vi "Main.vi"() -> ()   [LabVIEW 2024]
doc: "Main Program initialize config files, handles user inputs, image acquisition, object detection and image storing. User interface is handled in a state machine sending outputs."
uses:
  controls/Data_JKI.ctl
  <vilib>/userDefined/High Color/IMAQdx.ctl
  <vilib>/vision/Image Controls.llb/IMAQ Image.ctl
  CAM_ID.ctl
  <vilib>/vision/driver/IMAQdx.llb/IMAQdx Camera Control Mode.ctl
  <vilib>/addons/_JKI Toolkits/State Machine/_JKI_lib_State_Machine.llb/Select State(s)_bool__jki_lib_state_machine.vi
  <vilib>/addons/_JKI Toolkits/State Machine/_JKI_lib_State_Machine.llb/Select State(s)_err__jki_lib_state_machine.vi
  5a594196-7142-418f-9656-114c0d668309.vi
  bb2d0c64-4a32-4bc2-b703-4003a0b41c3e.vi
  382dfe38-6e62-4a8f-90ef-71572aba4852.vi
  03aece60-1779-4009-a170-6ff07e738b5d.vi
  84b06488-54b1-401d-9401-24ea6e13162c.vi
  8324a88f-2dce-41de-b56a-eb000cd9b6a9.vi
  af50b9d5-4c90-4cd4-8bfe-74b4777be0cf.vi
  75fb93f5-a9aa-4c6b-93c7-07fbec5219cd.vi
  9cdd72f1-8236-455d-ab5e-5837bd52b41e.vi
  99c214c5-2fde-429c-805f-c7e6bab6585a.vi
  c28b30e7-2201-423e-8025-b3bde2d8c85a.vi
  557f3c17-7900-4f14-af8c-d1828dceced0.vi
  f995d3e5-f405-4ab5-a577-27e0de2fc963.vi
  fac71c25-9fc9-4a64-ae82-7863fefb1b13.vi
  4f10c793-c4d5-419f-bcb1-2d0c9d14968a.vi
  05f65ac7-837b-4982-8062-8738a5ade4f2.vi
  3f6d6c7d-6f0a-4ecb-ada9-c2a4a5f01e8e.vi
  <extravilib>/ChannelInstances/Tag-t'Data_JKI.ctl'/Read With Abort.vi
  <extravilib>/ChannelInstances/Tag-c(bool,bool)/Write With Abort.vi
  <extravilib>/ChannelInstances/Tag-c(bool,bool)/Read With Abort.vi
  <extravilib>/ChannelInstances/Tag-t'Data_JKI.ctl'/Write With Abort.vi
  <extravilib>/ChannelInstances/Tag-t'Data_JKI.ctl'/Instantiate.vi
  <extravilib>/ChannelInstances/Tag-t'Data_JKI.ctl'/EndpointRead.vi
  <vilib>/addons/_JKI Toolkits/State Machine/_JKI_lib_State_Machine.llb/Periodic Trigger__ogtk__JKI-SM__jki_lib_state_machine.vi
  <vilib>/Utility/xml.llb/Read From XML File(string).vi
  <vilib>/Utility/xml.llb/Write to XML File(string).vi
  <extravilib>/ChannelInstances/Tag-t'Data_JKI.ctl'/Endpoint.vi
  <extravilib>/ChannelInstances/Tag-c(bool,bool)/Instantiate.vi
  <extravilib>/ChannelInstances/Tag-c(bool,bool)/EndpointRead.vi
  <extravilib>/ChannelInstances/Tag-c(bool,bool)/Endpoint.vi
  <vilib>/regexp/Match Regular Expression.xnode
  <extravilib>/ChannelInstances/Tag-c(bool,bool).lvlib
  <vilib>/vision/driver/NI_Vision_Acquisition_Software.lvlib
  <extravilib>/ChannelInstances/Tag-t'Data_JKI.ctl'.lvlib
panel:
  out "Phase 3":bool
  out "Valve":bool
  out "Pump":bool
  out "Cam 1":bool
  out "Cam 2":bool
  out "Status":string
  in  "Auto Flush":bool
  in  "Empty and Refill":bool
  in  "Close and Refill":bool
  out "read buffer 2":string
  out "System Version":string="SRS Software - Version 0.0.0.1-beta"
  in  "Other notes":string caption="Sample Name"
  in  "Species Name":string="Test Sample" caption="Sample Name"
  out "Ready":bool=TRUE
  in  "Operator":string="JFR" caption="Sample Name"
  out "Active":bool
  in  "Start Image Capture":bool
  in  "Sample Name":string="#00000"
  in  "Stop Image Capture":bool
  out "Overlay_tab":T1(tab)=enum."Phase3"
  in  "Overload threshold":i32=50 min=1
  in  "Img Save Que Size":i32=100 caption="Save Buffer Size" min=1
  in  "Img Proc Que Size":i32=200 caption="Process Buffer Sze" min=1
  in  "Reconnect Cams":bool
  in  "Reconnect Arduino mega":bool
  in  "Reconnect Pump":bool
  in  "Reconnect Arduino Uno":bool
  in  "Connect Systems":bool
  out "Cam1_Stats":cluster{"Mean_Area":i32, "Img_Count":u32} caption="Camera 1"
  out "Cam2_Stats":cluster{"Mean_Area":i32, "Img_Count":u32} caption="Camera 2"
  out "Sample Number":string="#0000" caption="Sample Name"
  out "Container barcode":string
  out "Container num. Out":i32
  out "Individual processed":bool
  in  "Collection Date":timestamp=timestamp(2713993200 s since 1904-01-01) format="%<%x>T"
  in  "Station":string="Station..." caption="Sample Name"
  in  "Location":string="Location..." caption="Sample Name"
  in  "Latitude":string="56.149375" caption="Sample Name"
  in  "Longitude":string="10.212404" caption="Sample Name"
  in  "Determiner":string="Name..." caption="Sample Name"
  in  "Sex":string="NaN" caption="Sample Name"
  in  "LegCamAtt":bool caption="Legacy Camera Attributes"
  in  "Change Crop":bool
  in  "DetectCrop":dbl=30.0 caption="Movement Detection size" format="%#_g %"
  in  "Sample size threshold":i32=500 min=1
  in  "New Sample timeout":i32=20 min=1
  in  "Calibration Pictures":bool
  out "Target framerate":i32=5 caption="Target FPS"
  in  "Max Framerate":i32=5 caption="Max FPS" min=1
  in  "Exposure Time":dbl=2000.0
  in  "Exposure":enum32{"Item 0", "Item 1", "Item 2", "Item 3"}(radio)=enum."Item 3"
  in  "Aperture":enum32{"Item 0", "Item 1", "Item 2", "Item 3"}(radio)=enum."Item 2"
  in  "I":i32(slide)=1 min=1 max=9 step=1 scale=1.0..9.0
  in  "A":dbl(slide) min=0.0 max=6000.0 step=100.0 scale=0.0..6000.0
  in  "Send CMD":bool
  in  "Pump Cycle":bool
  in  "Manual Open":bool
  in  "Open & Close":bool
  in  "Manual Close":bool
  out "Current Position":string
  in  "Position":bool
  in  "Apply sorting val":bool
  in  "Initial size":dbl min=0.0
  in  "Num. of containers":dbl=30.0 min=1.0 max=30.0
  in  "Size Interval":dbl=100.0 min=1.0
  in  "Sorting sys.":bool
  in  "Clear Error":bool
  in  "Rescan barcodes":bool
  in  "Send Barcode":bool
  in  "Return Home":bool
  in  "Get Barcode list":bool
  in  "Get Status":bool
  in  "Container nr.":dbl=30.0 min=1.0 max=30.0
  out "Process buffer":T2(graph)
  out "Save buffer":T2(graph)
  out "Framerate":i32 caption="Current Framerate"
  out "Status History":string
  in  "Save History":bool
  in  "Overlay_Ring":u16(ring)=5 items=["System", "Session Data", "Extended Setup", "Camera", "Dispenser", "Phase3", "Stats", "History"]
  in  "Exit":bool
  out "Camera 1":T3(plugin-control)
  out "Camera 2":T3(plugin-control)
  out "Camera 1 Binary":T3(plugin-control)
  out "Camera 2 Binary":T3(plugin-control)
  out "Camera 1 Detect":T3(plugin-control)
  out "Camera 2 Detect":T3(plugin-control)
  # "Connections"
  # "Description:\nData from the last sample for each camera.\n\nMean area\nMean area  from detection algorithm.\n\nImages\nTotal number of images saved."
  # "Barcode and container"
  # "Detection settings"
  # "Camera/Lens settings"
  # "Pump Control"
  # "Hatch Control"
  # "A0-6000 Plunger position\nI1-9 Valve port [CW]"
  # "Automatic Functions"
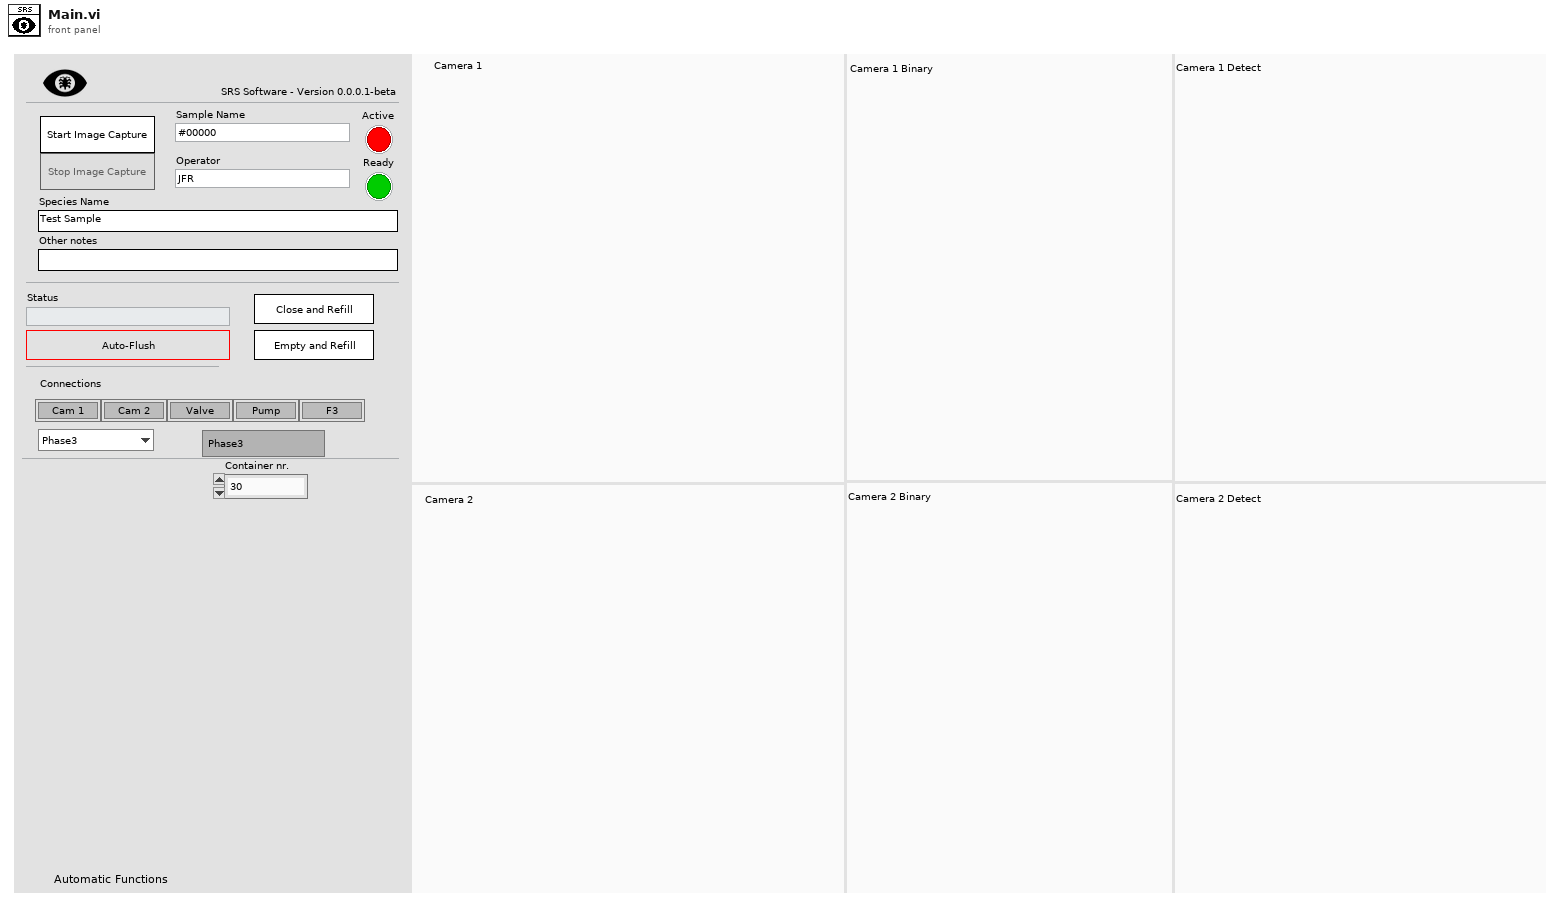
[diagram p1: front panel]
types:
  T1 = enum32{"System", "Session Data", "Extended Setup", "Camera", "Dispenser", "Phase3", "Stats", "History"}
  T2 = cluster{"# elements in queue":i32, "# elements in queue":i32}
  T3 = typedef "IMAQ Image.ctl" = refnum<image>
  T4 = typedef "Data_JKI.ctl" = cluster{"Camera 1":cluster{"Camera1":T5, "Cam 1":bool, "CAM1 Model":enum16{"a2A5328-15ucBAS", "acA1920-155uc"}, "Cam1 ID":i32}, "Camera 2":cluster{"Camera2":T5, "Cam 2":bool, "CAM2 Model":enum16{"a2A5328-15ucBAS", "acA1920-155uc"}, "Cam2 ID":i32}, "Image":cluster{"Camera1_Img":T3, "Camera2_Img":T3, "Img1_Orig_Disp":T3, "Img2_Orig_Disp":T3, "Img1_Orig_RGB":T3, "Img2_Orig_RGB":T3, "Blue_Plane_Extract":T3, "Subtracted_Plane":T3, "Img1_Binary":T3, "Img2_Binary":T3, "Crop_Mask":T3, "Img1_Save":T3, "Img2_Save":T3, "Img1_Cali_Full":T3, "Img2_Cali_Full":T3, "Img1_Cali_Detect":T3, "Img2_Cali_Detect":T3}, "Ques":cluster{"Cam 1 queue":refnum<queue>, "Cam 2 queue":refnum<queue>, "Cam 1 - save queue":refnum<queue>, "Cam 2 - save queue":refnum<queue>, "Image Process Queue Size":i32, "Image Save Queue Size":i32, "Overload threshold":i32, "Max large object threshold":i32}, "Arduino SRS":cluster{"Pinch-valve":refnum<visa-resource-name>, "Actuator":bool, "Arduino Uno":string, "Valve state":enum16{"Standby", "Close", "Open"}}, "Pump":cluster{"Port":refnum<visa-resource-name>, "Connection":bool, "Flush Size":i32, "Command":string, "Pump Size":enum16{"None", "Small", "Large"}, "Pump":string, "Ready":bool}, "Camera settings":cluster{"Detection settings":cluster{"Sample size threshold":i32, "Detection Region %":dbl, "Timeout Sample":i32}, "Lens/camera settings":cluster{"Aperture":enum32{"Item 0", "Item 1", "Item 2", "Item 3"}, "Legacy Cam Attributes":bool, "Max Framerate":i32, "Exposure Time":dbl, "Framerate":i32}, "Crop settings":cluster{"Cam1":cluster{"Rectangle 1":T6, "Camera Orientation 1":string, "Pixel to mm 1":dbl}, "Cam2":cluster{"Rectangle 2":T6, "Camera Orientation 2":string, "Pixel to mm 2":dbl}}}, "Arduino ISS":cluster{"Mega F3":refnum<visa-resource-name>, "Phase3":bool, "Barcode":string, "Sorting sys.":bool, "Initial size":dbl, "Size Interval":dbl, "Mun. of containers":dbl, "Container nr.":dbl, "Arduino Mega":string, "Attempts":dbl}, "Img_Capt":bool, "Empty_Refill":bool, "I don't think is in use":cluster{"Light intensity":i32}, "Extended setup":cluster{"Location":string, "Latitude":string, "Longitude":string, "Determiner":string, "Sex":string, "Station":string, "Collection date":string}, "Main interface":cluster{"Sample Name":string, "Operator":string, "Species Name":string, "Other Notes":string}, "Tap1":u16, "SystemVersion":u16, "System Serial":string, "Exit":bool, "Kuvette Full":bool, "Core JKI":cluster{"Current VI Reference":refnum<vi>, "Close Panel on Exit?":bool}, "Calibration":cluster{"Calibration 1":path, "Calibration 2":path, "Detect 1":path, "Detect 2":path}, "Auto Flush":bool, "Status History":string, "Timestamp Start":string}
  T5 = typedef "IMAQdx.ctl" = refnum<k21>
  T6 = typedef "IMAQ Rectangle" = cluster{"Left":i32, "Top":i32, "Right":i32, "Bottom":i32, "Rotation":dbl}
  T7 = enum8{"Enabled", "Disabled", "Disabled and Grayed Out"}
  T8 = enum32{"Invalid", "Standard", "Closed", "Hidden", "Minimized", "Maximized"}
  T9 = enum32{"invalid app kind", "Development System", "Run Time System", "Student Edition", "Embedded LabVIEW", "Evaluation", "Custom"}
  T10 = typedef "CAM_ID.ctl" = cluster{"CAM_ID1":i32, "CAM_ID2":i32}
  T11 = enum16{"open", "replace", "create", "open or create", "replace or create", "replace or create with confirmation"}
  T12 = cluster{"Current VI Reference":refnum<vi>, "Close Panel on Exit?":bool}
  T13 = cluster{"# elements in queue":i32, "# elements in queue":i32}[]
  T14 = enum16{"Left Button", "Center Button", "Right Button", "Window Close"}
  T15 = typedef "NI_Vision_Acquisition_Software.lvlib/IMAQdx Camera Control Mode.ctl" = enum32{"Controller", "Listener"}
  T16 = typedef "Tag-t'Data_JKI.ctl'.lvlib/))Channel.ctl" = refnum<queue>
  T17 = typedef "Tag-c(bool,bool).lvlib/))Channel.ctl" = refnum<queue>
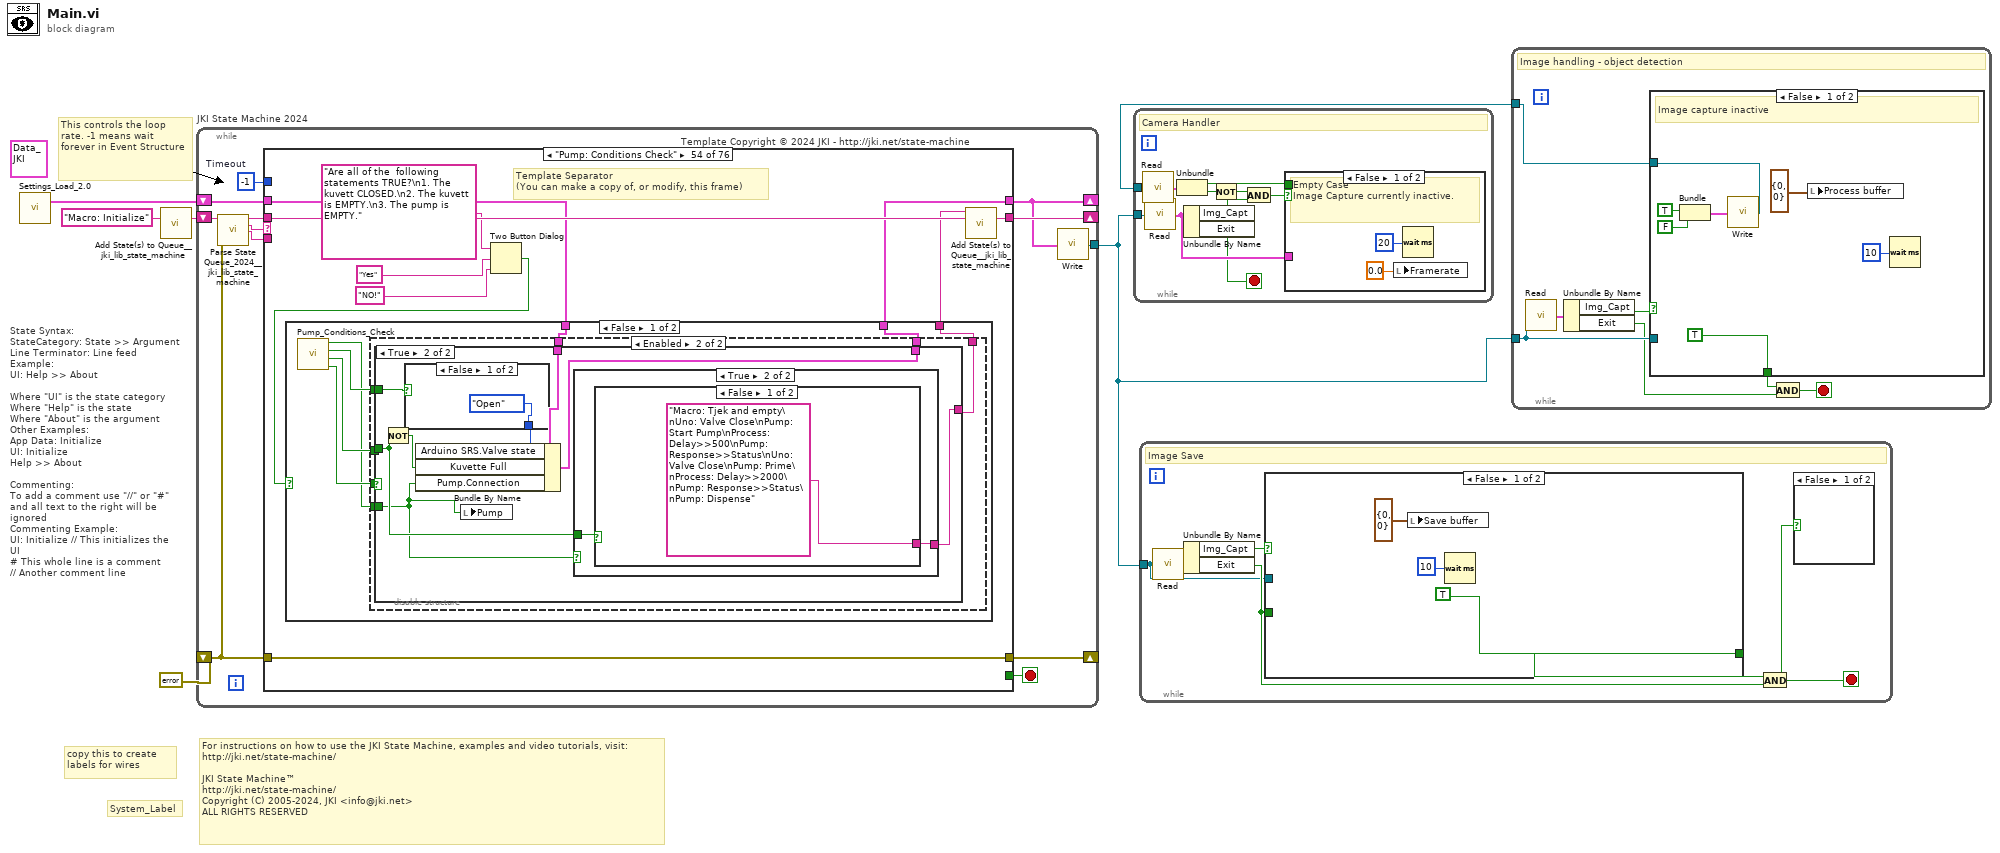
[diagram p0: block diagram]
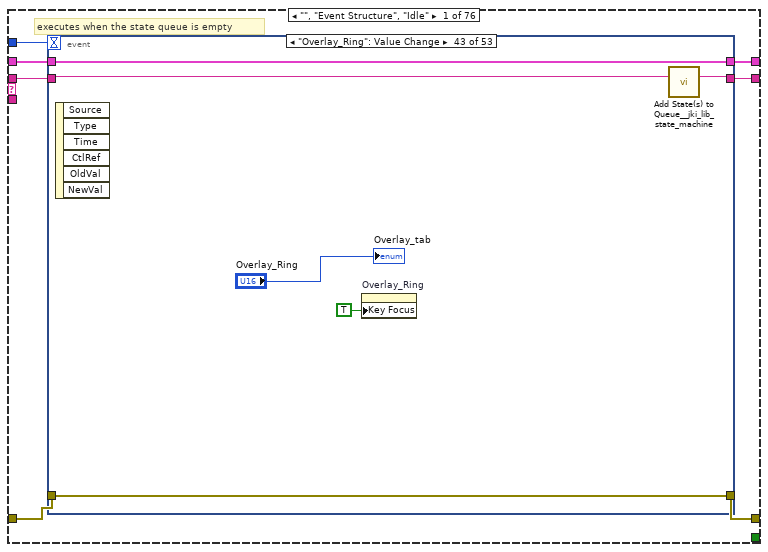
[diagram p2: hidden frame]
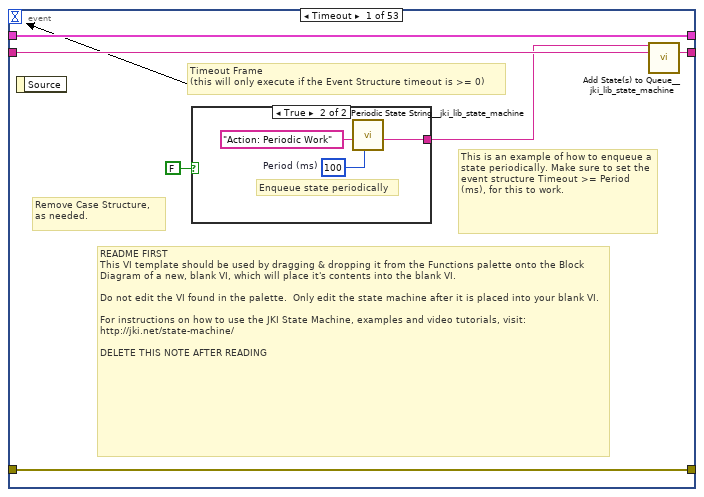
[diagram p3: hidden frame]
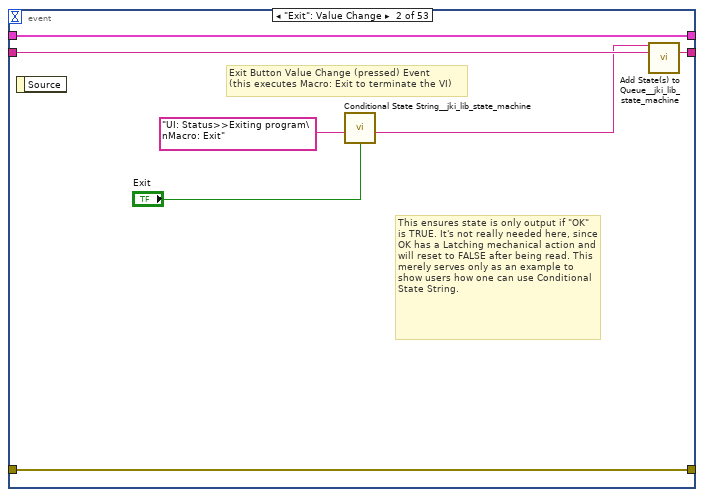
[diagram p5: hidden frame]
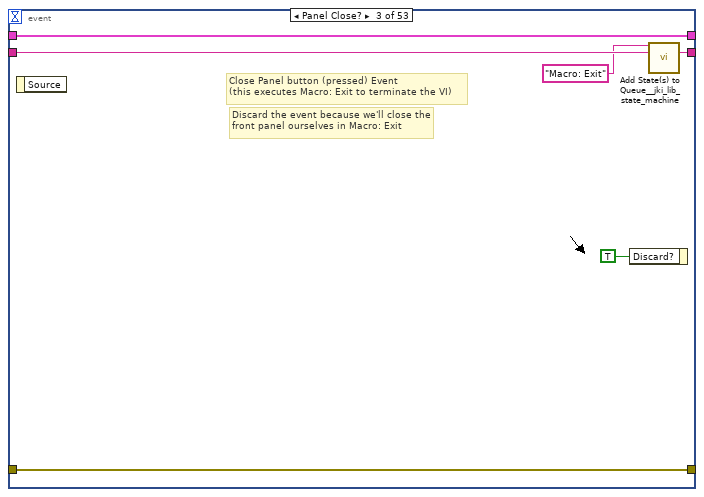
[diagram p6: hidden frame]
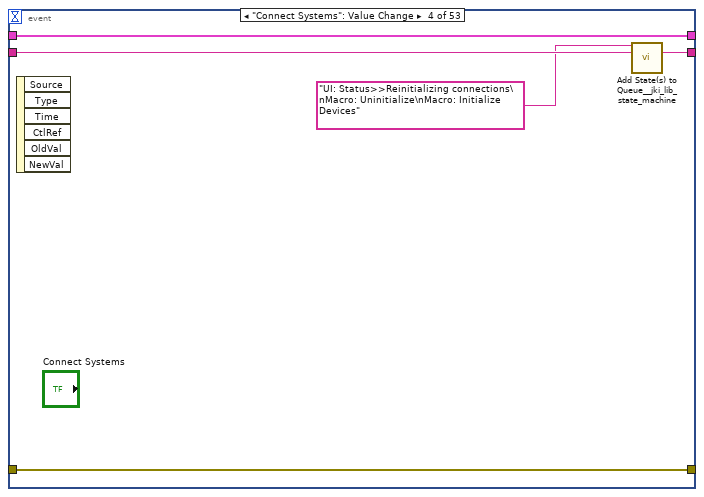
[diagram p7: hidden frame]
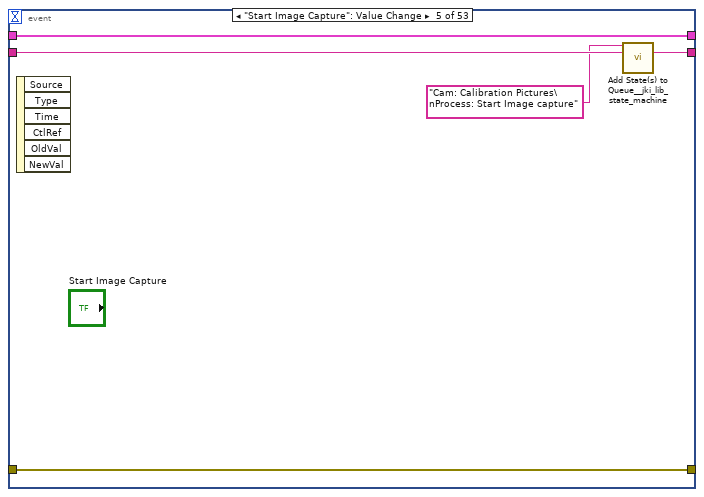
[diagram p8: hidden frame]
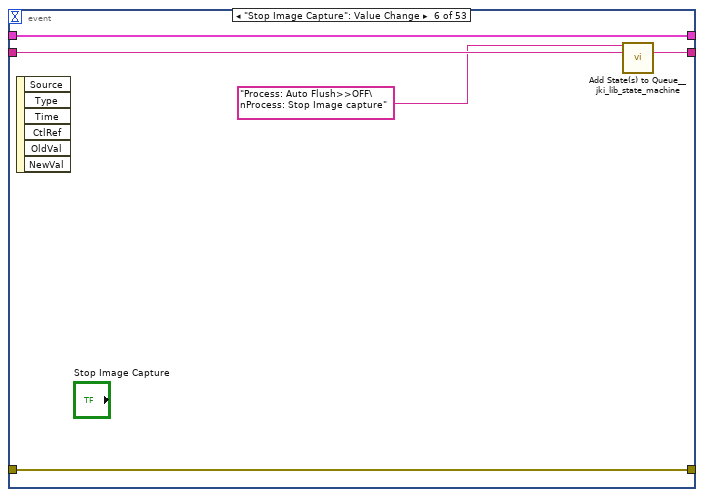
[diagram p9: hidden frame]
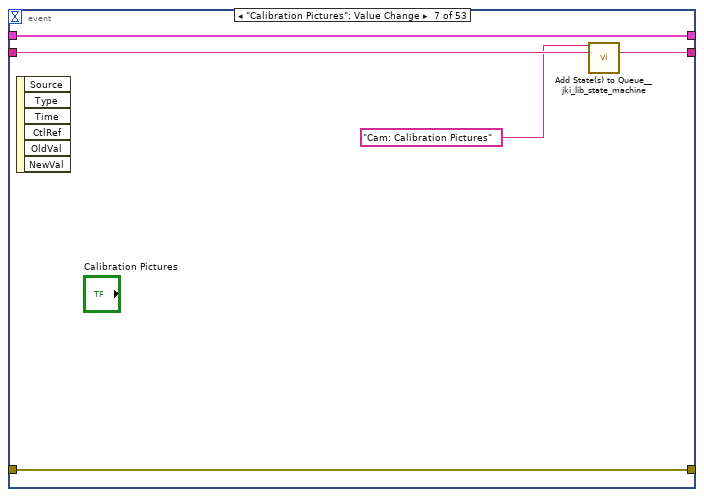
[diagram p10: hidden frame]
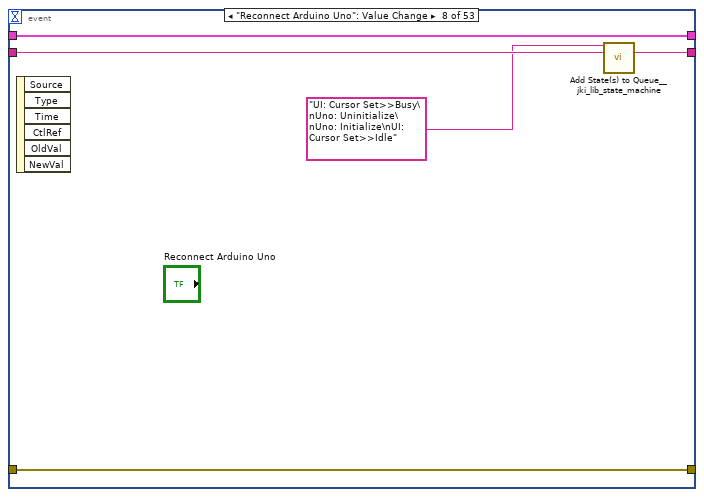
[diagram p11: hidden frame]
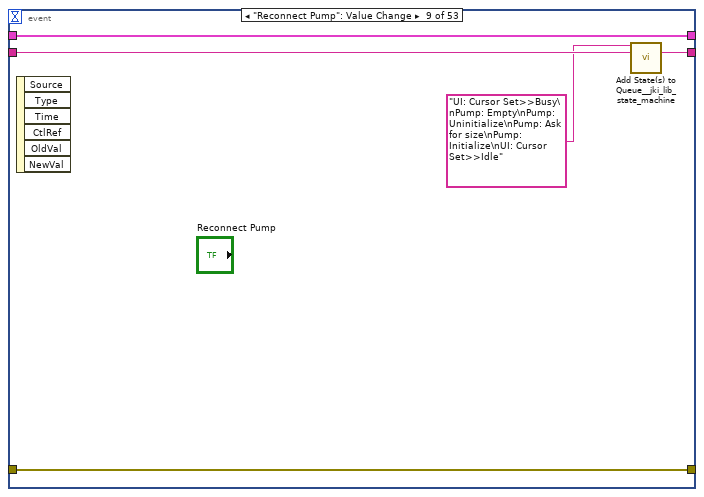
[diagram p12: hidden frame]
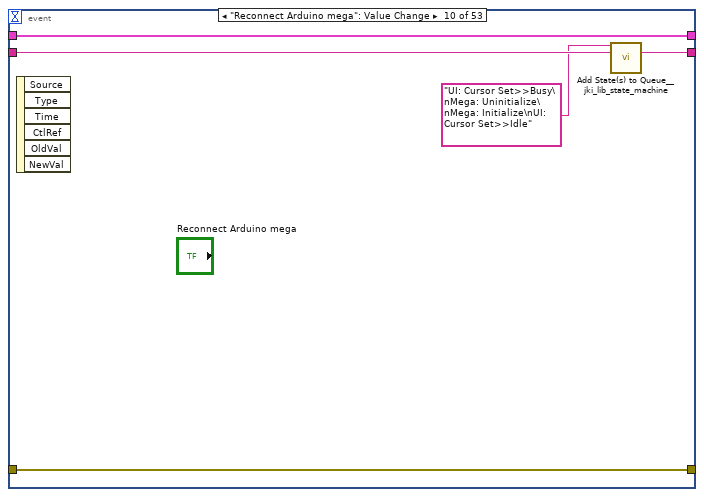
[diagram p13: hidden frame]
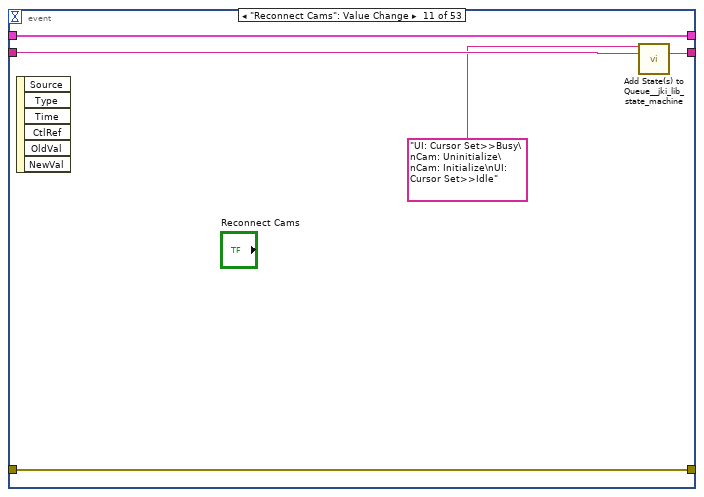
[diagram p14: hidden frame]
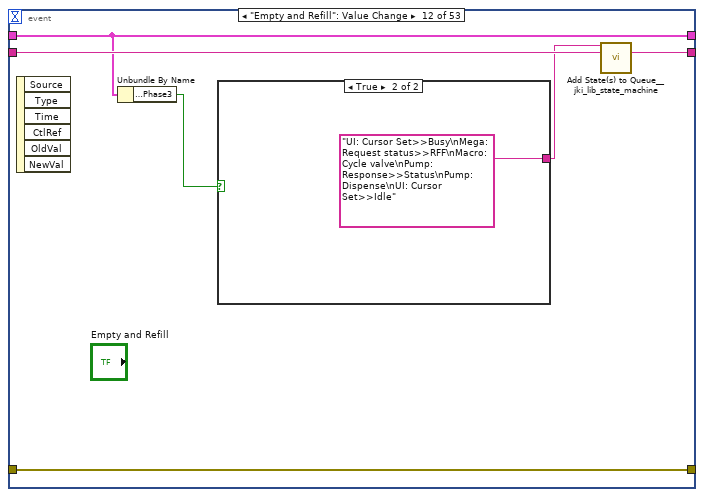
[diagram p15: hidden frame]
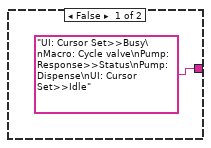
[diagram p16: hidden frame]
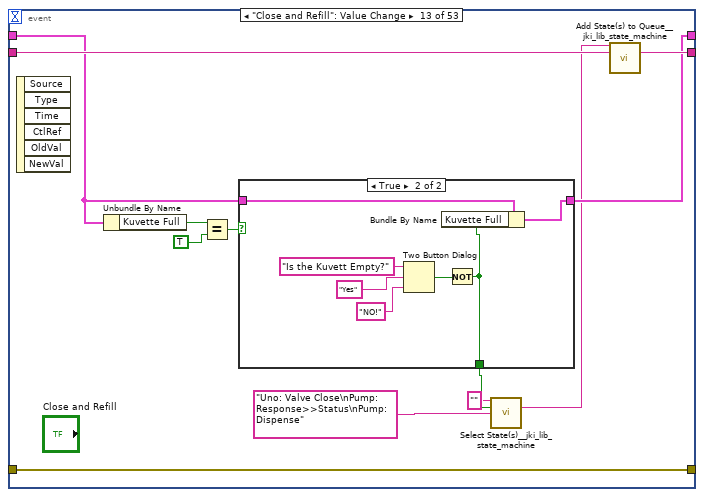
[diagram p17: hidden frame]
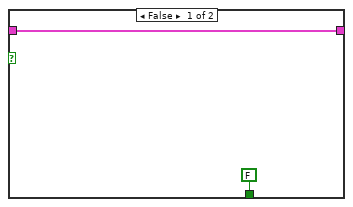
[diagram p18: hidden frame]
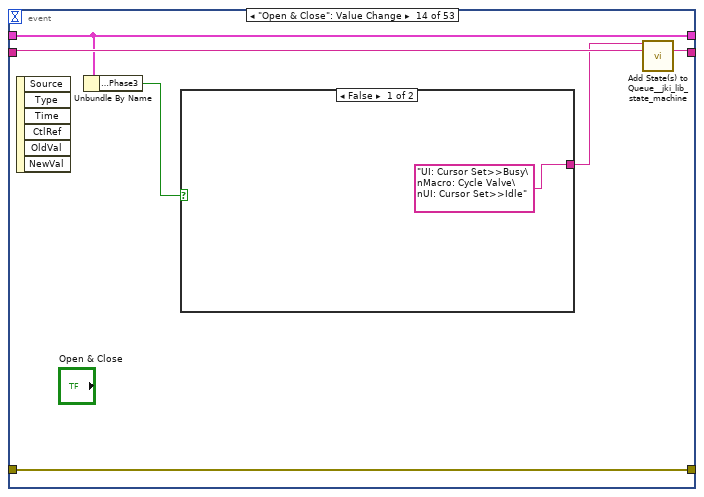
[diagram p19: hidden frame]
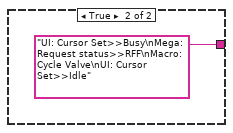
[diagram p20: hidden frame]
diagram:
  (unwired) T4 {"Camera 1"={"Camera1"="", "Cam 1"=FALSE, "CAM1 Model"=enum."a2A5328-15ucBAS", "Cam1 ID"=0}, "Camera 2"={"Camera2"="", "Cam 2"=FALSE, "CAM2 Model"=enum."a2A5328-15ucBAS", "Cam2 ID"=0}, "Image"={"Camera1_Img"=refnum, "Camera2_Img"=refnum, "Img1_Orig_Disp"=refnum, "Img2_Orig_Disp"=refnum, "Img1_Orig_RGB"=refnum, "Img2_Orig_RGB"=refnum, "Blue_Plane_Extract"=refnum, "Subtracted_Plane"=refnum, "Img1_Binary"=refnum, "Img2_Binary"=refnum, "Crop_Mask"=refnum, "Img1_Save"=refnum, "Img2_Save"=refnum, "Img1_Cali_Full"=refnum, "Img2_Cali_Full"=refnum, "Img1_Cali_Detect"=refnum, "Img2_Cali_Detect"=refnum}, "Ques"={"Cam 1 queue"=refnum, "Cam 2 queue"=refnum, "Cam 1 - save queue"=refnum, "Cam 2 - save queue"=refnum, "Image Process Queue Size"=0, "Image Save Queue Size"=0, "Overload threshold"=0, "Max large object threshold"=0}, "Arduino SRS"={"Pinch-valve"="", "Actuator"=FALSE, "Arduino Uno"="", "Valve state"=enum."Standby"}, "Pump"={"Port"="", "Connection"=FALSE, "Flush Size"=0, "Command"="", "Pump Size"=enum."None", "Pump"="", "Ready"=FALSE}, "Camera settings"={"Detection settings"={"Sample size threshold"=0, "Detection Region %"=0.0, "Timeout Sample"=0}, "Lens/camera settings"={"Aperture"=enum."Item 0", "Legacy Cam Attributes"=FALSE, "Max Framerate"=0, "Exposure Time"=0.0, "Framerate"=0}, "Crop settings"={"Cam1"={"Rectangle 1"={"Left"=0, "Top"=0, "Right"=0, "Bottom"=0, "Rotation"=0.0}, "Camera Orientation 1"="", "Pixel to mm 1"=0.0}, "Cam2"={"Rectangle 2"={"Left"=0, "Top"=0, "Right"=0, "Bottom"=0, "Rotation"=0.0}, "Camera Orientation 2"="", "Pixel to mm 2"=0.0}}}, "Arduino ISS"={"Mega F3"="", "Phase3"=FALSE, "Barcode"="", "Sorting sys."=FALSE, "Initial size"=0.0, "Size Interval"=0.0, "Mun. of containers"=0.0, "Container nr."=0.0, "Arduino Mega"="", "Attempts"=0.0}, "Img_Capt"=FALSE, "Empty_Refill"=FALSE, "I don't think is in use"={"Light intensity"=0}, "Extended setup"={"Location"="", "Latitude"="", "Longitude"="", "Determiner"="", "Sex"="", "Station"="", "Collection date"=""}, "Main interface"={"Sample Name"="", "Operator"="", "Species Name"="", "Other Notes"=""}, "Tap1"=0, "SystemVersion"=0, "System Serial"="", "Exit"=FALSE, "Kuvette Full"=FALSE, "Core JKI"={"Current VI Reference"=refnum, "Close Panel on Exit?"=FALSE}, "Calibration"={"Calibration 1"=path "", "Calibration 2"=path "", "Detect 1"=path "", "Detect 2"=path ""}, "Auto Flush"=FALSE, "Status History"="", "Timestamp Start"=""}
  # "For instructions on how to use the JKI State Machine, examples and video tutorials, visit:\nhttp://jki.net/state-machine/\n\nJKI State Machine™\nhttp://jki.net/state-machine/\nCopyright (C) 2005-2024, JKI <info@jki.net>\nALL RIGHTS RESERVED"
  # "State Syntax:\nStateCategory: State >> Argument\nLine Terminator: Line feed\nExample:\nUI: Help >> About\n\nWhere \"UI\" is the state category\nWhere \"Help\" is the state\nWhere \"About\" is the argument\nOther Examples:\nApp Data: Initialize\nUI: Initialize\nHelp >> About\n\nCommenting:\nTo add a comment use \"//\" or \"#\" and all text to the right will be ignored\nCommenting Example:\nUI: Initialize // This initializes the UI\n# This whole line is a comment\n// Another comment line"
  # "copy this to create labels for wires"
  # "This controls the loop rate. -1 means wait forever in Event Structure"
  # "System_Label"
  n1 = call "Settings_Load_2.0.vi"() -> ("Data"=w3:T4)  [unwired: 3 in, 1 out]
  n2 = call <vilib>:"Add State(s) to Queue__jki_lib_state_machine.vi"("State(s) in (\"\")"="Macro: Initialize") -> ("States Out"=w5:string)  [unwired: 14 in]
  n3 = while "JKI State Machine 2024" {
    shift-right: [w7] -> _
    shift-left: w3 -> [w8]
    shift-right: [w14] -> _
    shift-left: errorcluster {"status"=FALSE, "code"=0, "source"=""} ("error constant") -> [w10]
    shift-right: [w13] -> _
    shift-left: w5 -> [w15]
    tunnel: [w9] -> w1
    stop <- w12 stop-if-true
    w11 = -1  # Timeout
    # "Template Copyright © 2024 JKI - http://jki.net/state-machine"
    n4 = call <vilib>:"Parse State Queue_2024__jki_lib_state_machine.vi"("State Queue"=w15, "Error In (no error)"=w10) -> ("Remaining States"=w17:string, "Current State"=w18:string, "Arguments"=w16:string)  [unwired: 11 in]
    n5 = case shown="\"Pump: Conditions Check\"" w18 {
      selector: w18 -> [_ _ w464 _ _ _ _ _ _ _ _ _ _ _ _ _ _ _ _ _ _ _ _ _ _ _ _ _ _ _ _ _ _ _ _ _ _ _ _ _ _ _ _ _ _ _ _ _ _ _ _ _ _ _ _ _ _ _ _ _ _ _ _ _ _ _ _ _ _ _ _ _ _ _ _ _]
      tunnel: w17 -> [w25 w463 w468 w487 w497 w508 w512 w518 w537 w563 w575 w581 w585 w602 w629 w634 w639 w654 w662 w667 w673 w684 w753 w758 w763 w768 w773 w778 w785 w801 w805 w815 w850 w874 w884 w892 w899 w904 w923 w927 w935 w942 w983 w1009 w1031 w1039 w1197 w1227 w1257 w1289 w1312 w1323 w1336 w1350 w1424 w1482 w1499 w1531 w1555 w1568 w1613 w1635 w1648 w1655 w1726 w1728 w1779 w1812 w1832 w1849 w1867 w1890 w1906 w1936 w1977 w1989]
      tunnel: w16 -> [_ _ _ _ w492 _ _ _ _ _ _ _ _ _ _ _ _ w644 w657 _ w668 w678 _ _ _ _ _ _ _ _ _ _ _ _ w879 _ w894 _ _ _ _ w938 _ _ _ _ _ _ _ w1281 _ _ _ _ _ _ _ _ _ w1574 _ _ _ _ _ w1727 _ w1797 _ _ w1859 _ _ _ _ _]
      tunnel: w8 -> [w23 w460 w466 w480 w494 w503 w509 w515 w521 w553 w565 w577 w582 w593 w625 w631 w636 w641 w659 w665 w671 w680 w750 w755 w760 w765 w770 w775 w781 w792 w802 w810 w840 w871 w881 w889 w897 w901 w917 w924 w933 w944 w978 w1004 w1029 w1036 w1195 w1225 w1253 w1283 w1309 w1321 w1333 w1343 w1418 w1475 w1500 w1530 w1548 w1573 w1607 w1632 w1645 w1653 w1724 w1736 w1775 w1801 w1829 w1845 w1861 w1887 w1904 w1942 w1975 w1983]
      tunnel: [w22 w461 w470 w484 errorcluster {"status"=FALSE, "code"=0, "source"=""} ("error out") w506 w510 w516 w524 w549 w567 w578 w583 w600 w627 w632 w637 w652 w660 w664 w669 w681 w751 w756 w761 w766 w771 w776 w783 w798 w803 w813 w837 w872 w882 w890 w895 w902 w914 w925 w931 w945 w979 w1005 w1027 w1032 w1191 w1221 w1254 w1284 w1310 w1319 w1334 w1348 w1421 w1477 w1501 w1532 w1552 w1577 w1608 w1633 w1640 w1651 w1721 w1738 w1774 w1802 w1827 w1844 w1864 w1888 w1891 w1937 w1972 w1978] -> w14
      tunnel: w10 -> [w19 w461 w469 w484 w493 w506 w510 w516 w523 w550 w566 w579 w583 w600 w627 w632 w637 w652 w660 w664 w670 w682 w751 w756 w761 w766 w771 w776 w783 w798 w803 w812 w843 w872 w882 w890 w896 w902 w905 w925 w930 w946 w980 w1006 w1028 w1033 w1192 w1222 w1255 w1285 w1310 w1318 w1334 w1348 w1422 w1478 w1503 w1534 w1553 w1575 w1609 w1633 w1646 w1652 w1723 w1739 w1776 w1803 w1828 w1846 w1865 w1888 w1903 w1938 w1973 w1980]
      tunnel: [w24 w462 w467 w486 w496 w507 w511 w517 w536 w562 w574 w580 w584 w601 w628 w633 w638 w653 w661 w666 w672 w683 w752 w757 w762 w767 w772 w777 w784 w800 w804 w814 w849 w873 w883 w891 w898 w903 w922 w926 w934 w948 w982 w1008 w1030 w1038 w1196 w1226 w1256 w1288 w1311 w1322 w1335 w1349 w1423 w1481 w1497 w1528 w1554 w1578 w1612 w1634 w1647 w1654 w1725 w1734 w1778 w1811 w1831 w1848 w1866 w1889 w1905 w1944 w1976 w1988] -> w13
      tunnel: [_ _ _ _ _ TRUE _ _ _ _ _ _ _ _ _ _ _ _ _ _ _ _ _ _ _ _ _ _ _ _ _ _ _ _ _ _ _ _ _ _ _ _ _ _ _ _ _ _ _ _ _ _ _ _ _ _ _ _ _ _ _ _ _ _ _ _ _ _ _ _ _ _ _ _ _ _] -> w12
      tunnel: [w21 w460 w466 w485 w494 w502 w509 w513 w520 w553 w565 w577 w582 w592 w625 w631 w636 w649 w659 w665 w671 w680 w750 w755 w760 w765 w770 w775 w781 w792 w802 w811 w841 w870 w880 w888 w897 w901 w917 w924 w932 w947 w977 w1003 w1026 w1035 w1195 w1225 w1253 w1282 w1309 w1320 w1332 w1342 w1417 w1474 w1502 w1533 w1547 w1572 w1606 w1632 w1639 w1653 w1722 w1730 w1775 w1801 w1829 w1845 w1860 w1887 w1896 w1943 w1974 w1981] -> w7
      tunnel: w11 -> [w20 _ _ _ _ _ _ _ _ _ _ _ _ _ _ _ _ _ _ _ _ _ _ _ _ _ _ _ _ _ _ _ _ _ _ _ _ _ _ _ _ _ _ _ _ _ _ _ _ _ _ _ _ _ _ _ _ _ _ _ _ _ _ _ _ _ _ _ _ _ _ _ _ _ _ _]
      frame "", "Event Structure", "Idle" {
        # "executes when the state queue is empty"
        n6 = event shown="[42] \"Overlay_Ring\": Value Change" {
          selector: _ -> [_ _ _ _ _ _ _ _ _ _ _ _ _ _ _ _ _ _ _ _ _ _ _ _ _ _ _ _ _ _ _ _ _ _ _ _ _ _ _ _ _ _ _ _ _ _ _ _ _ _ _ _ _]
          dyn-events: _ -> [_ _ _ _ _ _ _ _ _ _ _ _ _ _ _ _ _ _ _ _ _ _ _ _ _ _ _ _ _ _ _ _ _ _ _ _ _ _ _ _ _ _ _ _ _ _ _ _ _ _ _ _ _]
          timeout: w20 -> [_ _ _ _ _ _ _ _ _ _ _ _ _ _ _ _ _ _ _ _ _ _ _ _ _ _ _ _ _ _ _ _ _ _ _ _ _ _ _ _ _ _ _ _ _ _ _ _ _ _ _ _ _]
          tunnel: w25 -> [w31 w41 w47 w50 w55 w61 w65 w71 w74 w79 w85 w91 w105 w121 w128 w134 w143 w158 w173 w225 w231 w237 w243 w250 w256 w263 w268 w274 w277 w286 w293 w299 w307 w326 w337 w343 w349 w361 w367 w373 w379 w384 w388 w398 w403 w408 w412 w422 w426 w431 w438 w452 w458]
          tunnel: [w30 w40 w46 w51 w56 w62 w66 w70 w75 w80 w84 w92 w106 w122 w129 w135 w144 w159 w174 w226 w232 w238 w244 w251 w257 w264 w269 w275 w281 w287 w294 w300 w308 w327 w338 w344 w350 w362 w368 w374 w380 w385 w389 w399 w404 w409 w413 w423 w427 w432 w439 w453 w457] -> w24
          tunnel: w23 -> [w28 w38 w44 w52 w53 w58 w64 w69 w76 w81 w86 w89 w101 w118 w126 w136 w142 w154 w178 w224 w230 w236 w242 w249 w255 w262 w267 w273 w279 w285 w292 w298 w305 w325 w336 w342 w348 w359 w366 w372 w378 w383 w387 w395 w405 w410 w415 w421 w428 w433 w437 w450 w456]
          tunnel: [w29 w39 w45 w49 w57 w59 w67 w72 w77 w82 w87 w93 w107 w120 w130 w137 w145 w160 w170 w227 w233 w239 w245 w252 w258 w260 w270 w276 w282 w288 w289 w301 w315 w328 w339 w345 w351 w363 w369 w375 w381 w386 w390 w400 w402 w406 w414 w424 w429 w434 w440 w454 w459] -> w22
          tunnel: w19 -> [w29 w39 w45 w49 w57 w59 w67 w72 w77 w82 w87 w93 w107 w120 w130 w137 w145 w160 w170 w227 w233 w239 w245 w252 w258 w260 w270 w276 w282 w288 w289 w301 w315 w328 w339 w345 w351 w363 w369 w375 w381 w386 w390 w400 w402 w406 w414 w424 w429 w434 w440 w454 w459]
          tunnel: [w28 w38 w44 w52 w53 w58 w64 w69 w76 w81 w86 w89 w100 w118 w126 w136 w142 w153 w176 w223 w229 w235 w241 w248 w254 w261 w266 w272 w280 w284 w291 w295 w302 w323 w335 w341 w347 w360 w365 w371 w377 w383 w387 w395 w405 w410 w415 w420 w428 w433 w436 w451 w456] -> w21
          event Timeout {
            # "Remove Case Structure, as needed."
            # "This is an example of how to enqueue a state periodically. Make sure to set the event structure Timeout >= Period (ms), for this to work."
            # "README FIRST\nThis VI template should be used by dragging & dropping it from the Functions palette onto the Block Diagram of a new, blank VI, which will place it's contents into the blank VI.\n\nDo not edit the VI found in the palette.  Only edit the state machine after it is placed into your blank VI.\n\nFor instructions on how to use the JKI State Machine, examples and video tutorials, visit:\nhttp://jki.net/state-machine/\n\nDELETE THIS NOTE AFTER READING"
            # "Timeout Frame\n(this will only execute if the Event Structure timeout is >= 0)"
            n7 = event-data() -> ()  [unwired: 1 in, 1 out]
            n8 = case shown="True" FALSE {
              tunnel: [_ w34] -> w27
              frame False {
              }
              frame True {
                w32 = u32 100  # Period (ms)
                # "Enqueue state periodically"
                n9 = call <vilib>:"Periodic State String__jki_lib_state_machine.vi"("Period (ms)"=w32, "State"="Action: Periodic Work") -> ("State Out"=w34:string)  [unwired: 9 in]
              }
            }
            n10 = call <vilib>:"Add State(s) to Queue__jki_lib_state_machine.vi"("State(s) in Front (\"\")"=w27, "State(s) in (\"\")"=w31) -> ("States Out"=w30:string)  [unwired: 13 in]
          }
          event "Exit": Value Change {
            # "This ensures state is only output if \"OK\" is TRUE. It's not really needed here, since OK has a Latching mechanical action and will reset to FALSE after being read. This merely serves only as an example to show users how one can use Conditional State String."
            # "Exit Button Value Change (pressed) Event\n(this executes Macro: Exit to terminate the VI)"
            n11 = event-data() -> ()  [unwired: 1 in, 1 out]
            n12 = call <vilib>:"Conditional State String__jki_lib_state_machine.vi"("Do State(s)?"="Exit", "State"="UI: Status>>Exiting program\nMacro: Exit") -> ("State Out"=w35:string)  [unwired: 7 in]
            n13 = call <vilib>:"Add State(s) to Queue__jki_lib_state_machine.vi"("State(s) in Front (\"\")"=w35, "State(s) in (\"\")"=w41) -> ("States Out"=w40:string)  [unwired: 13 in]
          }
          event Panel Close? {
            # "Discard the event because we'll close the front panel ourselves in Macro: Exit"
            # "Close Panel button (pressed) Event\n(this executes Macro: Exit to terminate the VI)"
            n14 = event-data() -> ()  [unwired: 1 in, 1 out]
            n15 = event-data("Discard?"=TRUE) -> ()  [unwired: 1 in, 1 out]
            n16 = call <vilib>:"Add State(s) to Queue__jki_lib_state_machine.vi"("State(s) in Front (\"\")"="Macro: Exit", "State(s) in (\"\")"=w47) -> ("States Out"=w46:string)  [unwired: 13 in]
          }
          event "Connect Systems": Value Change {
            n17 = event-data() -> ()  [unwired: 1 in, 6 out]
            n18 = call <vilib>:"Add State(s) to Queue__jki_lib_state_machine.vi"("State(s) in Front (\"\")"="UI: Status>>Reinitializing connections\nMacro: Uninitialize\nMacro: Initialize Devices" ("State(s) in Front (\"\")"), "State(s) in (\"\")"=w50) -> ("States Out"=w51:string)  [unwired: 13 in]
          }
          event "Start Image Capture": Value Change {
            n19 = event-data() -> ()  [unwired: 1 in, 6 out]
            n20 = call <vilib>:"Add State(s) to Queue__jki_lib_state_machine.vi"("State(s) in Front (\"\")"="Cam: Calibration Pictures\nProcess: Start Image capture" ("State(s) in Front (\"\")"), "State(s) in (\"\")"=w55) -> ("States Out"=w56:string)  [unwired: 13 in]
          }
          event "Stop Image Capture": Value Change {
            n21 = event-data() -> ()  [unwired: 1 in, 6 out]
            n22 = call <vilib>:"Add State(s) to Queue__jki_lib_state_machine.vi"("State(s) in Front (\"\")"="Process: Auto Flush>>OFF\nProcess: Stop Image capture" ("State(s) in Front (\"\")"), "State(s) in (\"\")"=w61) -> ("States Out"=w62:string)  [unwired: 13 in]
          }
          event "Calibration Pictures": Value Change {
            n23 = event-data() -> ()  [unwired: 1 in, 6 out]
            n24 = call <vilib>:"Add State(s) to Queue__jki_lib_state_machine.vi"("State(s) in Front (\"\")"="Cam: Calibration Pictures" ("State(s) in Front (\"\")"), "State(s) in (\"\")"=w65) -> ("States Out"=w66:string)  [unwired: 13 in]
          }
          event "Reconnect Arduino Uno": Value Change {
            n25 = event-data() -> ()  [unwired: 1 in, 6 out]
            n26 = call <vilib>:"Add State(s) to Queue__jki_lib_state_machine.vi"("State(s) in Front (\"\")"="UI: Cursor Set>>Busy\nUno: Uninitialize\nUno: Initialize\nUI: Cursor Set>>Idle" ("State(s) in Front (\"\")"), "State(s) in (\"\")"=w71) -> ("States Out"=w70:string)  [unwired: 13 in]
          }
          event "Reconnect Pump": Value Change {
            n27 = event-data() -> ()  [unwired: 1 in, 6 out]
            n28 = call <vilib>:"Add State(s) to Queue__jki_lib_state_machine.vi"("State(s) in Front (\"\")"="UI: Cursor Set>>Busy\nPump: Empty\nPump: Uninitialize\nPump: Ask for size\nPump: Initialize\nUI: Cursor Set>>Idle" ("State(s) in Front (\"\")"), "State(s) in (\"\")"=w74) -> ("States Out"=w75:string)  [unwired: 13 in]
          }
          event "Reconnect Arduino mega": Value Change {
            n29 = event-data() -> ()  [unwired: 1 in, 6 out]
            n30 = call <vilib>:"Add State(s) to Queue__jki_lib_state_machine.vi"("State(s) in Front (\"\")"="UI: Cursor Set>>Busy\nMega: Uninitialize\nMega: Initialize\nUI: Cursor Set>>Idle" ("State(s) in Front (\"\")"), "State(s) in (\"\")"=w79) -> ("States Out"=w80:string)  [unwired: 13 in]
          }
          event "Reconnect Cams": Value Change {
            n31 = event-data() -> ()  [unwired: 1 in, 6 out]
            n32 = call <vilib>:"Add State(s) to Queue__jki_lib_state_machine.vi"("State(s) in Front (\"\")"="UI: Cursor Set>>Busy\nCam: Uninitialize\nCam: Initialize\nUI: Cursor Set>>Idle" ("State(s) in Front (\"\")"), "State(s) in (\"\")"=w85) -> ("States Out"=w84:string)  [unwired: 13 in]
          }
          event "Empty and Refill": Value Change {
            n33 = event-data() -> ()  [unwired: 1 in, 6 out]
            n34 = Unbundle By Name(w89) -> ("Arduino ISS.Phase3"=w88:bool)
            n35 = case shown="True" w88 {
              tunnel: ["UI: Cursor Set>>Busy\nMacro: Cycle valve\nPump: Response>>Status\nPump: Dispense\nUI: Cursor Set>>Idle" ("State(s) in Front (\"\")") "UI: Cursor Set>>Busy\nMega: Request status>>RFF\nMacro: Cycle valve\nPump: Response>>Status\nPump: Dispense\nUI: Cursor Set>>Idle" ("State(s) in Front (\"\")")] -> w90
              frame False {
              }
              frame True {
              }
            }
            n36 = call <vilib>:"Add State(s) to Queue__jki_lib_state_machine.vi"("State(s) in Front (\"\")"=w90, "State(s) in (\"\")"=w91) -> ("States Out"=w92:string)  [unwired: 13 in]
          }
          event "Close and Refill": Value Change {
            n37 = event-data() -> ()  [unwired: 1 in, 6 out]
            n38 = Unbundle By Name(w101) -> ("Kuvette Full"=w104:bool)
            n39 = Equal?(x=w104, y=TRUE) -> (x = y?=w102:bool)
            n40 = case shown="True" w102 {
              tunnel: w101 -> [w109 w113]
              tunnel: [w109 w112] -> w100
              tunnel: [FALSE w110] -> w99
              frame False {
              }
              frame True {
                n41 = Two Button Dialog(message="Is the Kuvett Empty?", 1:"NO!" ("F button name (\"Cancel\")"), 2:"Yes" ("T button name (\"OK\")")) -> (T button?=w111:bool)
                n42 = Not(x=w111) -> (.not. x?=w110:bool)
                n43 = Bundle By Name(cluster=w113, "Kuvette Full"=w110) -> (w112:T4)
              }
            }
            n44 = call-poly <vilib>:"Select State(s)__jki_lib_state_machine.vi"("State(s) if True (\"\")"="" ("State(s) if True (\"\")"), "Select"=w99, "State(s) if False (\"\")"="Uno: Valve Close\nPump: Response>>Status\nPump: Dispense" ("State(s) in Front (\"\")")) -> ("States Out"=w96:string)  [unwired: 12 in]
            n45 = call <vilib>:"Add State(s) to Queue__jki_lib_state_machine.vi"("State(s) in Front (\"\")"=w96, "State(s) in (\"\")"=w105) -> ("States Out"=w106:string)  [unwired: 13 in]
          }
          event "Open & Close": Value Change {
            n46 = event-data() -> ()  [unwired: 1 in, 6 out]
            n47 = Unbundle By Name(w118) -> ("Arduino ISS.Phase3"=w117:bool)
            n48 = case shown="False" w117 {
              tunnel: ["UI: Cursor Set>>Busy\nMacro: Cycle Valve\nUI: Cursor Set>>Idle" ("State(s) in Front (\"\")") "UI: Cursor Set>>Busy\nMega: Request status>>RFF\nMacro: Cycle Valve\nUI: Cursor Set>>Idle" ("State(s) in Front (\"\")")] -> w119
              frame False {
              }
              frame True {
              }
            }
            n49 = call <vilib>:"Add State(s) to Queue__jki_lib_state_machine.vi"("State(s) in Front (\"\")"=w119, "State(s) in (\"\")"=w121) -> ("States Out"=w122:string)  [unwired: 13 in]
          }
          event "Manual Open": Value Change {
            n50 = event-data() -> ()  [unwired: 1 in, 6 out]
            n51 = Unbundle By Name(w126) -> ("Arduino ISS.Phase3"=w125:bool)
            n52 = case shown="True" w125 {
              tunnel: ["Uno: Valve Open" ("State(s) in Front (\"\")") "Mega: Request status>>RFF\nUno: Valve Open" ("State(s) in Front (\"\")")] -> w127
              frame False {
              }
              frame True {
              }
            }
            n53 = call <vilib>:"Add State(s) to Queue__jki_lib_state_machine.vi"("State(s) in Front (\"\")"=w127, "State(s) in (\"\")"=w128) -> ("States Out"=w129:string)  [unwired: 13 in]
          }
          event "Manual Close": Value Change {
            n54 = event-data() -> ()  [unwired: 1 in, 6 out]
            n55 = call <vilib>:"Add State(s) to Queue__jki_lib_state_machine.vi"("State(s) in Front (\"\")"="Uno: Valve Close" ("State(s) in Front (\"\")"), "State(s) in (\"\")"=w134) -> ("States Out"=w135:string)  [unwired: 13 in]
          }
          event "Position": Value Change {
            n56 = event-data() -> ()  [unwired: 1 in, 6 out]
            n57 = Unbundle By Name(w142) -> ("Arduino SRS.Valve state"=w141:enum16{"Standby", "Close", "Open"})
            n58 = case shown="\"Standby\", Default" w141 {
              tunnel: ["Standby" ("string") "Close" ("string") "Open" ("string")] -> w139
              frame "Standby", Default {
              }
              frame "Close" {
              }
              frame "Open" {
              }
            }
            n59 = Concatenate Strings("Uno: Validate Valve Pos´>> " ("State(s) in Front (\"\")"), w139) -> (w138:string)
            n60 = call <vilib>:"Add State(s) to Queue__jki_lib_state_machine.vi"("State(s) in Front (\"\")"=w138, "State(s) in (\"\")"=w143) -> ("States Out"=w144:string)  [unwired: 13 in]
          }
          event "Pump Cycle": Value Change {
            n61 = event-data() -> ()  [unwired: 1 in, 6 out]
            n62 = Unbundle By Name(w154) -> ("Kuvette Full"=w157:bool)
            n63 = Equal?(x=w157, y=TRUE) -> (x = y?=w155:bool)
            n64 = case shown="False" w155 {
              tunnel: w154 -> [w162 w166]
              tunnel: [w162 w165] -> w153
              tunnel: [FALSE w163] -> w152
              frame False {
              }
              frame True {
                n65 = Two Button Dialog(message="Is the Kuvett Empty?", 1:"NO!" ("F button name (\"Cancel\")"), 2:"Yes" ("T button name (\"OK\")")) -> (T button?=w164:bool)
                n66 = Not(x=w164) -> (.not. x?=w163:bool)
                n67 = Bundle By Name(cluster=w166, "Kuvette Full"=w163) -> (w165:T4)
              }
            }
            n68 = call-poly <vilib>:"Select State(s)__jki_lib_state_machine.vi"("State(s) if True (\"\")"="" ("State(s) if True (\"\")"), "Select"=w152, "State(s) if False (\"\")"="UI: Status>>Pump cycle requested\nPump: Response>>Status\nPump: Dispense\nProcess: Delay>>2000\nPump: Response>>Status\nPump: Prime" ("State(s) in Front (\"\")")) -> ("States Out"=w151:string)  [unwired: 12 in]
            n69 = call <vilib>:"Add State(s) to Queue__jki_lib_state_machine.vi"("State(s) in Front (\"\")"=w151, "State(s) in (\"\")"=w158) -> ("States Out"=w159:string)  [unwired: 13 in]
          }
          event "Send CMD": Value Change {
            # "Manual Pump Command\nManually move the pump \nto the selected valve and plunger positions."
            n70 = event-data() -> ()  [unwired: 1 in, 6 out]
            n71 = Unbundle By Name(w178) -> ("Kuvette Full"=w181:bool, "Pump.Pump Size"=w175:enum16{"None", "Small", "Large"})
            n72 = Equal?(x=w181, y=TRUE) -> (x = y?=w179:bool)
            n73 = case shown="True" w179 {
              tunnel: w178 -> [w214 w218]
              tunnel: [w214 w217] -> w177
              tunnel: [FALSE w215] -> w171
              frame False {
              }
              frame True {
                n74 = Two Button Dialog(message="Is the Kuvett Empty?", 1:"NO!" ("F button name (\"Cancel\")"), 2:"Yes" ("T button name (\"OK\")")) -> (T button?=w216:bool)
                n75 = Not(x=w216) -> (.not. x?=w215:bool)
                n76 = Bundle By Name(cluster=w218, "Kuvette Full"=w215) -> (w217:T4)
              }
            }
            n77 = case shown="False" w171 {
              tunnel: w177 -> [w185 w212]
              tunnel: [w184 w212] -> w176
              tunnel: w175 -> [w183 _]
              tunnel: ["Pump: Response>>Status\nPump: Command" ("State(s) in Front (\"\")") "" ("State(s) in Front (\"\")")] -> w172
              frame False {
                n78 = To Long Integer(number="A") -> (32bit integer=w188:i32)
                n79 = case shown="\"Small\"" w183 {
                  tunnel: "I" -> [_ w197 w209]
                  tunnel: ["" w195 w210] -> w189
                  tunnel: w188 -> [_ w191 w200]
                  frame "None", Default {
                  }
                  frame "Large" {
                    n80 = Number To Decimal String(number=w191) -> (decimal integer string=w196:string)  [unwired: 1 in]
                    n81 = Number To Decimal String(number=w197) -> (decimal integer string=w194:string)  [unwired: 1 in]
                    n82 = Concatenate Strings("I" ("string"), w194, "A" ("string"), w196) -> (w195:string)
                  }
                  frame "Small" {
                    w201 = 1000 ("y")
                    n83 = Greater Or Equal?(x=w200, y=w201) -> (x >= y?=w202:bool)
                    n84 = Equal?(x=w209, y=1) -> (x = y?=w207:bool)
                    n85 = Select(t=w201, s=w202, f=w200) -> (s? t:f=w199:i32)
                    n86 = Select(t="I", s=w207, f="O") -> (s? t:f=w205:string)
                    n87 = Number To Decimal String(number=w199) -> (decimal integer string=w198:string)  [unwired: 1 in]
                    n88 = Concatenate Strings(w205, "A" ("string"), w198) -> (w210:string)
                  }
                }
                n89 = Bundle By Name(cluster=w185, "Pump.Command"=w189, "Pump.Flush Size"=w188) -> (w184:T4)
              }
              frame True {
              }
            }
            n90 = call <vilib>:"Add State(s) to Queue__jki_lib_state_machine.vi"("State(s) in Front (\"\")"=w172, "State(s) in (\"\")"=w173) -> ("States Out"=w174:string)  [unwired: 13 in]
          }
          event "Sample Name": Value Change {
            n91 = event-data() -> ()  [unwired: 1 in, 6 out]
            n92 = Bundle By Name(cluster=w224, "Main interface.Sample Name"="Sample Name") -> (w223:T4)
            n93 = call <vilib>:"Add State(s) to Queue__jki_lib_state_machine.vi"("State(s) in (\"\")"=w225) -> ("States Out"=w226:string)  [unwired: 14 in]
          }
          event "Operator": Value Change {
            n94 = event-data() -> ()  [unwired: 1 in, 6 out]
            n95 = Bundle By Name(cluster=w230, "Main interface.Operator"="Operator") -> (w229:T4)
            n96 = call <vilib>:"Add State(s) to Queue__jki_lib_state_machine.vi"("State(s) in (\"\")"=w231) -> ("States Out"=w232:string)  [unwired: 14 in]
          }
          event "Species Name": Value Change {
            n97 = event-data() -> ()  [unwired: 1 in, 6 out]
            n98 = Bundle By Name(cluster=w236, "Main interface.Species Name"="Species Name") -> (w235:T4)
            n99 = call <vilib>:"Add State(s) to Queue__jki_lib_state_machine.vi"("State(s) in (\"\")"=w237) -> ("States Out"=w238:string)  [unwired: 14 in]
          }
          event "Collection Date": Value Change {
            n100 = event-data() -> ()  [unwired: 1 in, 6 out]
            n101 = call "Timestamp_Converter.vi"("Date"="Collection Date") -> ("Date string"=w240:string)  [unwired: 7 in, 1 out]
            n102 = Bundle By Name(cluster=w242, "Extended setup.Collection date"=w240) -> (w241:T4)
            n103 = call <vilib>:"Add State(s) to Queue__jki_lib_state_machine.vi"("State(s) in (\"\")"=w243) -> ("States Out"=w244:string)  [unwired: 14 in]
          }
          event "Station": Value Change {
            n104 = event-data() -> ()  [unwired: 1 in, 6 out]
            n105 = Bundle By Name(cluster=w249, "Extended setup.Station"="Station") -> (w248:T4)
            n106 = call <vilib>:"Add State(s) to Queue__jki_lib_state_machine.vi"("State(s) in (\"\")"=w250) -> ("States Out"=w251:string)  [unwired: 14 in]
          }
          event "Location": Value Change {
            n107 = event-data() -> ()  [unwired: 1 in, 6 out]
            n108 = Bundle By Name(cluster=w255, "Extended setup.Location"="Location") -> (w254:T4)
            n109 = call <vilib>:"Add State(s) to Queue__jki_lib_state_machine.vi"("State(s) in (\"\")"=w256) -> ("States Out"=w257:string)  [unwired: 14 in]
          }
          event "Latitude": Value Change {
            n110 = event-data() -> ()  [unwired: 1 in, 6 out]
            n111 = Bundle By Name(cluster=w262, "Extended setup.Latitude"="Latitude") -> (w261:T4)
            n112 = call <vilib>:"Add State(s) to Queue__jki_lib_state_machine.vi"("State(s) in (\"\")"=w263) -> ("States Out"=w264:string)  [unwired: 14 in]
          }
          event "Longitude": Value Change {
            n113 = event-data() -> ()  [unwired: 1 in, 6 out]
            n114 = Bundle By Name(cluster=w267, "Extended setup.Longitude"="Longitude") -> (w266:T4)
            n115 = call <vilib>:"Add State(s) to Queue__jki_lib_state_machine.vi"("State(s) in (\"\")"=w268) -> ("States Out"=w269:string)  [unwired: 14 in]
          }
          event "Determiner": Value Change {
            n116 = event-data() -> ()  [unwired: 1 in, 6 out]
            n117 = Bundle By Name(cluster=w273, "Extended setup.Determiner"="Determiner") -> (w272:T4)
            n118 = call <vilib>:"Add State(s) to Queue__jki_lib_state_machine.vi"("State(s) in (\"\")"=w274) -> ("States Out"=w275:string)  [unwired: 14 in]
          }
          event "Sex": Value Change {
            n119 = event-data() -> ()  [unwired: 1 in, 6 out]
            n120 = Bundle By Name(cluster=w279, "Extended setup.Sex"="Sex") -> (w280:T4)
            n121 = call <vilib>:"Add State(s) to Queue__jki_lib_state_machine.vi"("State(s) in (\"\")"=w277) -> ("States Out"=w281:string)  [unwired: 14 in]
          }
          event "LegCamAtt": Value Change {
            n122 = event-data() -> ()  [unwired: 1 in, 6 out]
            n123 = Bundle By Name(cluster=w285, "Camera settings.Lens/camera settings.Legacy Cam Attributes"="LegCamAtt") -> (w284:T4)
            n124 = call <vilib>:"Add State(s) to Queue__jki_lib_state_machine.vi"("State(s) in (\"\")"=w286) -> ("States Out"=w287:string)  [unwired: 14 in]
          }
          event "Other notes": Value Change {
            n125 = event-data() -> ()  [unwired: 1 in, 6 out]
            n126 = Bundle By Name(cluster=w292, "Main interface.Other Notes"="Other notes") -> (w291:T4)
            n127 = call <vilib>:"Add State(s) to Queue__jki_lib_state_machine.vi"("State(s) in (\"\")"=w293) -> ("States Out"=w294:string)  [unwired: 14 in]
          }
          event "Aperture": Value Change {
            n128 = event-data() -> ()  [unwired: 1 in, 6 out]
            n129 = Bundle By Name(cluster=w298, "Camera settings.Lens/camera settings.Aperture"="Aperture") -> (w296:T4)
            n130 = call "Calibration_Update_2.0.vi"("Data"=w296) -> ("output cluster"=w295:T4)  [unwired: 2 in]
            n131 = call <vilib>:"Add State(s) to Queue__jki_lib_state_machine.vi"("State(s) in (\"\")"=w299) -> ("States Out"=w300:string)  [unwired: 14 in]
          }
          event "Exposure": Value Change {
            n132 = event-data() -> ()  [unwired: 1 in, 6 out]
            n133 = Unbundle By Name(w305) -> ("Camera settings.Lens/camera settings.Max Framerate"=w314:i32)
            n134 = case shown="\"Item 0\", Default" "Exposure" {
              tunnel: [1000.0 1500.0 2000.0 w319] -> w309
              frame "Item 0", Default {
              }
              frame "Item 1" {
              }
              frame "Item 2" {
              }
              frame "Item 3" {
                n135 = local read "Exposure Time"() -> (w319:dbl)
              }
            }
            n136 = Multiply(x=w309, y=10.0) -> (x*y=w312:dbl)
            n137 = Divide(x=1000000.0, y=w312) -> (x/y=w313:dbl)
            n138 = local write "Exposure Time"(w309) -> ()
            n139 = Max & Min(x=w313, y=w314) -> (min(x,y)=w304:dbl)  [unwired: 1 out]
            n140 = local write "Target framerate"(w304) -> ()
            n141 = Bundle By Name(cluster=w305, "Camera settings.Lens/camera settings.Exposure Time"=w309, "Camera settings.Lens/camera settings.Framerate"=w304) -> (w303:T4)
            n142 = call <vilib>:"Add State(s) to Queue__jki_lib_state_machine.vi"("State(s) in (\"\")"=w307) -> ("States Out"=w308:string)  [unwired: 14 in]
            n143 = call "Calibration_Update_2.0.vi"("Data"=w303) -> ("output cluster"=w302:T4)  [unwired: 2 in]
          }
          event "Exposure Time": Value Change {
            n144 = event-data() -> ()  [unwired: 1 in, 6 out]
            n145 = Unbundle By Name(w325) -> ("Camera settings.Lens/camera settings.Max Framerate"=w333:i32)
            n146 = Multiply(x="Exposure Time", y=10.0) -> (x*y=w330:dbl)
            n147 = Divide(x=1000000.0, y=w330) -> (x/y=w332:dbl)
            n148 = local write "Exposure"(enum32{"Item 0", "Item 1", "Item 2", "Item 3"}."Item 3" ("Exposure")) -> ()
            n149 = Max & Min(x=w332, y=w333) -> (min(x,y)=w321:dbl)  [unwired: 1 out]
            "Target framerate" <- w321
            n150 = Bundle By Name(cluster=w325, "Camera settings.Lens/camera settings.Exposure Time"="Exposure Time", "Camera settings.Lens/camera settings.Framerate"=w321) -> (w324:T4)
            n151 = call <vilib>:"Add State(s) to Queue__jki_lib_state_machine.vi"("State(s) in (\"\")"=w326) -> ("States Out"=w327:string)  [unwired: 14 in]
            n152 = call "Calibration_Update_2.0.vi"("Data"=w324) -> ("output cluster"=w323:T4)  [unwired: 2 in]
          }
          event "Img Proc Que Size": Value Change {
            n153 = event-data() -> ()  [unwired: 1 in, 6 out]
            n154 = property on="Process buffer" class="WFChart (strict)"("YScale.Maximum"="Img Proc Que Size") -> ()  [unwired: 2 in, 2 out]
            n155 = Bundle By Name(cluster=w336, "Ques.Image Process Queue Size"="Img Proc Que Size") -> (w335:T4)
            n156 = call <vilib>:"Add State(s) to Queue__jki_lib_state_machine.vi"("State(s) in (\"\")"=w337) -> ("States Out"=w338:string)  [unwired: 14 in]
          }
          event "Img Save Que Size": Value Change {
            n157 = event-data() -> ()  [unwired: 1 in, 6 out]
            n158 = property on="Save buffer" class="WFChart (strict)"("YScale.Maximum"="Img Save Que Size") -> ()  [unwired: 2 in, 2 out]
            n159 = Bundle By Name(cluster=w342, "Ques.Image Save Queue Size"="Img Save Que Size") -> (w341:T4)
            n160 = call <vilib>:"Add State(s) to Queue__jki_lib_state_machine.vi"("State(s) in (\"\")"=w343) -> ("States Out"=w344:string)  [unwired: 14 in]
          }
          event "Overload threshold": Value Change {
            n161 = event-data() -> ()  [unwired: 1 in, 6 out]
            n162 = Bundle By Name(cluster=w348, "Ques.Overload threshold"="Overload threshold") -> (w347:T4)
            n163 = call <vilib>:"Add State(s) to Queue__jki_lib_state_machine.vi"("State(s) in (\"\")"=w349) -> ("States Out"=w350:string)  [unwired: 14 in]
          }
          event "Max Framerate": Value Change {
            n164 = event-data() -> ()  [unwired: 1 in, 6 out]
            n165 = Unbundle By Name(w359) -> ("Camera settings.Lens/camera settings.Exposure Time"=w352:dbl)
            n166 = Multiply(x=w352, y=10.0) -> (x*y=w357:dbl)
            n167 = Divide(x=1000000.0, y=w357) -> (x/y=w358:dbl)
            n168 = Max & Min(x="Max Framerate", y=w358) -> (min(x,y)=w353:dbl)  [unwired: 1 out]
            n169 = Bundle By Name(cluster=w359, "Camera settings.Lens/camera settings.Max Framerate"="Max Framerate", "Camera settings.Lens/camera settings.Framerate"=w353) -> (w360:T4)
            n170 = local write "Target framerate"(w353) -> ()
            n171 = call <vilib>:"Add State(s) to Queue__jki_lib_state_machine.vi"("State(s) in (\"\")"=w361) -> ("States Out"=w362:string)  [unwired: 14 in]
          }
          event "New Sample timeout": Value Change {
            n172 = event-data() -> ()  [unwired: 1 in, 6 out]
            n173 = Bundle By Name(cluster=w366, "Camera settings.Detection settings.Timeout Sample"="New Sample timeout") -> (w365:T4)
            n174 = call <vilib>:"Add State(s) to Queue__jki_lib_state_machine.vi"("State(s) in (\"\")"=w367) -> ("States Out"=w368:string)  [unwired: 14 in]
          }
          event "Sample size threshold": Value Change {
            n175 = event-data() -> ()  [unwired: 1 in, 6 out]
            n176 = Bundle By Name(cluster=w372, "Camera settings.Detection settings.Sample size threshold"="Sample size threshold") -> (w371:T4)
            n177 = call <vilib>:"Add State(s) to Queue__jki_lib_state_machine.vi"("State(s) in (\"\")"=w373) -> ("States Out"=w374:string)  [unwired: 14 in]
          }
          event "DetectCrop": Value Change {
            n178 = event-data() -> ()  [unwired: 1 in, 6 out]
            n179 = Bundle By Name(cluster=w378, "Camera settings.Detection settings.Detection Region %"="DetectCrop") -> (w377:T4)
            n180 = call <vilib>:"Add State(s) to Queue__jki_lib_state_machine.vi"("State(s) in (\"\")"=w379) -> ("States Out"=w380:string)  [unwired: 14 in]
          }
          event "Change Crop": Value Change {
            n181 = event-data() -> ()  [unwired: 1 in, 6 out]
            n182 = call <vilib>:"Add State(s) to Queue__jki_lib_state_machine.vi"("State(s) in Front (\"\")"="Cam: Change Crop\nData: Save Settings" ("State(s) in Front (\"\")"), "State(s) in (\"\")"=w384) -> ("States Out"=w385:string)  [unwired: 13 in]
          }
          event "Overlay_Ring": Value Change {
            n183 = event-data() -> ()  [unwired: 1 in, 6 out]
            n184 = property on="Overlay_Ring" class="Ring (strict)"("Key Focus"=TRUE) -> ()  [unwired: 2 in, 2 out]
            n185 = call <vilib>:"Add State(s) to Queue__jki_lib_state_machine.vi"("State(s) in (\"\")"=w388) -> ("States Out"=w389:string)  [unwired: 14 in]
            "Overlay_tab" <- "Overlay_Ring"
          }
          event "Individual processed": Value Change {
            n186 = event-data() -> ()  [unwired: 1 in, 6 out]
            n187 = Unbundle By Name(w395) -> ("Auto Flush"=w394:bool)
            n188 = call-poly <vilib>:"Select State(s)__jki_lib_state_machine.vi"("State(s) if True (\"\")"="UI: Status>>Individual Processed\n\rMacro: Auto Flush" ("State(s) if True (\"\")"), "Select"=w394, "State(s) if False (\"\")"="UI: Status>>Individual Processed" ("State(s) if True (\"\")")) -> ("States Out"=w396:string)  [unwired: 12 in]
            n189 = call <vilib>:"Add State(s) to Queue__jki_lib_state_machine.vi"("State(s) in Front (\"\")"=w396, "State(s) in (\"\")"=w398) -> ("States Out"=w399:string)  [unwired: 13 in]
          }
          event "Get Status": Value Change {
            n190 = event-data() -> ()  [unwired: 1 in, 6 out]
            n191 = call <vilib>:"Add State(s) to Queue__jki_lib_state_machine.vi"("State(s) in Front (\"\")"="UI: Status>>Requesting F3 status\nMega: Request status" ("State(s) in Front (\"\")"), "State(s) in (\"\")"=w403) -> ("States Out"=w404:string)  [unwired: 13 in]
          }
          event "Get Barcode list": Value Change {
            n192 = event-data() -> ()  [unwired: 1 in, 6 out]
            n193 = call <vilib>:"Add State(s) to Queue__jki_lib_state_machine.vi"("State(s) in Front (\"\")"="Mega: Request Barcodes" ("State(s) in Front (\"\")"), "State(s) in (\"\")"=w408) -> ("States Out"=w409:string)  [unwired: 13 in]
          }
          event "Return Home": Value Change {
            n194 = event-data() -> ()  [unwired: 1 in, 6 out]
            n195 = call <vilib>:"Add State(s) to Queue__jki_lib_state_machine.vi"("State(s) in Front (\"\")"="Mega: Return Home" ("State(s) in Front (\"\")"), "State(s) in (\"\")"=w412) -> ("States Out"=w413:string)  [unwired: 13 in]
          }
          event "Send Barcode": Value Change {
            n196 = event-data() -> ()  [unwired: 1 in, 6 out]
            n197 = Number To Decimal String(number="Container nr.") -> (decimal integer string=w418:string)  [unwired: 1 in]
            n198 = Bundle By Name(cluster=w421, "Arduino ISS.Container nr."="Container nr.") -> (w420:T4)
            n199 = Concatenate Strings("Mega: Send Barcode>>" ("State(s) in Front (\"\")"), w418) -> (w417:string)
            n200 = call <vilib>:"Add State(s) to Queue__jki_lib_state_machine.vi"("State(s) in Front (\"\")"=w417, "State(s) in (\"\")"=w422) -> ("States Out"=w423:string)  [unwired: 13 in]
          }
          event "Rescan barcodes": Value Change {
            n201 = event-data() -> ()  [unwired: 1 in, 6 out]
            n202 = call <vilib>:"Add State(s) to Queue__jki_lib_state_machine.vi"("State(s) in Front (\"\")"="Mega: Scan Barcodes" ("State(s) in Front (\"\")"), "State(s) in (\"\")"=w426) -> ("States Out"=w427:string)  [unwired: 13 in]
          }
          event "Clear Error": Value Change {
            n203 = event-data() -> ()  [unwired: 1 in, 6 out]
            n204 = call <vilib>:"Add State(s) to Queue__jki_lib_state_machine.vi"("State(s) in Front (\"\")"="Mega: Clear error" ("State(s) in Front (\"\")"), "State(s) in (\"\")"=w431) -> ("States Out"=w432:string)  [unwired: 13 in]
          }
          event "Sorting sys.": Value Change {
            n205 = event-data() -> ()  [unwired: 1 in, 6 out]
            n206 = case shown="False" "Sorting sys." {
              frame False {
                n207 = property on="Initial size" class="DigNum (strict)"("DisabledEnum"=T7."Disabled and Grayed Out" ("Disabled")) -> ()  [unwired: 2 in, 2 out]
                n208 = property on="Size Interval" class="DigNum (strict)"("DisabledEnum"=T7."Disabled and Grayed Out" ("Disabled")) -> ()  [unwired: 2 in, 2 out]
                n209 = property on="Num. of containers" class="DigNum (strict)"("DisabledEnum"=T7."Disabled and Grayed Out" ("Disabled")) -> ()  [unwired: 2 in, 2 out]
              }
              frame True {
                n210 = property on="Initial size" class="DigNum (strict)"("DisabledEnum"=T7."Enabled" ("Disabled")) -> ()  [unwired: 2 in, 2 out]
                n211 = property on="Size Interval" class="DigNum (strict)"("DisabledEnum"=T7."Enabled" ("Disabled")) -> ()  [unwired: 2 in, 2 out]
                n212 = property on="Num. of containers" class="DigNum (strict)"("DisabledEnum"=T7."Enabled" ("Disabled")) -> ()  [unwired: 2 in, 2 out]
              }
            }
            n213 = Bundle By Name(cluster=w437, "Arduino ISS.Sorting sys."="Sorting sys.") -> (w436:T4)
            n214 = call <vilib>:"Add State(s) to Queue__jki_lib_state_machine.vi"("State(s) in (\"\")"=w438) -> ("States Out"=w439:string)  [unwired: 14 in]
          }
          event "Apply sorting val": Value Change {
            n215 = event-data() -> ()  [unwired: 1 in, 6 out]
            n216 = Bundle By Name(cluster=w450, "Arduino ISS.Initial size"="Initial size", "Arduino ISS.Size Interval"="Size Interval", "Arduino ISS.Mun. of containers"="Num. of containers") -> (w451:T4)
            n217 = call <vilib>:"Add State(s) to Queue__jki_lib_state_machine.vi"("State(s) in (\"\")"=w452) -> ("States Out"=w453:string)  [unwired: 14 in]
          }
          event "Save History": Value Change {
            n218 = event-data() -> ()  [unwired: 1 in, 6 out]
            n219 = call <vilib>:"Add State(s) to Queue__jki_lib_state_machine.vi"("State(s) in Front (\"\")"="UI: Status>>Saving history\nProcess: Save History" ("State(s) in Front (\"\")"), "State(s) in (\"\")"=w458) -> ("States Out"=w457:string)  [unwired: 13 in]
          }
        }
      }
      frame "---------- Core ----------" {
        # "Do not put any code in this frame.\n(it is a separator no-op)"
        n220 = call <vilib>:"Add State(s) to Queue__jki_lib_state_machine.vi"("State(s) in (\"\")"=w463) -> ("States Out"=w462:string)  [unwired: 14 in]
      }
      frame Default {
        w473 = 42 items=["No error", "Argument error", "Memory is full", "Out of zone", "End of file", "File already open", "Generic file I/O error", "File not found", "File permission error", "Disk is full", "Duplicate path", "Too many files open", "System feature not enabled", "Resource file not found", "Cannot add resource", "Resource not found", "Image not found", "Image memory error", "Pen does not exist", "Config type invalid", "Config token not found", "Config parse error", "Config memory error", "Bad external code format", "Bad external code offset", "External code not present", "Null window", "Destroy window error", "Null menu", "Print aborted", "Bad print record", "Print driver error", "Windows error during printing", "Memory error during printing", "Print dialog error", "Generic print error", "Invalid device refnum", "Device not found", "Device parameter error", "Device unit error", "Cannot open device", "Device call aborted", "Generic error", "Cancelled by user", "Object ID too low", "Object ID too high", "Object not in heap", "Unknown heap", "Unknown object (invalid DefProc)", "Unknown object (DefProc not in table)", "Message out of range", "Invalid (null) method", "Unknown message", "Manager call not supported", "Bad address", "Network operation in progress", "Network operation timed out", "Connection is busy", "Network attribute not supported", "Network error", "Address in use", "System out of memory", "Connection aborted", "Connection refused", "Not connected", "Already connected", "Connection closed", "Initialization error (interapplication manager)", "Bad occurrence", "Wait on unbound occurrence handler", "Occurrence queue overflow", "Datalog type conflict", "Unused", "Unrecognized type (interapplication manager)", "Memory corrupt", "Failed to make temporary DLL", "Old CIN version", "Drag socket not found", "Failed to load drop-object", "Failed to register OLE object", "Failed to release OLE object", "Format specifier type mismatch", "Unknown format specifier", "Too few format specifiers", "Too many format specifiers", "Scan failed", "Newer CIN version", "Error converting to variant", "Runtime menu error", "Password tampered", "Variant attribute not found", "Incompatible variant data type", "Event data is not available", "Event Store is not present", "Occurrence is not found", "Event Queue is not created", "Event info is not available", "Refnum passed is NULL", "Error retrieving Class GUID", "Error retrieving CoClass GUID", "Error retrieving TypeLib GUID.", "Bad built application magic bytes.", "Specific driver is different from the specific driver associated with the Logical Name.", "There is no session opened to the class driver.", "Max Error", "MAX - Error with config objects", "MAX - Error loading configuration", "MAX - Group not supported"]
        # "Current State"
        # "Do not delete, rename, or modify this frame.\n(this is used to capture unhandled states and typos)"
        # "Handle mistyped state name (developer tool)"
        n221 = Format Into String(format string="Software Exception: Unhandled State \"%s\"." ("message"), error in=w469, w464) -> (resulting string=w472:string, error out=w471:errorcluster)  [unwired: 1 in]
        n222 = call <vilib>:"Error Cluster From Error Code.vi"("show call chain? (False)"=TRUE, "error in (no error)"=w471, "error message (\"\")"=w472, "error code (0)"=w473) -> ("error out"=w470:errorcluster)  [unwired: 5 in]
        n223 = call <vilib>:"Add State(s) to Queue__jki_lib_state_machine.vi"("State(s) in (\"\")"=w468) -> ("States Out"=w467:string)  [unwired: 14 in]
      }
      frame "Initialize Core Data" {
        # "Do not delete, rename, or modify this frame.\n(this is used to determine panel behavior on exit)"
        # "originally closed?"
        # "exe?"
        # "If panel starts closed or is an EXE, then close it when we exit"
        n224 = property class="VI"() -> ("FP.State"=w477:T8)  [unwired: 2 in, 2 out]
        n225 = property class="App"() -> ("App.Kind"=w483:T9)  [unwired: 2 in, 2 out]
        n226 = control-ref of="Current VI Reference"() -> (w478:refnum<vi>)
        n227 = Equal?(x=w477, y=T8."Closed" ("Front Panel Window:State")) -> (x = y?=w475:bool)
        n228 = Equal?(x=w483, y=T9."Run Time System" ("Application:Kind")) -> (x = y?=w481:bool)
        n229 = Or(x=w475, y=w481) -> (x .or. y?=w479:bool)
        n230 = Bundle By Name(cluster=w480, "Core JKI.Current VI Reference"=w478, "Core JKI.Close Panel on Exit?"=w479) -> (w485:T4)
        n231 = call <vilib>:"Add State(s) to Queue__jki_lib_state_machine.vi"("State(s) in (\"\")"=w487) -> ("States Out"=w486:string)  [unwired: 14 in]
      }
      frame "Error Handler" {
        # "When running as sourcecode, this function will add previous state data to the error message to aid the developer in troubleshoot errors.\nIf run as an executable, no additional information is added to the error message."
        # "This state receives both Errors and Warnings which is how the Status of this wire can be FALSE"
        # "Unhandled Error -- Display it"
        # "Handle any errors or warnings here.\nYou can also output any states to clean-up after errors or warnings occur"
        # "Clear error or warning"
        n232 = disable-structure shown="Default" {
          disable-tunnel: w493 -> [w500 w501]
          disable-tunnel: w492 -> [w499 _]
          disable-tunnel: [w498 w501] -> w491
          frame condition #0 (active) {
            n233 = call <vilib>:"Append Error Details__jki_lib_state_machine.vi"("error in (no error)"=w500, "Previous State and Argument(s)"=w499) -> ("error out"=w498:errorcluster)  [unwired: 9 in]
          }
          frame condition #1 {
          }
        }
        n234 = call <vilib>:"General Error Handler.vi"("error in (no error)"=w491) -> ()  [unwired: 10 in, 5 out]
        n235 = call-poly <vilib>:"Select State(s)__jki_lib_state_machine.vi"("State(s) if True (\"\")"="/* Post Error States", "Select"=w491, "State(s) if False (\"\")"="/* Post Warning States") -> ("States Out"=w489:string)  [unwired: 12 in]
        n236 = call <vilib>:"Add State(s) to Queue__jki_lib_state_machine.vi"("State(s) in Front (\"\")"=w489, "State(s) in (\"\")"=w497) -> ("States Out"=w496:string)  [unwired: 13 in]
      }
      frame "Exit" {
        # "Do not put any code in this frame.\n(No errors that occur here will be handled.)"
        n237 = Bundle By Name(cluster=w503, "Exit"=TRUE) -> (w502:T4)
        n238 = call <vilib>:"Add State(s) to Queue__jki_lib_state_machine.vi"("State(s) in (\"\")"=w508) -> ("States Out"=w507:string)  [unwired: 14 in]
      }
      frame "---------- Data ----------" {
        # "Do not put any code in this frame.\n(It is a separator no-op. You can make a copy of this frame to create a new Data frame)"
        n239 = call <vilib>:"Add State(s) to Queue__jki_lib_state_machine.vi"("State(s) in (\"\")"=w512) -> ("States Out"=w511:string)  [unwired: 14 in]
      }
      frame "Data: Initialize" {
        w514 = T12 {"Current VI Reference"=refnum, "Close Panel on Exit?"=FALSE}  # Core
        # "Initialize the shift-register data, here.\n(data names are defined by what you wire into the bundle function)"
        n240 = Bundle By Name(cluster=w515, "Core JKI"=w514) -> (w513:T4)
        n241 = call <vilib>:"Add State(s) to Queue__jki_lib_state_machine.vi"("State(s) in (\"\")"=w518) -> ("States Out"=w517:string)  [unwired: 14 in]
      }
      frame "Data: Camera ID from file" {
        # "Do not put any code in this frame.\n(It is a separator no-op. You can make a copy of this frame to create a new Data frame)"
        n242 = call <vilib>:"Application Directory.vi"() -> ("Application Directory"=w534:path)
        n243 = Path To String(path=w534) -> (string=w535:string)
        n244 = Concatenate Strings(w535, "\\CameraID.ini" ("string")) -> (w532:string)
        n245 = String To Path(string=w532) -> (path=w531:path)
        n246 = call-poly <vilib>:"Read From XML File.vi"("error in (no error)"=w523, "XML File Path"=w531) -> ("error out"=w529:errorcluster, "XML Elements"=w530:string)  [unwired: 7 in, 1 out]
        n247 = Unflatten From XML(xml string=w530, type=T10 {"CAM_ID1"=0, "CAM_ID2"=0} ("CAM_ID"), error in (no error)=w529) -> (value=w527:T10, error out=w525:errorcluster)
        n248 = Unbundle By Name(w527) -> ("CAM_ID1"=w528:i32)
        n249 = Equal To 0?(x=w528) -> (x = 0?=w522:bool)
        n250 = case shown="False" w522 {
          tunnel: w527 -> [w542 _]
          tunnel: [w544 errorcluster {"status"=FALSE, "code"=0, "source"=""} ("error out")] -> w524
          tunnel: w525 -> [w544 _]
          tunnel: w521 -> [w543 w547]
          tunnel: [w539 w547] -> w520
          tunnel: ["" "Uno: Cam Id request"] -> w519
          frame False {
            n251 = Unbundle By Name(w542) -> ("CAM_ID1"=w541:i32, "CAM_ID2"=w540:i32)
            n252 = Bundle By Name(cluster=w543, "Camera 1.Cam1 ID"=w541, "Camera 2.Cam2 ID"=w540) -> (w539:T4)
          }
          frame True {
            n253 = One Button Dialog(message="Camera ID's not found on file") -> ()  [unwired: 1 in, 1 out]
          }
        }
        n254 = call <vilib>:"Add State(s) to Queue__jki_lib_state_machine.vi"("State(s) in Front (\"\")"=w519, "State(s) in (\"\")"=w537) -> ("States Out"=w536:string)  [unwired: 13 in]
      }
      frame "Data: Save Cam Id" {
        # "Do not put any code in this frame.\n(It is a separator no-op. You can make a copy of this frame to create a new Data frame)"
        n255 = Unbundle By Name(w553) -> ("Camera 1.Cam1 ID"=w552:i32, "Camera 2.Cam2 ID"=w551:i32)
        n256 = call <vilib>:"Application Directory.vi"() -> ("Application Directory"=w559:path)
        n257 = Bundle By Name(cluster=T10 {"CAM_ID1"=0, "CAM_ID2"=0} ("CAM_ID"), "CAM_ID1"=w552, "CAM_ID2"=w551) -> (w554:T10)
        n258 = Path To String(path=w559) -> (string=w560:string)
        n259 = Concatenate Strings(w560, "\\CameraID.ini" ("string")) -> (w557:string)
        n260 = String To Path(string=w557) -> (path=w556:path)
        n261 = Flatten To XML(6:w554) -> (2:w561:string)
        n262 = call-poly <vilib>:"Write to XML File.vi"("error in (no error)"=w550, "XML Input"=w561, "XML File Path"=w556) -> ("error out"=w549:errorcluster)  [unwired: 6 in, 2 out]
        n263 = case shown="No Error" w549 {
          frame No Error {
          }
          frame Error {
            n264 = One Button Dialog(message="Camera ID Save Error!\nError while saving camera IDs") -> ()  [unwired: 1 in, 1 out]
          }
        }
        n265 = call <vilib>:"Add State(s) to Queue__jki_lib_state_machine.vi"("State(s) in (\"\")"=w563) -> ("States Out"=w562:string)  [unwired: 14 in]
      }
      frame "Data: Save Settings" {
        # "Do not put any code in this frame.\n(It is a separator no-op. You can make a copy of this frame to create a new Data frame)"
        n266 = call <vilib>:"Application Directory.vi"() -> ("Application Directory"=w571:path)
        n267 = Path To String(path=w571) -> (string=w572:string)
        n268 = Concatenate Strings(w572, "\\settings.ini" ("string")) -> (w569:string)
        n269 = String To Path(string=w569) -> (path=w568:path)
        n270 = Flatten To XML(6:w565) -> (2:w573:string)
        n271 = call-poly <vilib>:"Write to XML File.vi"("error in (no error)"=w566, "XML Input"=w573, "XML File Path"=w568) -> ("error out"=w567:errorcluster)  [unwired: 6 in, 2 out]
        n272 = call <vilib>:"Add State(s) to Queue__jki_lib_state_machine.vi"("State(s) in (\"\")"=w575) -> ("States Out"=w574:string)  [unwired: 14 in]
      }
      frame "Data: Cleanup" {
        # "Cleanup any data and references, here.\n(this is called automatically, by the Macro: Exit)"
        n273 = Unbundle By Name(w577) -> ("Core JKI.Current VI Reference"=w576:refnum<vi>)
        n274 = Close Reference(reference=w576, error in (no error)=w579) -> (error out=w578:errorcluster)
        n275 = call <vilib>:"Add State(s) to Queue__jki_lib_state_machine.vi"("State(s) in (\"\")"=w581) -> ("States Out"=w580:string)  [unwired: 14 in]
      }
      frame "---------- UI ----------" {
        # "Do not put any code in this frame.\n(It is a separator no-op. You can make a copy of this frame to create a new UI frame)"
        n276 = call <vilib>:"Add State(s) to Queue__jki_lib_state_machine.vi"("State(s) in (\"\")"=w585) -> ("States Out"=w584:string)  [unwired: 14 in]
      }
      frame "UI: Initialize" {
        w586 = u16 7 items=["System", "Session Data", "Extended Setup", "Camera", "Dispenser", "Phase3", "Stats", "History"] ("Overlay_Ring")
        w590 = FALSE ("Pump")
        w595 = T13 [] ("History Data")
        # "BETA"
        # "Initialize the User Interface, here.\n(this is called automatically, by the Macro: Initialize)"
        n277 = property on="Overlay_tab" class="TabCtl (strict)"("Page Labels Display Visible?"=FALSE) -> ()  [unwired: 2 in, 2 out]
        n278 = property on="Process buffer" class="WFChart (strict)"("History Data"=w595) -> ()  [unwired: 2 in, 2 out]
        n279 = property on="Save buffer" class="WFChart (strict)"("History Data"=w595) -> ()  [unwired: 2 in, 2 out]
        n280 = local write "Exposure"(enum32{"Item 0", "Item 1", "Item 2", "Item 3"}."Item 3" ("Exposure")) -> ()
        n281 = call "Read Exe Version.vi"("beta?"=TRUE, "Application name"=path "SRS.exe") -> ("Title String"=→"System Version":string)  [unwired: 6 in, 3 out]
        n282 = Format Date/Time String(time format string (%c)="%y%m%d-%H;%M;%S") -> (date/time string=w588:string)  [unwired: 2 in]
        n283 = local write "Overlay_tab"(T1."History" ("Overlay_tab")) -> ()
        n284 = local write "Active"(w590) -> ()
        n285 = local write "Pump"(w590) -> ()
        n286 = local write "Valve"(w590) -> ()
        n287 = local write "Phase 3"(w590) -> ()
        n288 = local write "Ready"(w590) -> ()
        n289 = local write "Cam 1"(w590) -> ()
        n290 = local write "Cam 2"(w590) -> ()
        n291 = property on="Overlay_Ring" class="Ring (strict)"("Value"=w586) -> ()  [unwired: 2 in, 2 out]
        n292 = Bundle By Name(cluster=w593, "Timestamp Start"=w588, "Img_Capt"=w590, "Auto Flush"=w590) -> (w592:T4)
        n293 = property on="Auto Flush" class="Bool (strict)"("Value"=w590) -> ()  [unwired: 2 in, 2 out]
        n294 = property on="Auto Flush" class="Bool (strict)"("DisabledEnum"=T7."Disabled and Grayed Out" ("Disabled")) -> ()  [unwired: 2 in, 2 out]
        n295 = call <vilib>:"Add State(s) to Queue__jki_lib_state_machine.vi"("State(s) in (\"\")"=w602) -> ("States Out"=w601:string)  [unwired: 14 in]
      }
      frame "UI: Display Cluster Data" {
        # "Do not put any code in this frame.\n(It is a separator no-op. You can make a copy of this frame to create a new UI frame)"
        n296 = Unbundle By Name(w625) -> ("Main interface.Operator"=w623:string, "Main interface.Sample Name"=w622:string, "Main interface.Species Name"=w621:string, "Main interface.Other Notes"=w620:string, "Extended setup.Location"=w619:string, "Extended setup.Latitude"=w618:string, "Extended setup.Longitude"=w617:string, "Extended setup.Determiner"=w616:string, "Extended setup.Sex"=w615:string, "Extended setup.Station"=w614:string, "Extended setup.Collection date"=w624:string, "Ques.Image Process Queue Size"=w609:i32, "Ques.Image Save Queue Size"=w608:i32, "Ques.Overload threshold"=w613:i32, "Camera settings.Detection settings.Sample size threshold"=w612:i32, "Camera settings.Detection settings.Timeout Sample"=w604:i32, "Camera settings.Detection settings.Detection Region %"=w605:dbl, "Camera settings.Lens/camera settings.Aperture"=w606:enum32{"Item 0", "Item 1", "Item 2", "Item 3"}, "Camera settings.Lens/camera settings.Max Framerate"=w611:i32, "Camera settings.Lens/camera settings.Framerate"=w610:i32, "Camera settings.Lens/camera settings.Legacy Cam Attributes"=w603:bool, "Camera settings.Lens/camera settings.Exposure Time"=w607:dbl)
        n297 = call "Timestamp_Converter.vi"("Date String"=w624) -> ("Date"=w626:timestamp)  [unwired: 7 in, 1 out]
        n298 = local write "Operator"(w623) -> ()
        n299 = local write "Sample Name"(w622) -> ()
        n300 = local write "Species Name"(w621) -> ()
        n301 = local write "Other notes"(w620) -> ()
        n302 = local write "Location"(w619) -> ()
        n303 = local write "Latitude"(w618) -> ()
        n304 = local write "Longitude"(w617) -> ()
        n305 = local write "Determiner"(w616) -> ()
        n306 = local write "Sex"(w615) -> ()
        n307 = local write "Station"(w614) -> ()
        n308 = local write "Collection Date"(w626) -> ()
        n309 = local write "Img Proc Que Size"(w609) -> ()
        n310 = local write "Img Save Que Size"(w608) -> ()
        n311 = local write "Overload threshold"(w613) -> ()
        n312 = local write "Sample size threshold"(w612) -> ()
        n313 = local write "New Sample timeout"(w604) -> ()
        n314 = local write "DetectCrop"(w605) -> ()
        n315 = local write "Aperture"(w606) -> ()
        n316 = local write "Max Framerate"(w611) -> ()
        n317 = local write "Target framerate"(w610) -> ()
        n318 = local write "LegCamAtt"(w603) -> ()
        n319 = local write "Exposure Time"(w607) -> ()
        n320 = property on="Process buffer" class="WFChart (strict)"("YScale.Maximum"=w609) -> ()  [unwired: 2 in, 2 out]
        n321 = property on="Save buffer" class="WFChart (strict)"("YScale.Maximum"=w608) -> ()  [unwired: 2 in, 2 out]
        n322 = call <vilib>:"Add State(s) to Queue__jki_lib_state_machine.vi"("State(s) in (\"\")"=w629) -> ("States Out"=w628:string)  [unwired: 14 in]
      }
      frame "UI: Disabled and Grayed Out" {
        w630 = T7."Disabled and Grayed Out" ("Disabled")
        # "Do not put any code in this frame.\n(It is a separator no-op. You can make a copy of this frame to create a new UI frame)"
        n323 = property on="Start Image Capture" class="Bool"("DisabledEnum"=w630) -> ()  [unwired: 2 in, 2 out]
        n324 = property on="Calibration Pictures" class="Bool"("DisabledEnum"=w630) -> ()  [unwired: 2 in, 2 out]
        n325 = property on="Connect Systems" class="Bool"("DisabledEnum"=w630) -> ()  [unwired: 2 in, 2 out]
        n326 = property on="Close and Refill" class="Bool"("DisabledEnum"=w630) -> ()  [unwired: 2 in, 2 out]
        n327 = property on="Empty and Refill" class="Bool"("DisabledEnum"=w630) -> ()  [unwired: 2 in, 2 out]
        n328 = property on="Pump Cycle" class="Bool"("DisabledEnum"=w630) -> ()  [unwired: 2 in, 2 out]
        n329 = property on="Send CMD" class="Bool"("DisabledEnum"=w630) -> ()  [unwired: 2 in, 2 out]
        n330 = property on="Open & Close" class="Bool"("DisabledEnum"=w630) -> ()  [unwired: 2 in, 2 out]
        n331 = property on="Manual Close" class="Bool"("DisabledEnum"=w630) -> ()  [unwired: 2 in, 2 out]
        n332 = property on="Manual Open" class="Bool"("DisabledEnum"=w630) -> ()  [unwired: 2 in, 2 out]
        n333 = property on="Position" class="Bool"("DisabledEnum"=w630) -> ()  [unwired: 2 in, 2 out]
        n334 = property on="Get Status" class="Bool"("DisabledEnum"=w630) -> ()  [unwired: 2 in, 2 out]
        n335 = property on="Get Barcode list" class="Bool"("DisabledEnum"=w630) -> ()  [unwired: 2 in, 2 out]
        n336 = property on="Return Home" class="Bool"("DisabledEnum"=w630) -> ()  [unwired: 2 in, 2 out]
        n337 = property on="Send Barcode" class="Bool"("DisabledEnum"=w630) -> ()  [unwired: 2 in, 2 out]
        n338 = property on="Rescan barcodes" class="Bool"("DisabledEnum"=w630) -> ()  [unwired: 2 in, 2 out]
        n339 = property on="Clear Error" class="Bool"("DisabledEnum"=w630) -> ()  [unwired: 2 in, 2 out]
        n340 = call <vilib>:"Add State(s) to Queue__jki_lib_state_machine.vi"("State(s) in (\"\")"=w634) -> ("States Out"=w633:string)  [unwired: 14 in]
      }
      frame "UI: Enabled" {
        w635 = T7."Enabled" ("Disabled")
        # "Do not put any code in this frame.\n(It is a separator no-op. You can make a copy of this frame to create a new UI frame)"
        n341 = property on="Start Image Capture" class="Bool"("DisabledEnum"=w635) -> ()  [unwired: 2 in, 2 out]
        n342 = property on="Calibration Pictures" class="Bool"("DisabledEnum"=w635) -> ()  [unwired: 2 in, 2 out]
        n343 = property on="Connect Systems" class="Bool"("DisabledEnum"=w635) -> ()  [unwired: 2 in, 2 out]
        n344 = property on="Close and Refill" class="Bool"("DisabledEnum"=w635) -> ()  [unwired: 2 in, 2 out]
        n345 = property on="Empty and Refill" class="Bool"("DisabledEnum"=w635) -> ()  [unwired: 2 in, 2 out]
        n346 = property on="Pump Cycle" class="Bool"("DisabledEnum"=w635) -> ()  [unwired: 2 in, 2 out]
        n347 = property on="Send CMD" class="Bool"("DisabledEnum"=w635) -> ()  [unwired: 2 in, 2 out]
        n348 = property on="Open & Close" class="Bool"("DisabledEnum"=w635) -> ()  [unwired: 2 in, 2 out]
        n349 = property on="Manual Close" class="Bool"("DisabledEnum"=w635) -> ()  [unwired: 2 in, 2 out]
        n350 = property on="Manual Open" class="Bool"("DisabledEnum"=w635) -> ()  [unwired: 2 in, 2 out]
        n351 = property on="Position" class="Bool"("DisabledEnum"=w635) -> ()  [unwired: 2 in, 2 out]
        n352 = property on="Get Status" class="Bool"("DisabledEnum"=w635) -> ()  [unwired: 2 in, 2 out]
        n353 = property on="Get Barcode list" class="Bool"("DisabledEnum"=w635) -> ()  [unwired: 2 in, 2 out]
        n354 = property on="Return Home" class="Bool"("DisabledEnum"=w635) -> ()  [unwired: 2 in, 2 out]
        n355 = property on="Send Barcode" class="Bool"("DisabledEnum"=w635) -> ()  [unwired: 2 in, 2 out]
        n356 = property on="Rescan barcodes" class="Bool"("DisabledEnum"=w635) -> ()  [unwired: 2 in, 2 out]
        n357 = property on="Clear Error" class="Bool"("DisabledEnum"=w635) -> ()  [unwired: 2 in, 2 out]
        n358 = call <vilib>:"Add State(s) to Queue__jki_lib_state_machine.vi"("State(s) in (\"\")"=w639) -> ("States Out"=w638:string)  [unwired: 14 in]
      }
      frame "UI: Status" {
        # "Do not put any code in this frame.\n(It is a separator no-op. You can make a copy of this frame to create a new UI frame)"
        n359 = Unbundle By Name(w641) -> ("Timestamp Start"=w640:string)
        n360 = Concatenate Strings("Starting system", w640) -> (w646:string)
        n361 = Format Date/Time String(time format string (%c)="%H;%M;%S") -> (date/time string=w642:string)  [unwired: 2 in]
        n362 = call <vilib>:"Space Constant.vi"() -> ("String"=w643:string)
        n363 = feedback #1(w646) -> (w650:string)
        n364 = Concatenate Strings(w650, "\r\n", w642, w643, w644) -> (w648:string)
        "Status History" <- w648
        n365 = feedback-in #1(w648) -> ()
        n366 = Bundle By Name(cluster=w641, "Status History"=w648) -> (w649:T4)
        n367 = call <vilib>:"Add State(s) to Queue__jki_lib_state_machine.vi"("State(s) in (\"\")"=w654) -> ("States Out"=w653:string)  [unwired: 14 in]
        "Status" <- w644
      }
      frame "UI: Popup" {
        # "Do not put any code in this frame.\n(It is a separator no-op. You can make a copy of this frame to create a new UI frame)"
        n368 = Concatenate Strings("The system has experienced an\nerror:  " ("string"), w657, ". \nSystem is stopped and user interaction is needed." ("string")) -> (w655:string)
        n369 = One Button Dialog(message=w655) -> ()  [unwired: 1 in, 1 out]
        n370 = call <vilib>:"Add State(s) to Queue__jki_lib_state_machine.vi"("State(s) in (\"\")"=w662) -> ("States Out"=w661:string)  [unwired: 14 in]
      }
      frame "UI: Uninitialize" {
        # "Cleanup the User Interface, here.\n(this is called automatically, by the Macro: Exit)"
        n371 = property on="Overlay_tab" class="TabCtl (strict)"("Page Labels Display Visible?"=TRUE) -> ()  [unwired: 2 in, 2 out]
        n372 = call <vilib>:"Add State(s) to Queue__jki_lib_state_machine.vi"("State(s) in (\"\")"=w667) -> ("States Out"=w666:string)  [unwired: 14 in]
      }
      frame "UI: Cursor Set" {
        # "Argument"
        # "Set and Unset Cursor Busy.\n(Usage: \"UI: Cursor Set >> Busy|Idle\")"
        n373 = case shown="\"Idle\", Default" w668 {
          tunnel: w670 -> [w675 w677]
          tunnel: [w674 w676] -> w669
          frame "Idle", Default {
            n374 = call <vilib>:"Unset Busy.vi"("error in (no error)"=w675) -> ("error out"=w674:errorcluster)  [unwired: 10 in]
          }
          frame "Busy" {
            n375 = call <vilib>:"Set Busy.vi"("error in (no error)"=w677) -> ("error out"=w676:errorcluster)  [unwired: 9 in, 1 out]
          }
        }
        n376 = call <vilib>:"Add State(s) to Queue__jki_lib_state_machine.vi"("State(s) in (\"\")"=w673) -> ("States Out"=w672:string)  [unwired: 14 in]
      }
      frame "UI: Front Panel State" {
        # "Argument"
        # "Set Front Panel Open or Closed\n(Usage: \"UI: Front Panel State >> Open|Close\")"
        n377 = Unbundle By Name(w680) -> ("Core JKI.Current VI Reference"=w679:refnum<vi>)
        n378 = case shown="\"Close\", \"Closed\"" w678 {
          tunnel: w682 -> [w690 w705 w716 w729 w742]
          tunnel: [w692 w706 w718 w731 w744] -> w681
          tunnel: w679 -> [w691 w703 w717 w730 w743]
          frame "Open", "Standard", Default {
            w685 = T8."Standard" ("State")
            n379 = property class="VI"(reference=w691, error in=w690) -> (reference out=w688:refnum<vi>, error out=w689:errorcluster, "FP.State"=w687:T8)
            n380 = Not Equal?(x=w687, y=w685) -> (x != y?=w686:bool)
            n381 = case shown="True" w686 {
              tunnel: [w696 w698] -> w692
              tunnel: w689 -> [w695 w698]
              tunnel: w688 -> [w694 _]
              tunnel: w685 -> [w693 _]
              frame True {
                n382 = invoke class="VI" method="FP.Open"(reference=w694, error in=w695, "Activate"=TRUE, "State"=w693) -> (error out=w696:errorcluster)  [unwired: 1 in, 4 out]
              }
              frame False {
              }
            }
          }
          frame "Close", "Closed" {
            n383 = property class="VI"(reference=w703, error in=w705) -> (reference out=w702:refnum<vi>, error out=w704:errorcluster, "FP.State"=w700:T8)
            n384 = Not Equal?(x=w700, y=T8."Closed" ("Front Panel Window:State")) -> (x != y?=w699:bool)
            n385 = case shown="True" w699 {
              tunnel: [w707 w710] -> w706
              tunnel: w704 -> [w707 w709]
              tunnel: w702 -> [_ w708]
              frame False {
              }
              frame True {
                n386 = invoke class="VI" method="FP.Close"(reference=w708, error in=w709) -> (error out=w710:errorcluster)  [unwired: 1 in, 2 out]
              }
            }
          }
          frame "Hidden", "Hide" {
            w711 = T8."Hidden" ("State")
            n387 = property class="VI"(reference=w717, error in=w716) -> (reference out=w714:refnum<vi>, error out=w715:errorcluster, "FP.State"=w713:T8)
            n388 = Not Equal?(x=w713, y=w711) -> (x != y?=w712:bool)
            n389 = case shown="True" w712 {
              tunnel: [w722 w723] -> w718
              tunnel: w715 -> [w721 w723]
              tunnel: w714 -> [w720 _]
              tunnel: w711 -> [w719 _]
              frame True {
                n390 = invoke class="VI" method="FP.Open"(reference=w720, error in=w721, "State"=w719) -> (error out=w722:errorcluster)  [unwired: 2 in, 4 out]
              }
              frame False {
              }
            }
          }
          frame "Minimize", "Minimized" {
            w724 = T8."Minimized" ("State")
            n391 = property class="VI"(reference=w730, error in=w729) -> (reference out=w727:refnum<vi>, error out=w728:errorcluster, "FP.State"=w726:T8)
            n392 = Not Equal?(x=w726, y=w724) -> (x != y?=w725:bool)
            n393 = case shown="True" w725 {
              tunnel: [w735 w736] -> w731
              tunnel: w728 -> [w734 w736]
              tunnel: w727 -> [w733 _]
              tunnel: w724 -> [w732 _]
              frame True {
                n394 = invoke class="VI" method="FP.Open"(reference=w733, error in=w734, "State"=w732) -> (error out=w735:errorcluster)  [unwired: 2 in, 4 out]
              }
              frame False {
              }
            }
          }
          frame "Maximize", "Maximized" {
            w737 = T8."Maximized" ("State")
            n395 = property class="VI"(reference=w743, error in=w742) -> (reference out=w740:refnum<vi>, error out=w741:errorcluster, "FP.State"=w739:T8)
            n396 = Not Equal?(x=w739, y=w737) -> (x != y?=w738:bool)
            n397 = case shown="True" w738 {
              tunnel: [w748 w749] -> w744
              tunnel: w741 -> [w747 w749]
              tunnel: w740 -> [w746 _]
              tunnel: w737 -> [w745 _]
              frame True {
                n398 = invoke class="VI" method="FP.Open"(reference=w746, error in=w747, "State"=w745) -> (error out=w748:errorcluster)  [unwired: 2 in, 4 out]
              }
              frame False {
              }
            }
          }
        }
        n399 = call <vilib>:"Add State(s) to Queue__jki_lib_state_machine.vi"("State(s) in (\"\")"=w684) -> ("States Out"=w683:string)  [unwired: 14 in]
      }
      frame "---------- Macro ----------" {
        # "Do not put any code in this frame.\n(It is a separator no-op. You can make a copy of this frame to create a new Macro frame)"
        n400 = call <vilib>:"Add State(s) to Queue__jki_lib_state_machine.vi"("State(s) in (\"\")"=w753) -> ("States Out"=w752:string)  [unwired: 14 in]
      }
      frame "Macro: Initialize" {
        # "Initialization Macro\n(This is called once, when the VI starts)"
        n401 = call <vilib>:"Add State(s) to Queue__jki_lib_state_machine.vi"("State(s) in Front (\"\")"="UI: Cursor Set>>Busy\nUI: Initialize\nUI: Status>>Initialize data\nData: Initialize\nInitialize Core Data\nUI: Status>>Initialize UI\nUI: Display Cluster Data\nUI: Front Panel State >> Maximize\nUI: Disabled and Grayed Out\nUI: Status>>Initializing Serial Com.\nProcess: Identify Serial Communication\nUno: System Serial and Version\nUI: Status>>Serial connections initiated\nUI: Status>>Initializing Cams\nData: Camera ID from file\nCam: Initialize\nPump: Response>>Status\nPump: Prime\nUI: Enabled\nUI: Cursor Set>>Idle\nUI: Status>>Welcome ", "State(s) in (\"\")"=w758) -> ("States Out"=w757:string)  [unwired: 13 in]
      }
      frame "Macro: Initialize Devices" {
        # "Do not put any code in this frame.\n(It is a separator no-op. You can make a copy of this frame to create a new Macro frame)"
        n402 = call <vilib>:"Add State(s) to Queue__jki_lib_state_machine.vi"("State(s) in Front (\"\")"="UI: Cursor Set>>Busy\nUI: Status>>Initialize Arduino Uno\nUno: Initialize\nUI: Status>>Initialize Pump\nPump: Initialize\nUI: Status>>Initialize Arduino Mega\nMega: Initialize\nUI: Status>>Initialize Cams\nCam: Initialize\nUI: Cursor Set>>Idle" ("State(s) in Front (\"\")"), "State(s) in (\"\")"=w763) -> ("States Out"=w762:string)  [unwired: 13 in]
      }
      frame "Macro: Uninitialize" {
        # "Do not put any code in this frame.\n(It is a separator no-op. You can make a copy of this frame to create a new Macro frame)"
        n403 = call <vilib>:"Add State(s) to Queue__jki_lib_state_machine.vi"("State(s) in Front (\"\")"="UI: Cursor Set>>Busy\nUI: Status>>Uninitialize Arduino Uno\nUno: Uninitialize\nUI: Status>>Empty Pump\nPump: Response>>Status\nPump: Empty\nUI: Status>>Uninitialize Pump\nPump: Uninitialize\nUI: Status>>Uninitialize Arduino Mega\nMega: Uninitialize\nUI: Status>>Uninitialize Cams\nCam: Uninitialize\nUI: Cursor Set>>Idle" ("State(s) in Front (\"\")"), "State(s) in (\"\")"=w768) -> ("States Out"=w767:string)  [unwired: 13 in]
      }
      frame "Macro: Auto Flush" {
        # "Do not put any code in this frame.\n(It is a separator no-op. You can make a copy of this frame to create a new Macro frame)"
        n404 = call <vilib>:"Add State(s) to Queue__jki_lib_state_machine.vi"("State(s) in Front (\"\")"="UI: Cursor Set>>Busy\nUI: Status>>Stopping Image capture\nProcess: Stop Image capture\nUI: Status>>Requesting F3 Status\nMega: Request status>>RFB\nUI: Status>>Sending barcode\nMega: Send Barcode\nUI: Status>>Requesting F3 status\nMega: Request status>>RFF\nUI: Status>>Flushing\nMacro: Cycle valve\nUno: Validate Valve Pos>>Close\nUI: Status>>Filling Cuvett\nPump: Response>>Status\nPump: Dispense\nUI: Status>>Sending F3 Home\nMega: Return Home\nMega: Request status>>RFB\nPump: Response>>Status\nPump: Prime\nUI: Status>>Starting Image capture\nProcess: Start Image capture\nUI: Cursor Set>>Idle" ("State(s) in Front (\"\")"), "State(s) in (\"\")"=w773) -> ("States Out"=w772:string)  [unwired: 13 in]
      }
      frame "Macro: Cycle Valve" {
        # "Do not put any code in this frame.\n(It is a separator no-op. You can make a copy of this frame to create a new Macro frame)"
        n405 = call <vilib>:"Add State(s) to Queue__jki_lib_state_machine.vi"("State(s) in Front (\"\")"="UI: Cursor Set>>Busy\nUno: Valve Open\nProcess: Delay>>10000\nUno: Valve Close\nUI: Cursor Set>>Idle" ("State(s) in Front (\"\")"), "State(s) in (\"\")"=w778) -> ("States Out"=w777:string)  [unwired: 13 in]
      }
      frame "Macro: Tjek and empty" {
        # "Do not put any code in this frame.\n(It is a separator no-op. You can make a copy of this frame to create a new Macro frame)"
        n406 = Unbundle By Name(w781) -> ("Kuvette Full"=w780:bool, "Arduino ISS.Phase3"=w779:bool)
        n407 = case shown="True" w780 {
          tunnel: ["" ("State(s) in Front (\"\")") w788] -> w782
          tunnel: w779 -> [_ w787]
          frame False {
          }
          frame True {
            n408 = case shown="True" w787 {
              tunnel: ["Uno: Valve Open\nProcess: Delay>>2000" ("State(s) in Front (\"\")") "Mega: Request status>>RFB\nMega: Send Barcode>>30\nMega: Request status>>RFF\nUno: Valve Open\nProcess: Delay>>2000" ("State(s) in Front (\"\")")] -> w788
              frame False {
                n409 = One Button Dialog(message="Ready for Valve open?") -> ()  [unwired: 1 in, 1 out]
              }
              frame True {
              }
            }
          }
        }
        n410 = call <vilib>:"Add State(s) to Queue__jki_lib_state_machine.vi"("State(s) in Front (\"\")"=w782, "State(s) in (\"\")"=w785) -> ("States Out"=w784:string)  [unwired: 13 in]
      }
      frame "Macro: Exit" {
        # "Exit Macro\n(This is called once, when the VI exits)"
        n411 = Unbundle By Name(w792) -> ("Core JKI.Close Panel on Exit?"=w796:bool)
        n412 = call <vilib>:"Conditional State String__jki_lib_state_machine.vi"("Do State(s)?"=w796, "State"="UI: Front Panel State >> Close") -> ("State Out"=w795:string)  [unwired: 7 in]
        n413 = call <vilib>:"Add State(s) to Queue__jki_lib_state_machine.vi"("State(s) in Front (\"\")"="UI: Cursor Set>>Busy\nUI: Status>>Tjeck and empty Kuvette\nMacro: Tjek and empty\nUI: Status>>Empty pump\nPump: Empty\nUI: Status>>Save settings\nData: Save Settings\nUI: Status>>Uno Uninitialize\nUno: Uninitialize>>Exit\nUI: Status>>Pump Uninitialize\nPump: Uninitialize\nUI: Status>>Mega Uninitialize\nMega: Return Home\nMega: Uninitialize>>Exit\nUI: Status>>Cam Uninitialize\nCam: Uninitialize\nData: Cleanup\nUI: Status>>Goodbye\nUI: Cursor Set>>Idle\nUI: Uninitialize" ("State(s) in Front (\"\")"), "State(s) in (\"\")"=w795, "State(s) at Back (\"\")"="Exit") -> ("States Out"=w799:string)  [unwired: 12 in]
        n414 = call <vilib>:"Add State(s) to Queue__jki_lib_state_machine.vi"("State(s) in Front (\"\")"=w799, "State(s) in (\"\")"=w801) -> ("States Out"=w800:string)  [unwired: 13 in]
      }
      frame "---------- Process ----------" {
        # "Template Separator\n(You can make a copy of, or modify, this frame)"
        n415 = call <vilib>:"Add State(s) to Queue__jki_lib_state_machine.vi"("State(s) in (\"\")"=w805) -> ("States Out"=w804:string)  [unwired: 14 in]
      }
      frame "Process: Start Image capture" {
        # "Template Separator\n(You can make a copy of, or modify, this frame)"
        n416 = call "Calibration_Load_2.0.vi"("Data"=w810) -> ("Next state"=w807:string, "Calibration error?"=w808:bool, "Data Out"=w809:T4)  [unwired: 2 in]
        n417 = case shown="False" w808 {
          tunnel: [w824 w832] -> w813
          tunnel: w812 -> [w823 w832]
          tunnel: [w818 w831] -> w811
          tunnel: w809 -> [w821 w831]
          frame False {
            w817 = TRUE ("Image_Capture")
            n418 = Unbundle By Name(w821) -> ("Arduino SRS.Pinch-valve"=w825:refnum<visa-resource-name>)
            n419 = call "Capture_Save_Initialize_2.0.vi"("Data"=w821) -> ("output cluster"=w819:T4)
            n420 = VISA Clear(VISA resource name=w825, error in (no error)=w823) -> (VISA resource name out=w829:refnum<visa-resource-name>, error out=w826:errorcluster)
            n421 = property on="Stop Image Capture" class="Bool"("DisabledEnum"=T7."Enabled" ("Disabled")) -> ()  [unwired: 2 in, 2 out]
            n422 = property on="Start Image Capture" class="Bool"("DisabledEnum"=T7."Disabled and Grayed Out" ("Disabled")) -> ()  [unwired: 2 in, 2 out]
            n423 = local write "Ready"(w817) -> ()
            n424 = VISA Write(VISA resource name=w829, write buffer="105", error in (no error)=w826) -> (error out=w828:errorcluster)  [unwired: 2 out]
            n425 = Bundle By Name(cluster=w819, "Img_Capt"=w817, "Auto Flush"="Auto Flush") -> (w818:T4)
            n426 = call "Stall Data Flow.vim"("value in"=w828, "milliseconds to wait"=u32 2005) -> ("value out"=w824:errorcluster)  [unwired: 1 out]
            "Active" <- w817
          }
          frame True {
          }
        }
        n427 = call <vilib>:"Add State(s) to Queue__jki_lib_state_machine.vi"("State(s) in Front (\"\")"=w807, "State(s) in (\"\")"=w815, "State(s) at Back (\"\")"="UI: Status>>Capture Active" ("State(s) at Back (\"\")")) -> ("States Out"=w814:string)  [unwired: 12 in]
      }
      frame "Process: Stop Image capture" {
        w833 = FALSE ("Image_Capture")
        # "Template Separator\n(You can make a copy of, or modify, this frame)"
        n428 = Unbundle By Name(w840) -> ("Auto Flush"=w836:bool, "Arduino SRS.Pinch-valve"=w842:refnum<visa-resource-name>)
        n429 = VISA Clear(VISA resource name=w842, error in (no error)=w843) -> (VISA resource name out=w845:refnum<visa-resource-name>, error out=w848:errorcluster)
        n430 = case shown="False" w836 {
          frame False {
            n431 = local write "Active"(FALSE ("Active")) -> ()
            n432 = property on="Start Image Capture" class="Bool"("DisabledEnum"=T7."Enabled" ("Disabled")) -> ()  [unwired: 2 in, 2 out]
          }
          frame True {
          }
        }
        n433 = property on="Stop Image Capture" class="Bool"("DisabledEnum"=T7."Disabled and Grayed Out" ("Disabled")) -> ()  [unwired: 2 in, 2 out]
        n434 = VISA Write(VISA resource name=w845, write buffer="106", error in (no error)=w848) -> (error out=w846:errorcluster)  [unwired: 2 out]
        n435 = call "Stall Data Flow.vim"("value in"=w846, "milliseconds to wait"=u32 4000) -> ("value out"=w838:errorcluster)  [unwired: 1 out]
        n436 = call "Image_Acquisition_Stop_2.0.vi"("error in"=w838, "Data"=w840) -> ("error out"=w837:errorcluster, "Data 2"=w839:T4)  [unwired: 1 in]
        n437 = local write "Ready"(w833) -> ()
        n438 = Bundle By Name(cluster=w839, "Img_Capt"=w833) -> (w841:T4)
        n439 = call <vilib>:"Add State(s) to Queue__jki_lib_state_machine.vi"("State(s) in (\"\")"=w850, "State(s) at Back (\"\")"="UI: Status>>Capture Stopped" ("State(s) at Back (\"\")")) -> ("States Out"=w849:string)  [unwired: 13 in]
      }
      frame "Process: Identify Serial Communication" {
        # "Template Separator\n(You can make a copy of, or modify, this frame)"
        n440 = call "ID_Connection_2.0.vi"() -> (2:"Arduino Uno"=w869:refnum<visa-resource-name>, 3:"Arduino Uno"=w868:string, 4:"Arduino Uno"=w862:bool, 6:"Pump"=w867:refnum<visa-resource-name>, 8:"Pump"=w866:string, 10:"Pump"=w858:bool, 13:"Arduino Mega"=w863:bool, 14:"Arduino Mega"=w864:string, 15:"Arduino Mega"=w865:refnum<visa-resource-name>)  [unwired: 7 in]
        "Valve" <- w862
        "Pump" <- w858
        "Phase 3" <- w863
        n441 = call-poly <vilib>:"Select State(s)__jki_lib_state_machine.vi"("State(s) if True (\"\")"="UI: Status>>Valve Initiated" ("State(s) if False (\"\")"), "Select"=w862, "State(s) if False (\"\")"="UI: Status>>Valve connection failed\nUno: Initialize" ("State(s) if True (\"\")")) -> ("States Out"=w855:string)  [unwired: 12 in]
        n442 = case shown="True" w863 {
          tunnel: ["UI: Status>>F3 Connection failed" ("State(s) at Back (\"\")") "UI: Status>>F3 Initiated\nMega: Scan Barcodes" ("State(s) at Back (\"\")")] -> w853
          frame False {
          }
          frame True {
            n443 = property on="Auto Flush" class="Bool (strict)"("DisabledEnum"=T7."Enabled" ("Disabled")) -> ()  [unwired: 2 in, 2 out]
          }
        }
        n444 = Bundle By Name(cluster=w871, "Arduino SRS.Pinch-valve"=w869, "Arduino SRS.Arduino Uno"=w868, "Arduino SRS.Actuator"=w862, "Pump.Port"=w867, "Pump.Pump"=w866, "Pump.Connection"=w858, "Arduino ISS.Mega F3"=w865, "Arduino ISS.Arduino Mega"=w864, "Arduino ISS.Phase3"=w863) -> (w870:T4)
        n445 = call-poly <vilib>:"Select State(s)__jki_lib_state_machine.vi"("State(s) if True (\"\")"="UI: Status>>Setting pump values\nPump: Conditions Check" ("State(s) if True (\"\")"), "Select"=w858, "State(s) if False (\"\")"="UI: Status>>Pump connection failed" ("State(s) if False (\"\")")) -> ("States Out"=w854:string)  [unwired: 12 in]
        n446 = call <vilib>:"Add State(s) to Queue__jki_lib_state_machine.vi"("State(s) in Front (\"\")"=w855, "State(s) in (\"\")"=w854, "State(s) at Back (\"\")"=w853) -> ("States Out"=w859:string)  [unwired: 12 in]
        n447 = call <vilib>:"Add State(s) to Queue__jki_lib_state_machine.vi"("State(s) in Front (\"\")"=w859, "State(s) in (\"\")"=w874) -> ("States Out"=w873:string)  [unwired: 13 in]
      }
      frame "Process: Auto Flush" {
        # "Template Separator\n(You can make a copy of, or modify, this frame)"
        n448 = case shown="\"OFF\", Default" w879 {
          tunnel: [FALSE TRUE] -> w878
          frame "OFF", Default {
          }
          frame "ON" {
          }
        }
        n449 = Bundle By Name(cluster=w881, "Auto Flush"=w878) -> (w880:T4)
        n450 = call <vilib>:"Add State(s) to Queue__jki_lib_state_machine.vi"("State(s) in (\"\")"=w884) -> ("States Out"=w883:string)  [unwired: 14 in]
      }
      frame "Process: End Auto Flush" {
        w887 = FALSE
        # "Template Separator\n(You can make a copy of, or modify, this frame)"
        n451 = Bundle By Name(cluster=w889, "Auto Flush"=w887) -> (w888:T4)
        n452 = property on="Auto Flush" class="Bool (strict)"("Value"=w887) -> ()  [unwired: 2 in, 2 out]
        n453 = call <vilib>:"Add State(s) to Queue__jki_lib_state_machine.vi"("State(s) in (\"\")"=w892) -> ("States Out"=w891:string)  [unwired: 14 in]
      }
      frame "Process: Delay" {
        # "Template Separator\n(You can make a copy of, or modify, this frame)"
        n454 = Decimal String To Number(string=w894) -> (number=w893:i32)  [unwired: 2 in, 1 out]
        n455 = call "Stall Data Flow.vim"("value in"=w896, "milliseconds to wait"=w893) -> ("value out"=w895:errorcluster)  [unwired: 1 out]
        n456 = call <vilib>:"Add State(s) to Queue__jki_lib_state_machine.vi"("State(s) in (\"\")"=w899) -> ("States Out"=w898:string)  [unwired: 14 in]
      }
      frame "Process: Stop" {
        # "Template Separator\n(You can make a copy of, or modify, this frame)"
        n457 = call <vilib>:"Add State(s) to Queue__jki_lib_state_machine.vi"("State(s) in Front (\"\")"="Process: Auto Flush>>OFF\nProcess: Stop Image capture\nUI: Enabled\nUI: Cursor Set>>Idle" ("State(s) in Front (\"\")"), "State(s) in (\"\")"=w904) -> ("States Out"=w903:string)  [unwired: 13 in]
      }
      frame "Process: Save History" {
        # "Template Separator\n(You can make a copy of, or modify, this frame)"
        n458 = Unbundle By Name(w917) -> ("Timestamp Start"=w913:string, "Status History"=w915:string)
        n459 = call <vilib>:"Application Directory.vi"() -> ("Application Directory"=w920:path)
        n460 = Path To String(path=w920) -> (string=w921:string)
        n461 = Concatenate Strings(w921, "\\StatusHistory" ("string"), "_" ("string"), w913, ".txt" ("string")) -> (w918:string)
        n462 = String To Path(string=w918) -> (path=w906:path)
        n463 = Open/Create/Replace File(file path (use dialog)=w906, error in=w905, operation (0:open)=T11."open or create") -> (refnum out=w911:refnum<file>, error out=w910:errorcluster)  [unwired: 3 in, 1 out]
        n464 = Write to Text File(file (use dialog)=w911, text=w915, error in=w910) -> (refnum out=w908:refnum<file>, error out=w909:errorcluster)  [unwired: 1 in, 1 out]
        n465 = Close File(refnum=w908, error in=w909) -> (error out=w914:errorcluster)  [unwired: 1 out]
        n466 = call <vilib>:"Add State(s) to Queue__jki_lib_state_machine.vi"("State(s) in (\"\")"=w923) -> ("States Out"=w922:string)  [unwired: 14 in]
      }
      frame "---------- Uno ----------" {
        # "Template Separator\n(You can make a copy of, or modify, this frame)"
        n467 = call <vilib>:"Add State(s) to Queue__jki_lib_state_machine.vi"("State(s) in (\"\")"=w927) -> ("States Out"=w926:string)  [unwired: 14 in]
      }
      frame "Uno: Initialize" {
        # "Your code here.\n(You can make a copy of, or modify, this frame)"
        n468 = call "Initialize_Serial_Device_2.0.vi"("error in (no error)"=w930, "Enum"=enum16{"Arduino Uno", "Pump", "Arduino Mega"}."Arduino Uno", "Data"=w933) -> ("error out"=w931:errorcluster, "Connection"=w928:bool, "Data 2"=w932:T4)  [unwired: 6 in]
        n469 = local write "Valve"(w928) -> ()
        n470 = call <vilib>:"Add State(s) to Queue__jki_lib_state_machine.vi"("State(s) in (\"\")"=w935) -> ("States Out"=w934:string)  [unwired: 14 in]
      }
      frame "Uno: Validate Valve Pos" {
        # "Template Separator\n(You can make a copy of, or modify, this frame)"
        n471 = case shown="\"Close\", Default" w938 {
          tunnel: [enum16{"Standby", "Close", "Open"}."Close" ("Expected state") enum16{"Standby", "Close", "Open"}."Open" ("Expected state")] -> w939
          frame "Close", Default {
            # "Expected state"
          }
          frame "Open" {
            # "Expected state"
          }
        }
        n472 = Unbundle By Name(w944) -> ("Auto Flush"=w943:bool)
        n473 = while {
          tunnel: [w963] -> w937
          tunnel: [w958] -> w941
          tunnel: w944 -> [w962]
          tunnel: [w966] -> w947
          tunnel: w946 -> [w965]
          tunnel: [w964] -> w945
          tunnel: w939 -> [w955]
          i -> [w961]
          stop <- w957 stop-if-true
          n474 = Wait (ms)(milliseconds to wait=u32 500) -> ()  [unwired: 1 out]
          n475 = Greater Or Equal?(x=w961, y=5) -> (x >= y?=w959:bool)
          n476 = call "Validate_Valve_pos_2.0.vi"("error in (no error)"=w965, "Expected state"=w955, "Data"=w962) -> ("error out"=w964:errorcluster, "Reported state"=w963:enum16{"Standby", "Close", "Open"}, "Valve check"=w958:bool, "output cluster"=w966:T4)  [unwired: 1 in]
          n477 = Or(x=w958, y=w959) -> (x .or. y?=w957:bool)
        }
        n478 = case shown="True" w943 {
          tunnel: w942 -> [w969 w973]
          tunnel: w941 -> [w967 w971]
          tunnel: [w970 w974] -> w940
          frame False {
            n479 = call-poly <vilib>:"Select State(s)__jki_lib_state_machine.vi"("State(s) if True (\"\")"=w969, "Select"=w967, "State(s) if False (\"\")"="UI: Status>>Valve check failed" ("State(s) if False (\"\")")) -> ("States Out"=w970:string)  [unwired: 12 in]
          }
          frame True {
            n480 = call-poly <vilib>:"Select State(s)__jki_lib_state_machine.vi"("State(s) if True (\"\")"=w973, "Select"=w971, "State(s) if False (\"\")"="UI: Status>>Valve responce didn't match\nProcess: Stop\nUI: Popup>>Valve response" ("f")) -> ("States Out"=w974:string)  [unwired: 12 in]
          }
        }
        n481 = case shown="\"Standby\", Default" w937 {
          tunnel: ["Standby" ("Current Position") "Close" ("Current Position") "Open" ("Current Position")] -> w936
          frame "Standby", Default {
            n482 = One Button Dialog(message="Valve  is reporting standby state") -> ()  [unwired: 1 in, 1 out]
          }
          frame "Close" {
          }
          frame "Open" {
          }
        }
        "Current Position" <- w936
        n483 = call <vilib>:"Add State(s) to Queue__jki_lib_state_machine.vi"("State(s) in (\"\")"=w940) -> ("States Out"=w948:string)  [unwired: 14 in]
      }
      frame "Uno: Valve Open" {
        # "Template Separator\n(You can make a copy of, or modify, this frame)"
        n484 = Unbundle By Name(w978) -> ("Arduino SRS.Pinch-valve"=w981:refnum<visa-resource-name>, "Arduino SRS.Actuator"=w976:bool)
        n485 = case shown="True" w976 {
          tunnel: w981 -> [_ w1000]
          tunnel: w980 -> [w985 w994]
          tunnel: [w985 w993] -> w979
          tunnel: w978 -> [w986 w992]
          tunnel: [w986 w991] -> w977
          tunnel: ["" ("State(s) in Front (\"\")") "UI: Status>>Valve Open" ("State(s) in Front (\"\")")] -> w975
          frame False {
          }
          frame True {
            n486 = VISA Clear(VISA resource name=w1000, error in (no error)=w994) -> (VISA resource name out=w996:refnum<visa-resource-name>, error out=w999:errorcluster)
            n487 = VISA Write(VISA resource name=w996, write buffer="102", error in (no error)=w999) -> (error out=w997:errorcluster)  [unwired: 2 out]
            n488 = call "Stall Data Flow.vim"("value in"=w997, "milliseconds to wait"=u32 2005) -> ("value out"=w993:errorcluster)  [unwired: 1 out]
            n489 = Bundle By Name(cluster=w992, "Arduino SRS.Valve state"=enum16{"Standby", "Close", "Open"}."Open", "Kuvette Full"=FALSE) -> (w991:T4)
            n490 = local write "Current Position"("Open" ("Current Position")) -> ()
          }
        }
        n491 = call <vilib>:"Add State(s) to Queue__jki_lib_state_machine.vi"("State(s) in Front (\"\")"=w975, "State(s) in (\"\")"=w983) -> ("States Out"=w982:string)  [unwired: 13 in]
      }
      frame "Uno: Valve Close" {
        # "Template Separator\n(You can make a copy of, or modify, this frame)"
        n492 = Unbundle By Name(w1004) -> ("Arduino SRS.Pinch-valve"=w1007:refnum<visa-resource-name>, "Arduino SRS.Actuator"=w1002:bool)
        n493 = case shown="True" w1002 {
          tunnel: w1007 -> [_ w1025]
          tunnel: w1006 -> [w1011 w1019]
          tunnel: [w1011 w1018] -> w1005
          tunnel: w1004 -> [w1012 w1017]
          tunnel: [w1012 w1016] -> w1003
          tunnel: ["" ("State(s) in Front (\"\")") "UI: Status>>Valve Closed" ("State(s) in Front (\"\")")] -> w1001
          frame False {
          }
          frame True {
            n494 = VISA Clear(VISA resource name=w1025, error in (no error)=w1019) -> (VISA resource name out=w1021:refnum<visa-resource-name>, error out=w1024:errorcluster)
            n495 = VISA Write(VISA resource name=w1021, write buffer="101", error in (no error)=w1024) -> (error out=w1022:errorcluster)  [unwired: 2 out]
            n496 = local write "Current Position"("Close" ("Current Position")) -> ()
            n497 = call "Stall Data Flow.vim"("value in"=w1022, "milliseconds to wait"=u32 2005) -> ("value out"=w1018:errorcluster)  [unwired: 1 out]
            n498 = Bundle By Name(cluster=w1017, "Arduino SRS.Valve state"=enum16{"Standby", "Close", "Open"}."Close") -> (w1016:T4)
          }
        }
        n499 = call <vilib>:"Add State(s) to Queue__jki_lib_state_machine.vi"("State(s) in Front (\"\")"=w1001, "State(s) in (\"\")"=w1009) -> ("States Out"=w1008:string)  [unwired: 13 in]
      }
      frame "Uno: Cam Id request" {
        # "Template Separator\n(You can make a copy of, or modify, this frame)"
        n500 = call "CAM_ID_Request_2.0.vi"("error in (no error)"=w1028, "Data"=w1029) -> ("error out"=w1027:errorcluster, "output cluster"=w1026:T4)  [unwired: 7 in, 1 out]
        n501 = call <vilib>:"Add State(s) to Queue__jki_lib_state_machine.vi"("State(s) in (\"\")"=w1031) -> ("States Out"=w1030:string)  [unwired: 14 in]
      }
      frame "Uno: System Serial and Version" {
        # "Template Separator\n(You can make a copy of, or modify, this frame)"
        n502 = Unbundle By Name(w1036) -> ("Arduino SRS.Pinch-valve"=w1037:refnum<visa-resource-name>, "Arduino SRS.Actuator"=w1034:bool)
        n503 = case shown="True" w1034 {
          tunnel: w1036 -> [w1041 w1049]
          tunnel: [w1041 w1048] -> w1035
          tunnel: w1033 -> [w1040 w1046]
          tunnel: [w1040 w1042] -> w1032
          tunnel: w1037 -> [_ w1047]
          frame False {
          }
          frame True {
            n504 = VISA Clear(VISA resource name=w1047, error in (no error)=w1046) -> (VISA resource name out=w1052:refnum<visa-resource-name>, error out=w1045:errorcluster)
            n505 = VISA Write(VISA resource name=w1052, write buffer="107", error in (no error)=w1045) -> (VISA resource name out=w1054:refnum<visa-resource-name>, error out=w1044:errorcluster)  [unwired: 1 out]
            n506 = call "Stall Data Flow.vim"("value in"=w1054, "milliseconds to wait"=u32 2005) -> ("value out"=w1051:refnum<visa-resource-name>)  [unwired: 1 out]
            n507 = property class="Instr"(reference=w1051, error in=w1044) -> (reference out=w1056:refnum<visa-resource-name>, error out=w1043:errorcluster, "Serial Settings:Number of Bytes at Serial Port"=w1057:u32)
            n508 = Greater Than 0?(x=w1057) -> (x > 0?=w1055:bool)
            n509 = case shown="True" w1055 {
              tunnel: w1057 -> [_ w1073]
              tunnel: w1056 -> [_ w1072]
              tunnel: w1049 -> [w1059 w1069]
              tunnel: [w1059 w1068] -> w1048
              tunnel: w1043 -> [w1058 w1062]
              tunnel: [w1058 w1060] -> w1042
              frame False {
                # "No data"
              }
              frame True {
                w1065 = u16 1 items=["Standard", "XL"] ("SystemVersion")
                w1066 = u16 0 items=["Standard", "XL"] ("SystemVersion")
                # "Data available"
                n510 = VISA Read(VISA resource name=w1072, byte count=w1073, error in (no error)=w1062) -> (read buffer=w1063:string, error out=w1061:errorcluster)  [unwired: 2 out]
                "read buffer 2" <- w1063
                n511 = xnode "Match Regular Expression"("input string"=w1063, "regular expression"="XL", "error in"=w1061) -> ("offset past match"=w1070:i32, "error out"=w1060:errorcluster)  [unwired: 3 in, 3 out]
                n512 = Greater Than 0?(x=w1070) -> (x > 0?=w1067:bool)
                n513 = Select(t=w1065, s=w1067, f=w1066) -> (s? t:f=w1064:u16)
                n514 = Bundle By Name(cluster=w1069, "System Serial"=w1063, "SystemVersion"=w1064) -> (w1068:T4)
              }
            }
          }
        }
        n515 = call <vilib>:"Add State(s) to Queue__jki_lib_state_machine.vi"("State(s) in (\"\")"=w1039) -> ("States Out"=w1038:string)  [unwired: 14 in]
      }
      frame "Uno: Send UR Go" {
        # "Template Separator\n(You can make a copy of, or modify, this frame)"
        n516 = Unbundle By Name(w1195) -> ("Arduino SRS.Pinch-valve"=w1194:refnum<visa-resource-name>, "Arduino SRS.Actuator"=w1193:bool)
        n517 = case shown="True" w1193 {
          tunnel: w1192 -> [w1198 w1208]
          tunnel: [w1198 w1199] -> w1191
          tunnel: w1194 -> [_ w1207]
          frame False {
          }
          frame True {
            n518 = VISA Clear(VISA resource name=w1207, error in (no error)=w1208) -> (VISA resource name out=w1210:refnum<visa-resource-name>, error out=w1213:errorcluster)
            n519 = VISA Write(VISA resource name=w1210, write buffer="105", error in (no error)=w1213) -> (VISA resource name out=w1206:refnum<visa-resource-name>, error out=w1211:errorcluster)  [unwired: 1 out]
            n520 = call "Stall Data Flow.vim"("value in"=w1211, "milliseconds to wait"=u32 2005) -> ("value out"=w1205:errorcluster)  [unwired: 1 out]
            n521 = property class="Instr"(reference=w1206, error in=w1205) -> (reference out=w1203:refnum<visa-resource-name>, error out=w1202:errorcluster, "Serial Settings:Number of Bytes at Serial Port"=w1200:u32)
            n522 = Not Equal?(x=w1200, y=u32 0) -> (x != y?=w1201:bool)
            n523 = case shown="True" w1201 {
              tunnel: w1200 -> [_ w1220]
              tunnel: w1203 -> [_ w1219]
              tunnel: w1202 -> [w1215 w1218]
              tunnel: [w1215 w1217] -> w1199
              tunnel: ["" ("read buffer") w1216] -> _
              frame False {
                # "No data"
              }
              frame True {
                # "Data available"
                n524 = VISA Read(VISA resource name=w1219, byte count=w1220, error in (no error)=w1218) -> (read buffer=w1216:string, error out=w1217:errorcluster)  [unwired: 2 out]
              }
            }
          }
        }
        n525 = call <vilib>:"Add State(s) to Queue__jki_lib_state_machine.vi"("State(s) in (\"\")"=w1197) -> ("States Out"=w1196:string)  [unwired: 14 in]
      }
      frame "Uno: Send UR Halt" {
        # "Template Separator\n(You can make a copy of, or modify, this frame)"
        n526 = Unbundle By Name(w1225) -> ("Arduino SRS.Pinch-valve"=w1224:refnum<visa-resource-name>, "Arduino SRS.Actuator"=w1223:bool)
        n527 = case shown="True" w1223 {
          tunnel: w1222 -> [w1228 w1238]
          tunnel: [w1228 w1229] -> w1221
          tunnel: w1224 -> [_ w1237]
          frame False {
          }
          frame True {
            n528 = VISA Clear(VISA resource name=w1237, error in (no error)=w1238) -> (VISA resource name out=w1240:refnum<visa-resource-name>, error out=w1243:errorcluster)
            n529 = VISA Write(VISA resource name=w1240, write buffer="106", error in (no error)=w1243) -> (VISA resource name out=w1236:refnum<visa-resource-name>, error out=w1241:errorcluster)  [unwired: 1 out]
            n530 = call "Stall Data Flow.vim"("value in"=w1241, "milliseconds to wait"=u32 2005) -> ("value out"=w1235:errorcluster)  [unwired: 1 out]
            n531 = property class="Instr"(reference=w1236, error in=w1235) -> (reference out=w1233:refnum<visa-resource-name>, error out=w1232:errorcluster, "Serial Settings:Number of Bytes at Serial Port"=w1230:u32)
            n532 = Not Equal?(x=w1230, y=u32 0) -> (x != y?=w1231:bool)
            n533 = case shown="True" w1231 {
              tunnel: w1230 -> [_ w1250]
              tunnel: w1233 -> [_ w1249]
              tunnel: w1232 -> [w1245 w1248]
              tunnel: [w1245 w1247] -> w1229
              tunnel: ["" ("read buffer") w1246] -> _
              frame False {
                # "No data"
              }
              frame True {
                # "Data available"
                n534 = VISA Read(VISA resource name=w1249, byte count=w1250, error in (no error)=w1248) -> (read buffer=w1246:string, error out=w1247:errorcluster)  [unwired: 2 out]
              }
            }
          }
        }
        n535 = call <vilib>:"Add State(s) to Queue__jki_lib_state_machine.vi"("State(s) in (\"\")"=w1227) -> ("States Out"=w1226:string)  [unwired: 14 in]
      }
      frame "Uno: Report Temp and Fan Data" {
        # "Template Separator\n(You can make a copy of, or modify, this frame)"
        n536 = Unbundle By Name(w1253) -> ("Arduino SRS.Pinch-valve"=w1251:refnum<visa-resource-name>, "Arduino SRS.Actuator"=w1252:bool)
        n537 = case shown="True" w1252 {
          tunnel: w1255 -> [w1258 w1268]
          tunnel: [w1258 w1259] -> w1254
          tunnel: w1251 -> [_ w1267]
          frame False {
          }
          frame True {
            n538 = VISA Clear(VISA resource name=w1267, error in (no error)=w1268) -> (VISA resource name out=w1270:refnum<visa-resource-name>, error out=w1273:errorcluster)
            n539 = VISA Write(VISA resource name=w1270, write buffer="106", error in (no error)=w1273) -> (VISA resource name out=w1266:refnum<visa-resource-name>, error out=w1271:errorcluster)  [unwired: 1 out]
            n540 = call "Stall Data Flow.vim"("value in"=w1271, "milliseconds to wait"=u32 2005) -> ("value out"=w1265:errorcluster)  [unwired: 1 out]
            n541 = property class="Instr"(reference=w1266, error in=w1265) -> (reference out=w1263:refnum<visa-resource-name>, error out=w1262:errorcluster, "Serial Settings:Number of Bytes at Serial Port"=w1260:u32)
            n542 = Not Equal?(x=w1260, y=u32 0) -> (x != y?=w1261:bool)
            n543 = case shown="True" w1261 {
              tunnel: w1260 -> [_ w1280]
              tunnel: w1263 -> [_ w1279]
              tunnel: w1262 -> [w1275 w1278]
              tunnel: [w1275 w1277] -> w1259
              tunnel: ["" ("read buffer") w1276] -> _
              frame False {
                # "No data"
              }
              frame True {
                # "Data available"
                n544 = VISA Read(VISA resource name=w1279, byte count=w1280, error in (no error)=w1278) -> (read buffer=w1276:string, error out=w1277:errorcluster)  [unwired: 2 out]
              }
            }
          }
        }
        n545 = call <vilib>:"Add State(s) to Queue__jki_lib_state_machine.vi"("State(s) in (\"\")"=w1257) -> ("States Out"=w1256:string)  [unwired: 14 in]
      }
      frame "Uno: Uninitialize" {
        # "Your code here.\n(You can make a copy of, or modify, this frame)"
        n546 = Unbundle By Name(w1283) -> ("Arduino SRS.Pinch-valve"=w1286:refnum<visa-resource-name>, "Arduino SRS.Actuator"=w1287:bool)
        n547 = case shown="True" w1287 {
          tunnel: w1286 -> [_ w1297]
          tunnel: w1285 -> [w1291 w1296]
          tunnel: [w1291 w1295] -> w1284
          tunnel: w1283 -> [w1290 w1294]
          tunnel: [w1290 w1293] -> w1282
          tunnel: w1281 -> [_ w1292]
          frame False {
          }
          frame True {
            n548 = case shown="\"Exit\"" w1292 {
              tunnel: w1297 -> [_ w1308]
              tunnel: w1296 -> [w1299 w1307]
              tunnel: [w1299 w1306] -> w1295
              tunnel: w1294 -> [w1301 w1305]
              tunnel: [w1300 w1304] -> w1293
              frame "", Default {
                w1302 = FALSE ("Arduino SRS.Actuator")
                n549 = local write "Valve"(w1302) -> ()
                n550 = Bundle By Name(cluster=w1301, "Arduino SRS.Pinch-valve"=refnum<visa-resource-name> refnum, "Arduino SRS.Actuator"=w1302) -> (w1300:T4)
              }
              frame "Exit" {
                w1303 = FALSE ("Arduino SRS.Actuator")
                n551 = VISA Close(VISA resource name=w1308, error in (no error)=w1307) -> (error out=w1306:errorcluster)
                n552 = local write "Valve"(w1303) -> ()
                n553 = Bundle By Name(cluster=w1305, "Arduino SRS.Actuator"=w1303) -> (w1304:T4)
              }
            }
          }
        }
        n554 = call <vilib>:"Add State(s) to Queue__jki_lib_state_machine.vi"("State(s) in (\"\")"=w1289) -> ("States Out"=w1288:string)  [unwired: 14 in]
      }
      frame "---------- Pump ----------" {
        # "Template Separator\n(You can make a copy of, or modify, this frame)"
        n555 = call <vilib>:"Add State(s) to Queue__jki_lib_state_machine.vi"("State(s) in (\"\")"=w1312) -> ("States Out"=w1311:string)  [unwired: 14 in]
      }
      frame "Pump: Initialize" {
        # "Template Separator\n(You can make a copy of, or modify, this frame)"
        n556 = call "Initialize_Serial_Device_2.0.vi"("error in (no error)"=w1318, "Enum"=enum16{"Arduino Uno", "Pump", "Arduino Mega"}."Pump", "Data"=w1321) -> ("error out"=w1319:errorcluster, "Connection"=w1316:bool, "Data 2"=w1320:T4)  [unwired: 6 in]
        n557 = local write "Pump"(w1316) -> ()
        n558 = call-poly <vilib>:"Select State(s)__jki_lib_state_machine.vi"("State(s) if True (\"\")"="UI: Status>>Pump Initiated\nPump: Conditions Check" ("State(s) if True (\"\")"), "Select"=w1316, "State(s) if False (\"\")"="UI: Status>>Pump initiazion failed" ("State(s) if False (\"\")")) -> ("States Out"=w1313:string)  [unwired: 12 in]
        n559 = call <vilib>:"Add State(s) to Queue__jki_lib_state_machine.vi"("State(s) in Front (\"\")"=w1313, "State(s) in (\"\")"=w1323) -> ("States Out"=w1322:string)  [unwired: 13 in]
      }
      frame "Pump: Ask for size" {
        # "Template Separator\n(You can make a copy of, or modify, this frame)"
        n560 = call <vilib>:"Three Button Dialog.vi"("Allow user to close window? (TRUE)"=TRUE, "Window Title (\"\")"="Pump Size" ("Window Title (\"\")"), "Right Button Text (\"Cancel\")"="None" ("Right Button Text (\"Cancel\")"), "Center Button Text (\"No\")"="Small" ("Center Button Text (\"No\")"), "Left Button Text (\"Yes\")"="Large" ("Left Button Text (\"Yes\")"), "message"="What size Pump is connected to the system?") -> ("Which Button?"=w1325:T14)  [unwired: 5 in]
        n561 = case shown="\"Center Button\"" w1325 {
          tunnel: [enum16{"None", "Small", "Large"}."None" ("Pump.Pump Size") enum16{"None", "Small", "Large"}."Large" ("Pump.Pump Size") enum16{"None", "Small", "Large"}."Small" ("Pump.Pump Size") enum16{"None", "Small", "Large"}."None" ("Pump.Pump Size")] -> w1324
          frame "Window Close", Default {
          }
          frame "Left Button" {
          }
          frame "Center Button" {
          }
          frame "Right Button" {
          }
        }
        n562 = Bundle By Name(cluster=w1333, "Pump.Pump Size"=w1324) -> (w1332:T4)
        n563 = call <vilib>:"Add State(s) to Queue__jki_lib_state_machine.vi"("State(s) in (\"\")"=w1336) -> ("States Out"=w1335:string)  [unwired: 14 in]
      }
      frame "Pump: Conditions Check" {
        # "Template Separator\n(You can make a copy of, or modify, this frame)"
        n564 = Two Button Dialog(message="Are all of the  following statements TRUE?\n1. The kuvett CLOSED.\n2. The kuvett is EMPTY.\n3. The pump is EMPTY.", 1:"NO!" ("F button name (\"Cancel\")"), 2:"Yes" ("T button name (\"OK\")")) -> (T button?=w1344:bool)
        n565 = case shown="False" w1344 {
          tunnel: w1343 -> [w1357 w1413]
          tunnel: [w1356 w1412] -> w1342
          tunnel: [w1355 "Pump: Start Pump\nProcess: Delay>>500\nPump: Response>>Status\nPump: Prime\nProcess: Delay>>2000\nPump: Response>>Status\nPump: Dispense" ("State(s) if False (\"\")")] -> w1341
          frame False {
            n566 = call "Pump_Conditions_Check.vi"() -> ("OK"=w1354:bool, "K_Empty Out"=w1353:bool, "K_Closed Out"=w1352:bool, "P_Empty Out"=w1351:bool)  [unwired: 4 in]
            n567 = disable-structure shown="Enabled" {
              disable-tunnel: w1357 -> [w1361 w1387]
              disable-tunnel: [w1360 w1383] -> w1356
              disable-tunnel: [w1358 w1382] -> w1355
              disable-tunnel: w1354 -> [_ w1388]
              disable-tunnel: w1353 -> [_ w1386]
              disable-tunnel: w1352 -> [_ w1385]
              disable-tunnel: w1351 -> [_ w1384]
              frame Disabled {
                n568 = Two Button Dialog(message="Is the kuvett Open?", 1:"No" ("F button name (\"Cancel\")"), 2:"YES!" ("T button name (\"OK\")")) -> (T button?=w1359:bool)
                n569 = case shown="False" w1359 {
                  tunnel: w1361 -> [w1368 w1381]
                  tunnel: [w1366 w1380] -> w1360
                  tunnel: [w1365 "Pump: Start Pump" ("State(s) if True (\"\")")] -> w1358
                  frame False {
                    n570 = Two Button Dialog(message="Is the kuvett Full?", 1:"No" ("F button name (\"Cancel\")"), 2:"YES!" ("T button name (\"OK\")")) -> (T button?=w1367:bool)
                    n571 = case shown="True" w1367 {
                      selector: w1367 -> [_ w1376]
                      tunnel: w1368 -> [w1373 w1377]
                      tunnel: [w1373 w1375] -> w1366
                      tunnel: ["UI: Status>>JackAss\nPump: Start Pump\nPrecess: Delay>>500\nPump: Response>>Status\nPump: Prime\nPump: Response>>Status\nPump: Dispense" ("State(s) if True (\"\")") "Pump: Start Pump" ("State(s) if True (\"\")")] -> w1365
                      frame False {
                      }
                      frame True {
                        n572 = Bundle By Name(cluster=w1377, "Kuvette Full"=w1376) -> (w1375:T4)
                      }
                    }
                  }
                  frame True {
                    n573 = Bundle By Name(cluster=w1381, "Arduino SRS.Valve state"=enum16{"Standby", "Close", "Open"}."Open") -> (w1380:T4)
                  }
                }
              }
              frame Enabled {
                n574 = case shown="True" w1388 {
                  tunnel: w1387 -> [w1394 w1402]
                  tunnel: w1386 -> [_ w1398]
                  tunnel: w1385 -> [_ w1401]
                  tunnel: w1384 -> [_ w1395]
                  tunnel: [w1390 w1396] -> w1383
                  tunnel: ["" ("State(s) if True (\"\")") w1400] -> w1382
                  frame False {
                    n575 = Bundle By Name(cluster=w1394, "Arduino SRS.Valve state"=enum16{"Standby", "Close", "Open"}."Standby", "Kuvette Full"=TRUE, "Pump.Connection"=FALSE) -> (w1390:T4)
                  }
                  frame True {
                    n576 = Not(x=w1398) -> (.not. x?=w1397:bool)
                    n577 = case shown="False" w1401 {
                      tunnel: [enum16{"Standby", "Close", "Open"}."Open" ("Arduino SRS.Valve state") enum16{"Standby", "Close", "Open"}."Close" ("Arduino SRS.Valve state")] -> w1399
                      frame False {
                      }
                      frame True {
                      }
                    }
                    n578 = Bundle By Name(cluster=w1402, "Arduino SRS.Valve state"=w1399, "Kuvette Full"=w1397, "Pump.Connection"=w1395) -> (w1396:T4)
                    n579 = local write "Pump"(w1395) -> ()
                    n580 = case shown="True" w1395 {
                      tunnel: ["Uno: Valve Close\nProcess: Delay>>500\nPump: Start Pump\nProcess: Delay>>500\nPump: Response>>Status\nMacro: Tjek and empty\nUno: Valve Close\nPump: Prime\nProcess: Delay>>2000\nPump: Response>>Status\nPump: Dispense" ("State(s) if True (\"\")") w1404] -> w1400
                      tunnel: w1398 -> [_ w1405]
                      frame False {
                      }
                      frame True {
                        n581 = case shown="False" w1405 {
                          tunnel: ["Macro: Tjek and empty\nUno: Valve Close\nPump: Start Pump\nProcess: Delay>>500\nPump: Response>>Status\nUno: Valve Close\nPump: Prime\nProcess: Delay>>2000\nPump: Response>>Status\nPump: Dispense" ("State(s) if True (\"\")") "Pump: Start Pump\nProcess: Delay>>500\nPump: Response>>Status\nPump: Prime\nProcess: Delay>>2000\nPump: Response>>Status\nPump: Dispense" ("State(s) if False (\"\")")] -> w1404
                          frame False {
                          }
                          frame True {
                          }
                        }
                      }
                    }
                  }
                }
              }
            }
          }
          frame True {
            n582 = Bundle By Name(cluster=w1413, "Kuvette Full"=FALSE, "Arduino SRS.Valve state"=enum16{"Standby", "Close", "Open"}."Close") -> (w1412:T4)
          }
        }
        n583 = call <vilib>:"Add State(s) to Queue__jki_lib_state_machine.vi"("State(s) in Front (\"\")"=w1341, "State(s) in (\"\")"=w1350) -> ("States Out"=w1349:string)  [unwired: 13 in]
      }
      frame "Pump: Start Pump" {
        (unwired) "OS20A1000IA0" ("write buffer 2")
        (unwired) "/1OS20A1000IA0" ("write buffer 2")
        # "Pumps just a little bit to refil\nthe hoses. otherwise there \nwhont be enougth in a regular\npump cycle."
        # "<I> Input valve\n<A> Absolute position (n = 1...1000)\n<O> Output valve\n<R> Execute commands\n<T> Abort commands"
        # "Template Separator\n(You can make a copy of, or modify, this frame)"
        n584 = Unbundle By Name(w1418) -> ("Pump.Port"=w1419:refnum<visa-resource-name>, "Pump.Pump Size"=w1420:enum16{"None", "Small", "Large"}, "Pump.Connection"=w1416:bool)
        n585 = case shown="True" w1416 {
          tunnel: w1422 -> [w1427 w1431]
          tunnel: [w1427 w1429] -> w1421
          tunnel: w1420 -> [_ w1434]
          tunnel: w1419 -> [_ w1430]
          tunnel: w1418 -> [w1426 w1433]
          tunnel: [w1426 w1432] -> w1417
          tunnel: ["" ("State(s) in Front (\"\")") w1428] -> w1415
          frame False {
          }
          frame True {
            n586 = case shown="\"Large\"" w1434 {
              tunnel: w1433 -> [w1437 w1451 w1458]
              tunnel: [w1437 w1450 w1468] -> w1432
              tunnel: w1431 -> [w1436 w1442 w1463]
              tunnel: w1430 -> [_ w1440 w1465]
              tunnel: [w1436 w1438 w1455] -> w1429
              tunnel: ["" ("State(s) in Front (\"\")") "UI: Status>>Large pump started" ("State(s) in Front (\"\")") "UI: Status>>Small Pump Started" ("State(s) in Front (\"\")")] -> w1428
              frame "None", Default {
              }
              frame "Large" {
                n587 = Bundle By Name(cluster=w1451, "Kuvette Full"=FALSE, "Pump.Flush Size"=0) -> (w1450:T4)
                n588 = Concatenate Strings("/1Z20,2,2", "I1" ("string"), "S20A600" ("string"), "I2" ("string"), "A0" ("string"), "O1" ("string"), "R" ("string"), "\r\n") -> (w1441:string)
                n589 = VISA Write(VISA resource name=w1440, write buffer=w1441, error in (no error)=w1442) -> (error out=w1438:errorcluster)  [unwired: 2 out]
              }
              frame "Small" {
                n590 = Bundle By Name(cluster=w1458, "Kuvette Full"=FALSE, "Pump.Flush Size"=0) -> (w1468:T4)
                n591 = Concatenate Strings("/1Y5", "IS20A500" ("string"), "OA0" ("string"), "I" ("string"), "R" ("string"), "\r\n") -> (w1464:string)
                n592 = VISA Write(VISA resource name=w1465, write buffer=w1464, error in (no error)=w1463) -> (error out=w1455:errorcluster)  [unwired: 2 out]
              }
            }
          }
        }
        n593 = call <vilib>:"Add State(s) to Queue__jki_lib_state_machine.vi"("State(s) in Front (\"\")"=w1415, "State(s) in (\"\")"=w1424) -> ("States Out"=w1423:string)  [unwired: 13 in]
      }
      frame "Pump: Command" {
        # "Template Separator\n(You can make a copy of, or modify, this frame)"
        n594 = Unbundle By Name(w1475) -> ("Pump.Port"=w1480:refnum<visa-resource-name>, "Pump.Command"=w1479:string, "Pump.Connection"=w1473:bool, "Kuvette Full"=w1476:bool, "Pump.Ready"=w1470:bool)
        n595 = Not(x=w1476) -> (.not. x?=w1472:bool)
        n596 = Compound Arithmetic op=AND(w1473, w1472, w1470) -> (w1471:bool)
        n597 = case shown="True" w1471 {
          tunnel: w1480 -> [_ w1492]
          tunnel: w1479 -> [_ w1491]
          tunnel: w1478 -> [w1484 w1489]
          tunnel: [w1484 w1488] -> w1477
          tunnel: w1475 -> [w1483 w1487]
          tunnel: [w1483 w1486] -> w1474
          frame False {
          }
          frame True {
            n598 = Concatenate Strings("/1S20" ("string"), w1491, "\r\n") -> (w1493:string)
            n599 = Bundle By Name(cluster=w1487, "Kuvette Full"=TRUE) -> (w1486:T4)
            n600 = VISA Write(VISA resource name=w1492, write buffer=w1493, error in (no error)=w1489) -> (error out=w1488:errorcluster)  [unwired: 2 out]
          }
        }
        n601 = call <vilib>:"Add State(s) to Queue__jki_lib_state_machine.vi"("State(s) in (\"\")"=w1482) -> ("States Out"=w1481:string)  [unwired: 14 in]
      }
      frame "Pump: Dispense" {
        # "Template Separator\n(You can make a copy of, or modify, this frame)"
        n602 = Unbundle By Name(w1500) -> ("Pump.Connection"=w1498:bool, "Pump.Flush Size"=w1496:i32)
        n603 = Greater Than 0?(x=w1496) -> (x > 0?=w1495:bool)
        n604 = case shown="True" w1498 {
          tunnel: w1500 -> [w1508 w1515]
          tunnel: w1503 -> [w1507 w1514]
          tunnel: [w1508 w1513] -> w1502
          tunnel: [w1507 w1512] -> w1501
          tunnel: w1499 -> [w1505 w1511]
          tunnel: [w1504 w1510] -> w1497
          tunnel: w1495 -> [_ w1509]
          frame False {
            n605 = call <vilib>:"Add State(s) to Queue__jki_lib_state_machine.vi"("State(s) in Front (\"\")"="UI: Status>>Pump not connected" ("State(s) if False (\"\")"), "State(s) in (\"\")"=w1505) -> ("States Out"=w1504:string)  [unwired: 13 in]
          }
          frame True {
            n606 = case shown="False" w1509 {
              tunnel: w1515 -> [w1519 w1527]
              tunnel: w1514 -> [w1517 w1526]
              tunnel: [w1519 w1525] -> w1513
              tunnel: [w1517 w1523] -> w1512
              tunnel: w1511 -> [w1520 w1522]
              tunnel: [w1518 w1521] -> w1510
              frame False {
                n607 = call <vilib>:"Add State(s) to Queue__jki_lib_state_machine.vi"("State(s) in Front (\"\")"="UI: Status>>Pump not primed\nPump: Response>>Status\nPump: Prime\nProcess: Delay>>500\nPump: Response>>Status\nPump: Dispense" ("State(s) in Front (\"\")"), "State(s) in (\"\")"=w1520) -> ("States Out"=w1518:string)  [unwired: 13 in]
              }
              frame True {
                n608 = call "Pump_Dispense_Command.vi"("error"=w1526, "Data"=w1527) -> ("value out"=w1523:errorcluster, "Status Out"=w1524:string, "Data 2"=w1525:T4)  [unwired: 2 in]
                n609 = call <vilib>:"Add State(s) to Queue__jki_lib_state_machine.vi"("State(s) in Front (\"\")"=w1524, "State(s) in (\"\")"=w1522) -> ("States Out"=w1521:string)  [unwired: 13 in]
              }
            }
          }
        }
      }
      frame "Pump: Prime" {
        # "Template Separator\n(You can make a copy of, or modify, this frame)"
        n610 = Unbundle By Name(w1530) -> ("Pump.Connection"=w1529:bool)
        n611 = case shown="True" w1529 {
          tunnel: w1530 -> [w1539 w1546]
          tunnel: w1534 -> [w1538 w1545]
          tunnel: [w1539 w1543] -> w1533
          tunnel: [w1538 w1544] -> w1532
          tunnel: w1531 -> [w1536 w1541]
          tunnel: [w1535 w1540] -> w1528
          frame False {
            n612 = call <vilib>:"Add State(s) to Queue__jki_lib_state_machine.vi"("State(s) in Front (\"\")"="UI: Status>>Pump not connected" ("State(s) if False (\"\")"), "State(s) in (\"\")"=w1536) -> ("States Out"=w1535:string)  [unwired: 13 in]
          }
          frame True {
            n613 = call "Pump_Prime_Command.vi"("error"=w1545, "Data"=w1546) -> ("value out"=w1544:errorcluster, "Status Out"=w1542:string, "Data 2"=w1543:T4)  [unwired: 2 in]
            n614 = call <vilib>:"Add State(s) to Queue__jki_lib_state_machine.vi"("State(s) in Front (\"\")"=w1542, "State(s) in (\"\")"=w1541) -> ("States Out"=w1540:string)  [unwired: 13 in]
          }
        }
      }
      frame "Pump: Empty" {
        # "Template Separator\n(You can make a copy of, or modify, this frame)"
        n615 = Unbundle By Name(w1548) -> ("Pump.Connection"=w1550:bool, "Pump.Ready"=w1549:bool)
        n616 = And(x=w1550, y=w1549) -> (x .and. y?=w1551:bool)
        n617 = case shown="True" w1551 {
          tunnel: w1553 -> [w1557 w1561]
          tunnel: [w1557 w1560] -> w1552
          tunnel: w1548 -> [w1556 w1559]
          tunnel: [w1556 w1558] -> w1547
          frame False {
          }
          frame True {
            n618 = call "Pump_empty.vi"("error constant"=w1561, "input cluster"=w1559) -> ("value out"=w1560:errorcluster, "output cluster"=w1558:T4)
          }
        }
        n619 = call <vilib>:"Add State(s) to Queue__jki_lib_state_machine.vi"("State(s) in (\"\")"=w1555) -> ("States Out"=w1554:string)  [unwired: 14 in]
      }
      frame "Pump: Response" {
        # "Important There is a Ready signal saved in the buffer"
        # "Template Separator\n(You can make a copy of, or modify, this frame)"
        n620 = case shown="\"Status\"" w1574 {
          tunnel: w1575 -> [w1598 w1602]
          tunnel: [w1598 w1602] -> w1565
          tunnel: ["" w1600] -> w1563
          frame "", Default {
          }
          frame "Status" {
            n621 = Concatenate Strings("/1Q" ("string"), "\r\n") -> (w1600:string)
          }
        }
        n622 = Unbundle By Name(w1573) -> ("Auto Flush"=w1562:bool, "Pump.Port"=w1567:refnum<visa-resource-name>)
        n623 = VISA Clear(VISA resource name=w1567, error in (no error)=w1565) -> (VISA resource name out=w1566:refnum<visa-resource-name>, error out=w1564:errorcluster)
        n624 = while {
          tunnel: w1566 -> [w1596]
          tunnel: [w1587] -> w1569
          tunnel: w1563 -> [w1589]
          tunnel: [w1594] -> w1576
          tunnel: w1564 -> [w1588]
          tunnel: [w1595] -> w1577
          i -> [w1586]
          stop <- w1593 stop-if-true
          n625 = call "Pump_statusrequest.vi"("error in (no error)"=w1588, "Command"=w1589, "VISA resource name"=w1596) -> ("error out"=w1595:errorcluster, "Message"=w1594:string, "Ready"=w1587:bool)  [unwired: 3 in, 3 out]
          n626 = Greater?(x=w1586, y=100) -> (0:w1591:bool)
          n627 = Wait (ms)(milliseconds to wait=u32 500) -> ()  [unwired: 1 out]
          n628 = Or(x=w1587, y=w1591) -> (x .or. y?=w1593:bool)
        }
        n629 = Concatenate Strings("UI: Status>>Pump Response;" ("string"), w1576) -> (w1570:string)
        n630 = case shown="False" w1569 {
          tunnel: [w1582 w1585] -> w1578
          tunnel: w1570 -> [_ w1584]
          tunnel: w1568 -> [_ w1583]
          tunnel: w1562 -> [w1579 _]
          frame False {
            n631 = call-poly <vilib>:"Select State(s)__jki_lib_state_machine.vi"("State(s) if True (\"\")"="UI: Status>>Pump response error\nProcess: Stop\nUI: Popup>>Pump response" ("States Out"), "Select"=w1579, "State(s) if False (\"\")"="UI: Status>>Pump response error" ("States Out")) -> ("States Out"=w1582:string)  [unwired: 12 in]
          }
          frame True {
            n632 = call <vilib>:"Add State(s) to Queue__jki_lib_state_machine.vi"("State(s) in Front (\"\")"=w1584, "State(s) in (\"\")"=w1583) -> ("States Out"=w1585:string)  [unwired: 13 in]
          }
        }
        n633 = Bundle By Name(cluster=w1573, "Pump.Ready"=w1569) -> (w1572:T4)
      }
      frame "Pump: Uninitialize" {
        # "Template Separator\n(You can make a copy of, or modify, this frame)"
        n634 = Unbundle By Name(w1607) -> ("Pump.Port"=w1610:refnum<visa-resource-name>, "Pump.Connection"=w1611:bool, "Pump.Flush Size"=w1604:i32)
        n635 = Greater Than 0?(x=w1604) -> (x > 0?=w1605:bool)
        n636 = case shown="True" w1605 {
          tunnel: w1611 -> [w1620 _]
          tunnel: w1610 -> [w1619 _]
          tunnel: w1609 -> [w1618 w1630]
          tunnel: [w1617 w1630] -> w1608
          tunnel: w1607 -> [w1616 w1631]
          tunnel: [w1615 w1631] -> w1606
          tunnel: ["" ("State(s) in Front (\"\")") "UI: Status>>Pump is not empty\nPump: Response>>Status\nPump: Empty\nPump: Uninitialize" ("State(s) in Front (\"\")")] -> w1603
          frame False {
            n637 = case shown="True" w1620 {
              tunnel: w1619 -> [_ w1628]
              tunnel: w1618 -> [w1622 w1627]
              tunnel: [w1622 w1626] -> w1617
              tunnel: w1616 -> [w1621 w1625]
              tunnel: [w1621 w1624] -> w1615
              frame False {
              }
              frame True {
                w1623 = FALSE ("Pump.Connection")
                n638 = VISA Close(VISA resource name=w1628, error in (no error)=w1627) -> (error out=w1626:errorcluster)
                n639 = Bundle By Name(cluster=w1625, "Pump.Connection"=w1623) -> (w1624:T4)
                n640 = local write "Pump"(w1623) -> ()
              }
            }
          }
          frame True {
          }
        }
        n641 = call <vilib>:"Add State(s) to Queue__jki_lib_state_machine.vi"("State(s) in Front (\"\")"=w1603, "State(s) in (\"\")"=w1613) -> ("States Out"=w1612:string)  [unwired: 13 in]
      }
      frame "---------- Mega ----------" {
        # "Template Separator\n(You can make a copy of, or modify, this frame)"
        n642 = call <vilib>:"Add State(s) to Queue__jki_lib_state_machine.vi"("State(s) in (\"\")"=w1635) -> ("States Out"=w1634:string)  [unwired: 14 in]
      }
      frame "Mega: Initialize" {
        # "Template Separator\n(You can make a copy of, or modify, this frame)"
        n643 = call "Initialize_Serial_Device_2.0.vi"("error in (no error)"=w1646, "Enum"=enum16{"Arduino Uno", "Pump", "Arduino Mega"}."Arduino Mega", "Data"=w1645) -> ("error out"=w1641:errorcluster, "Connection"=w1643:bool, "Data 2"=w1642:T4)  [unwired: 6 in]
        n644 = case shown="True" w1643 {
          frame False {
          }
          frame True {
            n645 = property on="Auto Flush" class="Bool (strict)"("DisabledEnum"=T7."Enabled" ("Disabled")) -> ()  [unwired: 2 in, 2 out]
          }
        }
        n646 = local write "Phase 3"(w1643) -> ()
        n647 = call "Get_Status_BarcodeString_2.0.vi"("error in (no error)"=w1641, "Data"=w1642) -> ("error out"=w1640:errorcluster, "F3 Status"=w1637:string, "Data 2"=w1639:T4)  [unwired: 2 in, 1 out]
        n648 = Concatenate Strings("UI: Status>>F3 Responce; " ("string"), w1637) -> (w1636:string)
        n649 = call <vilib>:"Add State(s) to Queue__jki_lib_state_machine.vi"("State(s) in Front (\"\")"=w1636, "State(s) in (\"\")"=w1648) -> ("States Out"=w1647:string)  [unwired: 13 in]
      }
      frame "Mega: Test Air system" {
        # "Template Separator\n(You can make a copy of, or modify, this frame)"
        n650 = Unbundle By Name(w1653) -> ("Arduino ISS.Mega F3"=w1650:refnum<visa-resource-name>)
        n651 = while {
          shift-right: [w1666] -> w1651
          shift-left: w1652 -> [w1686]
          tunnel: w1650 -> [w1675]
          i -> [w1664]
          stop <- w1662 stop-if-true
          n652 = VISA Clear(VISA resource name=w1675, error in (no error)=w1686) -> (VISA resource name out=w1689:refnum<visa-resource-name>, error out=w1688:errorcluster)
          n653 = Equal?(x=w1664, y=3) -> (x = y?=w1661:bool)
          n654 = VISA Write(VISA resource name=w1689, write buffer="303/1", error in (no error)=w1688) -> (VISA resource name out=w1656:refnum<visa-resource-name>, error out=w1690:errorcluster)  [unwired: 1 out]
          n655 = call "Stall Data Flow.vim"("value in"=w1690, "milliseconds to wait"=u32 10000) -> ("value out"=w1677:errorcluster)  [unwired: 1 out]
          n656 = VISA Clear(VISA resource name=w1656, error in (no error)=w1677) -> (VISA resource name out=w1681:refnum<visa-resource-name>, error out=w1682:errorcluster)
          n657 = VISA Write(VISA resource name=w1681, write buffer="305", error in (no error)=w1682) -> (VISA resource name out=w1678:refnum<visa-resource-name>, error out=w1680:errorcluster)  [unwired: 1 out]
          n658 = call "Stall Data Flow.vim"("value in"=w1680, "milliseconds to wait"=u32 2005) -> ("value out"=w1679:errorcluster)  [unwired: 1 out]
          n659 = property class="Instr"(reference=w1678, error in=w1679) -> (reference out=w1674:refnum<visa-resource-name>, error out=w1673:errorcluster, "Serial Settings:Number of Bytes at Serial Port"=w1657:u32)
          n660 = Greater Than 0?(x=w1657) -> (x > 0?=w1676:bool)
          n661 = case shown="True" w1676 {
            selector: w1676 -> [w1693 _]
            tunnel: w1673 -> [w1694 w1706]
            tunnel: w1674 -> [w1692 w1705]
            tunnel: [w1694 w1697] -> w1665
            tunnel: [w1693 w1700] -> w1659
            tunnel: [w1692 w1696] -> w1667
            tunnel: w1657 -> [_ w1695]
            frame False {
            }
            frame True {
              n662 = VISA Read(VISA resource name=w1705, byte count=w1695, error in (no error)=w1706) -> (VISA resource name out=w1699:refnum<visa-resource-name>, read buffer=w1703:string, error out=w1698:errorcluster)  [unwired: 1 out]
              n663 = Match Pattern(string=w1703, regular expression=",") -> (before substring=w1702:string)  [unwired: 1 in, 3 out]
              n664 = Not Equal?(x="E", y=w1702) -> (x != y?=w1700:bool)
              n665 = case shown="True" w1700 {
                tunnel: w1699 -> [w1708 w1717]
                tunnel: w1698 -> [w1709 w1716]
                tunnel: [w1710 w1716] -> w1697
                tunnel: [w1707 w1717] -> w1696
                frame False {
                  n666 = VISA Clear(VISA resource name=w1708, error in (no error)=w1709) -> (VISA resource name out=w1714:refnum<visa-resource-name>, error out=w1713:errorcluster)
                  n667 = VISA Write(VISA resource name=w1714, write buffer="306", error in (no error)=w1713) -> (VISA resource name out=w1707:refnum<visa-resource-name>, error out=w1715:errorcluster)  [unwired: 1 out]
                  n668 = call "Stall Data Flow.vim"("value in"=w1715, "milliseconds to wait"=u32 3000) -> ("value out"=w1710:errorcluster)  [unwired: 1 out]
                }
                frame True {
                }
              }
            }
          }
          n669 = Not(x=w1659) -> (.not. x?=w1660:bool)
          n670 = And(x=w1660, y=w1661) -> (x .and. y?=w1658:bool)
          n671 = case shown="True" w1658 {
            frame False {
            }
            frame True {
              n672 = One Button Dialog(message="Phase 3\nAir system\nDidn't recover") -> ()  [unwired: 1 in, 1 out]
            }
          }
          n673 = VISA Clear(VISA resource name=w1667, error in (no error)=w1665) -> (VISA resource name out=w1671:refnum<visa-resource-name>, error out=w1670:errorcluster)
          n674 = VISA Write(VISA resource name=w1671, write buffer="304", error in (no error)=w1670) -> (error out=w1672:errorcluster)  [unwired: 2 out]
          n675 = Or(x=w1659, y=w1661) -> (x .or. y?=w1662:bool)
          n676 = call "Stall Data Flow.vim"("value in"=w1672, "milliseconds to wait"=u32 4000) -> ("value out"=w1666:errorcluster)  [unwired: 1 out]
        }
        n677 = call <vilib>:"Add State(s) to Queue__jki_lib_state_machine.vi"("State(s) in (\"\")"=w1655) -> ("States Out"=w1654:string)  [unwired: 14 in]
      }
      frame "Mega: Scan Barcodes" {
        # "Template Separator\n(You can make a copy of, or modify, this frame)"
        n678 = call "Ini_GetBarcodeString_2.0.vi"("error in (no error)"=w1723, "Data"=w1724) -> ("error out"=w1721:errorcluster, "F3 Status"=w1719:string, "Data 2"=w1722:T4)  [unwired: 2 in, 1 out]
        n679 = Concatenate Strings("UI: Status>>F3 Responce; " ("string"), w1719) -> (w1718:string)
        n680 = call <vilib>:"Add State(s) to Queue__jki_lib_state_machine.vi"("State(s) in Front (\"\")"=w1718, "State(s) in (\"\")"=w1726) -> ("States Out"=w1725:string)  [unwired: 13 in]
      }
      frame "Mega: Request status" {
        # "Template Separator\n(You can make a copy of, or modify, this frame)"
        n681 = Unbundle By Name(w1736) -> ("Auto Flush"=w1731:bool, "Arduino ISS.Phase3"=w1737:bool)
        n682 = case shown="True" w1737 {
          tunnel: w1739 -> [w1764 w1771]
          tunnel: [w1764 w1769] -> w1738
          tunnel: w1736 -> [w1763 w1772]
          tunnel: [w1763 w1768] -> w1729
          tunnel: [TRUE w1767] -> w1733
          tunnel: w1727 -> [_ w1770]
          tunnel: [w1761 w1766] -> w1735
          tunnel: [w1761 w1765] -> w1732
          frame False {
            w1761 = ""
            # "In case the system i used without a F3,\nthis value needs to be true, so that the function is not blocking anything else."
          }
          frame True {
            n683 = call "F3_Response.vi"("Data"=w1772, "Arguments"=w1770, "error constant"=w1771) -> ("Data 2"=w1768:T4, "Responce match"=w1767:bool, "Responce code"=w1765:string, "error out"=w1769:errorcluster, "UI: Status>>F3 responce"=w1766:string)
          }
        }
        n684 = case shown="True" w1733 {
          tunnel: w1735 -> [w1748 w1757]
          tunnel: [w1747 w1758] -> w1734
          tunnel: w1732 -> [w1741 _]
          tunnel: w1731 -> [w1746 _]
          tunnel: w1729 -> [w1744 w1760]
          tunnel: [w1740 w1760] -> w1730
          tunnel: w1728 -> [w1743 w1759]
          tunnel: w1727 -> [w1742 _]
          frame False {
            # "Responce was not a mach"
            n685 = case shown="True" w1746 {
              tunnel: ["UI: Status>>F3 responce don't match" ("f") w1752] -> w1745
              tunnel: w1744 -> [w1749 w1756]
              tunnel: w1743 -> [_ w1755]
              tunnel: w1742 -> [_ w1754]
              tunnel: w1741 -> [_ w1753]
              tunnel: [w1749 w1751] -> w1740
              frame False {
                # "Manual commands, so no need to interupt"
              }
              frame True {
                # "Auto flushing"
                n686 = call "F3_ErrorAndResponceHandler.vi"("Responce code"=w1753, "Arguments"=w1754, "State Que"=w1755, "Data"=w1756) -> ("State Que Out"=w1752:string, "Data Out"=w1751:T4)
              }
            }
            n687 = call <vilib>:"Add State(s) to Queue__jki_lib_state_machine.vi"("State(s) in Front (\"\")"=w1748, "State(s) in (\"\")"=w1745) -> ("States Out"=w1747:string)  [unwired: 13 in]
          }
          frame True {
            # "The Responce was a mach, No need for any action"
            n688 = call <vilib>:"Add State(s) to Queue__jki_lib_state_machine.vi"("State(s) in Front (\"\")"=w1757, "State(s) in (\"\")"=w1759) -> ("States Out"=w1758:string)  [unwired: 13 in]
          }
        }
      }
      frame "Mega: Request Barcodes" {
        # "Template Separator\n(You can make a copy of, or modify, this frame)"
        n689 = Unbundle By Name(w1775) -> ("Arduino ISS.Mega F3"=w1777:refnum<visa-resource-name>, "Arduino ISS.Phase3"=w1773:bool)
        n690 = case shown="True" w1773 {
          tunnel: w1777 -> [_ w1783]
          tunnel: w1776 -> [w1780 w1782]
          tunnel: [w1780 w1781] -> w1774
          frame False {
          }
          frame True {
            n691 = VISA Clear(VISA resource name=w1783, error in (no error)=w1782) -> (VISA resource name out=w1786:refnum<visa-resource-name>, error out=w1787:errorcluster)
            n692 = VISA Write(VISA resource name=w1786, write buffer="302", error in (no error)=w1787) -> (VISA resource name out=w1790:refnum<visa-resource-name>, error out=w1795:errorcluster)  [unwired: 1 out]
            n693 = call "Stall Data Flow.vim"("value in"=w1790, "milliseconds to wait"=u32 2001) -> ("value out"=w1789:refnum<visa-resource-name>)  [unwired: 1 out]
            n694 = property class="Instr"(reference=w1789, error in=w1795) -> (reference out=w1793:refnum<visa-resource-name>, error out=w1792:errorcluster, "Serial Settings:Number of Bytes at Serial Port"=w1794:u32)
            n695 = VISA Read(VISA resource name=w1793, byte count=w1794, error in (no error)=w1792) -> (read buffer=w1785:string, error out=w1784:errorcluster)  [unwired: 2 out]
            n696 = call "SaveBarcodeString.vi"("error in"=w1784, "String"=w1785) -> ("error out"=w1781:errorcluster)  [unwired: 3 in]
          }
        }
        n697 = call <vilib>:"Add State(s) to Queue__jki_lib_state_machine.vi"("State(s) in (\"\")"=w1779) -> ("States Out"=w1778:string)  [unwired: 14 in]
      }
      frame "Mega: Send Barcode" {
        # "Template Separator\n(You can make a copy of, or modify, this frame)"
        n698 = local read "Container barcode"() -> (w1798:string)
        n699 = Unbundle By Name(w1801) -> ("Arduino ISS.Barcode"=w1810:string, "Arduino ISS.Mega F3"=w1799:refnum<visa-resource-name>, "Auto Flush"=w1800:bool)
        n700 = Decimal String To Number(string=w1797) -> (number=w1796:i32)  [unwired: 2 in, 1 out]
        n701 = case shown="False" w1800 {
          tunnel: w1810 -> [_ _]
          tunnel: [w1817 w1823] -> w1805
          tunnel: [w1815 w1821] -> w1804
          tunnel: w1798 -> [_ w1822]
          tunnel: w1803 -> [w1814 w1821]
          tunnel: w1796 -> [w1813 _]
          frame False {
            n702 = Decrement(x=w1813) -> (x-1=w1816:i32)
            n703 = call "ContainerNumToBarcode.vi"("error in"=w1814, "Container num."=w1816) -> ("error out"=w1815:errorcluster, "Container barcode"=w1818:string)  [unwired: 5 in, 3 out]
            n704 = Concatenate Strings("303" ("write buffer"), "/" ("string"), w1818) -> (w1817:string)
          }
          frame True {
            n705 = Concatenate Strings("303" ("write buffer"), "/" ("string"), w1822) -> (w1823:string)
          }
        }
        n706 = VISA Clear(VISA resource name=w1799, error in (no error)=w1804) -> (VISA resource name out=w1808:refnum<visa-resource-name>, error out=w1807:errorcluster)
        n707 = VISA Write(VISA resource name=w1808, write buffer=w1805, error in (no error)=w1807) -> (error out=w1809:errorcluster)  [unwired: 2 out]
        n708 = call "Stall Data Flow.vim"("value in"=w1809, "milliseconds to wait"=u32 10000) -> ("value out"=w1802:errorcluster)  [unwired: 1 out]
        n709 = call <vilib>:"Add State(s) to Queue__jki_lib_state_machine.vi"("State(s) in (\"\")"=w1812) -> ("States Out"=w1811:string)  [unwired: 14 in]
      }
      frame "Mega: Return Home" {
        # "Template Separator\n(You can make a copy of, or modify, this frame)"
        n710 = Unbundle By Name(w1829) -> ("Arduino ISS.Mega F3"=w1830:refnum<visa-resource-name>, "Arduino ISS.Phase3"=w1826:bool)
        n711 = case shown="True" w1826 {
          tunnel: w1830 -> [_ w1836]
          tunnel: w1828 -> [w1833 w1835]
          tunnel: [w1833 w1834] -> w1827
          frame False {
          }
          frame True {
            n712 = VISA Clear(VISA resource name=w1836, error in (no error)=w1835) -> (VISA resource name out=w1840:refnum<visa-resource-name>, error out=w1841:errorcluster)
            n713 = VISA Write(VISA resource name=w1840, write buffer="304", error in (no error)=w1841) -> (error out=w1838:errorcluster)  [unwired: 2 out]
            n714 = call "Stall Data Flow.vim"("value in"=w1838, "milliseconds to wait"=u32 4000) -> ("value out"=w1834:errorcluster)  [unwired: 1 out]
          }
        }
        n715 = call <vilib>:"Add State(s) to Queue__jki_lib_state_machine.vi"("State(s) in (\"\")"=w1832) -> ("States Out"=w1831:string)  [unwired: 14 in]
      }
      frame "Mega: Clear error" {
        # "Template Separator\n(You can make a copy of, or modify, this frame)"
        n716 = Unbundle By Name(w1845) -> ("Arduino ISS.Mega F3"=w1847:refnum<visa-resource-name>, "Arduino ISS.Phase3"=w1843:bool)
        n717 = case shown="True" w1843 {
          tunnel: w1847 -> [_ w1853]
          tunnel: w1846 -> [w1850 w1852]
          tunnel: [w1850 w1851] -> w1844
          frame False {
          }
          frame True {
            n718 = VISA Clear(VISA resource name=w1853, error in (no error)=w1852) -> (VISA resource name out=w1855:refnum<visa-resource-name>, error out=w1856:errorcluster)
            n719 = VISA Write(VISA resource name=w1855, write buffer="306", error in (no error)=w1856) -> (error out=w1854:errorcluster)  [unwired: 2 out]
            n720 = call "Stall Data Flow.vim"("value in"=w1854, "milliseconds to wait"=u32 3000) -> ("value out"=w1851:errorcluster)  [unwired: 1 out]
          }
        }
        n721 = call <vilib>:"Add State(s) to Queue__jki_lib_state_machine.vi"("State(s) in Front (\"\")"="Mega: Return Home" ("State(s) in Front (\"\")"), "State(s) in (\"\")"=w1849) -> ("States Out"=w1848:string)  [unwired: 13 in]
      }
      frame "Mega: Uninitialize" {
        # "Template Separator\n(You can make a copy of, or modify, this frame)"
        n722 = Unbundle By Name(w1861) -> ("Arduino ISS.Mega F3"=w1862:refnum<visa-resource-name>, "Arduino ISS.Phase3"=w1863:bool)
        n723 = case shown="False" w1863 {
          tunnel: w1865 -> [w1868 w1875]
          tunnel: [w1868 w1874] -> w1864
          tunnel: w1862 -> [_ w1873]
          tunnel: w1861 -> [w1869 w1872]
          tunnel: [w1869 w1871] -> w1860
          tunnel: w1859 -> [_ w1870]
          frame False {
          }
          frame True {
            n724 = case shown="\"\", Default" w1870 {
              tunnel: w1875 -> [w1880 w1886]
              tunnel: [w1880 w1885] -> w1874
              tunnel: w1873 -> [_ w1884]
              tunnel: w1872 -> [w1879 w1883]
              tunnel: [w1878 w1882] -> w1871
              frame "", Default {
                w1877 = FALSE ("Arduino ISS.Phase3")
                n725 = Bundle By Name(cluster=w1879, "Arduino ISS.Mega F3"=refnum<visa-resource-name> refnum, "Arduino ISS.Phase3"=w1877) -> (w1878:T4)
                n726 = local write "Phase 3"(w1877) -> ()
              }
              frame "Exit" {
                w1881 = FALSE ("Arduino ISS.Phase3")
                n727 = Bundle By Name(cluster=w1883, "Arduino ISS.Phase3"=w1881) -> (w1882:T4)
                n728 = local write "Phase 3"(w1881) -> ()
                n729 = VISA Close(VISA resource name=w1884, error in (no error)=w1886) -> (error out=w1885:errorcluster)
              }
            }
          }
        }
        n730 = call <vilib>:"Add State(s) to Queue__jki_lib_state_machine.vi"("State(s) in (\"\")"=w1867) -> ("States Out"=w1866:string)  [unwired: 14 in]
      }
      frame "---------- Cam ----------" {
        # "Template Separator\n(You can make a copy of, or modify, this frame)"
        n731 = call <vilib>:"Add State(s) to Queue__jki_lib_state_machine.vi"("State(s) in (\"\")"=w1890) -> ("States Out"=w1889:string)  [unwired: 14 in]
      }
      frame "Cam: Initialize" {
        w1902 = IMAQdx_Camera_Control_Mode."Controller" ("Camera Control Mode")
        # "Template Separator\n(You can make a copy of, or modify, this frame)"
        n732 = call "Camera_ID_2.0.vi"("error in"=w1903, "Data"=w1904) -> ("error out"=w1891:errorcluster, "CAM2"=w1900:string, "CAM1"=w1901:string, "output cluster"=w1897:T4)  [unwired: 5 in]
        n733 = call <vilib>:"IMAQdx Open Camera.vi"("Camera Control Mode"=w1902, "error in"=w1891, "Session In"=w1900) -> ("error out"=w1894:errorcluster, "Session Out"=w1898:T5)  [unwired: 7 in]
        n734 = call <vilib>:"IMAQdx Open Camera.vi"("Camera Control Mode"=w1902, "error in"=w1891, "Session In"=w1901) -> ("error out"=w1895:errorcluster, "Session Out"=w1899:T5)  [unwired: 7 in]
        n735 = Merge Errors(w1895, w1894) -> (w1892:errorcluster)
        n736 = case shown="No Error" w1892 {
          tunnel: w1899 -> [w1911 w1925]
          tunnel: w1898 -> [w1908 w1923]
          tunnel: w1897 -> [w1912 w1916]
          tunnel: [w1910 w1915] -> w1896
          tunnel: w1895 -> [_ w1926]
          tunnel: w1894 -> [_ w1924]
          tunnel: ["UI: Status>>Cameras Initiated sucessfully\nData: Save Cam Id\nPump: Response>>Status\nCam: Calibration Pictures" w1921] -> w1893
          frame No Error {
            w1907 = TRUE ("Camera 1.Cam 1")
            n737 = Bundle By Name(cluster=w1912, "Camera 1.Camera1"=w1911, "Camera 1.Cam 1"=w1907, "Camera 2.Camera2"=w1908, "Camera 2.Cam 2"=w1907) -> (w1910:T4)
            "Cam 2" <- w1907
            "Cam 1" <- w1907
          }
          frame Error {
            n738 = case shown="No Error" w1924 {
              tunnel: w1923 -> [w1928 _]
              tunnel: [TRUE FALSE] -> w1913
              frame No Error {
                n739 = call <vilib>:"IMAQdx Close Camera.vi"("Session In"=w1928) -> ()  [unwired: 10 in, 1 out]
              }
              frame Error {
              }
            }
            n740 = case shown="No Error" w1926 {
              tunnel: w1925 -> [w1931 _]
              tunnel: [TRUE ("Camera 1") FALSE ("Camera 1")] -> w1914
              frame No Error {
                n741 = call <vilib>:"IMAQdx Close Camera.vi"("Session In"=w1931) -> ()  [unwired: 10 in, 1 out]
              }
              frame Error {
              }
            }
            n742 = Bundle By Name(cluster=w1916, "Camera 1.Cam 1"=w1914, "Camera 2.Cam 2"=w1913) -> (w1915:T4)
            n743 = local write "Cam 1"(w1914) -> ()
            n744 = local write "Cam 2"(w1913) -> ()
            n745 = Two Button Dialog(message="Cam Connection Failed", 2:"Retry" ("T button name (\"OK\")")) -> (T button?=w1919:bool)  [unwired: 1 in]
            n746 = Select(t="Uno: Cam Id request\nCam: Initialize", s=w1919, f="") -> (s? t:f=w1921:string)
          }
        }
        n747 = call <vilib>:"Add State(s) to Queue__jki_lib_state_machine.vi"("State(s) in Front (\"\")"=w1893, "State(s) in (\"\")"=w1906) -> ("States Out"=w1905:string)  [unwired: 13 in]
      }
      frame "Cam: Calibration Pictures" {
        # "Template Separator\n(You can make a copy of, or modify, this frame)"
        n748 = Unbundle By Name(w1942) -> ("Camera 1.Cam 1"=w1941:bool, "Camera 2.Cam 2"=w1940:bool)
        n749 = And(x=w1941, y=w1940) -> (x .and. y?=w1939:bool)
        n750 = case shown="True" w1939 {
          tunnel: [w1948 w1961] -> w1943
          tunnel: w1942 -> [w1948 w1960]
          tunnel: w1938 -> [w1947 w1958]
          tunnel: [w1947 w1955] -> w1937
          tunnel: [FALSE TRUE] -> w1933
          frame False {
            n751 = One Button Dialog(message="One or both cameras\nare missing.\nCould not start image captire.") -> ()  [unwired: 1 in, 1 out]
          }
          frame True {
            w1964 = TRUE ("Crop?")
            n752 = call "Calibration_Capture_2.0.vi"("Crop?"=FALSE, "Enum"=enum16{"Wide", "Cuvette", "Detect"}."Wide", "Data"=w1960) -> ("Image2"=w1969:T3, "Image1"=w1970:T3, "Data 2"=w1968:T4, "error out"=w1959:errorcluster)  [unwired: 3 in]
            n753 = local write "Camera 1 Detect"(w1970) -> ()
            n754 = local write "Camera 2 Detect"(w1969) -> ()
            n755 = call "Calibration_Capture_2.0.vi"("Detect Movement"=FALSE ("Crop?"), "Crop?"=TRUE, "Enum"=enum16{"Wide", "Cuvette", "Detect"}."Cuvette", "Data"=w1968) -> ("Image2"=w1962:T3, "Image1"=w1963:T3, "Data 2"=w1967:T4, "error out"=w1957:errorcluster)  [unwired: 2 in]
            n756 = local write "Camera 1 Binary"(w1963) -> ()
            n757 = local write "Camera 2 Binary"(w1962) -> ()
            n758 = call "Calibration_Capture_2.0.vi"("Detect Movement"=w1964, "Crop?"=w1964, "Enum"=enum16{"Wide", "Cuvette", "Detect"}."Detect", "Data"=w1967) -> ("Image2"=w1953:T3, "Image1"=w1954:T3, "Data 2"=w1961:T4, "error out"=w1956:errorcluster)  [unwired: 2 in]
            n759 = Merge Errors(w1959, w1957, w1956, w1958) -> (w1955:errorcluster)
            n760 = local write "Camera 1"(w1954) -> ()
            n761 = local write "Camera 2"(w1953) -> ()
          }
        }
        n762 = call-poly <vilib>:"Select State(s)__jki_lib_state_machine.vi"("State(s) if True (\"\")"=w1936, "Select"=w1933, "State(s) if False (\"\")"="" ("State(s) if False (\"\")")) -> ("States Out"=w1935:string)  [unwired: 12 in]
        n763 = call <vilib>:"Add State(s) to Queue__jki_lib_state_machine.vi"("State(s) in (\"\")"=w1935) -> ("States Out"=w1944:string)  [unwired: 14 in]
      }
      frame "Cam: Change Crop" {
        # "Template Separator\n(You can make a copy of, or modify, this frame)"
        n764 = call "Camera_Crop_Setup_2.0.vi"("error in (no error)"=w1973, "Data"=w1975) -> ("error out"=w1972:errorcluster, "output cluster"=w1974:T4)  [unwired: 1 in]
        n765 = call <vilib>:"Add State(s) to Queue__jki_lib_state_machine.vi"("State(s) in (\"\")"=w1977) -> ("States Out"=w1976:string)  [unwired: 14 in]
      }
      frame "Cam: Uninitialize" {
        # "Template Separator\n(You can make a copy of, or modify, this frame)"
        n766 = Unbundle By Name(w1983) -> ("Camera 1.Camera1"=w1984:T5, "Camera 1.Cam 1"=w1987:bool, "Camera 2.Camera2"=w1985:T5, "Camera 2.Cam 2"=w1986:bool)
        n767 = case shown="True" w1986 {
          tunnel: w1985 -> [_ w1993]
          tunnel: w1983 -> [w1991 w1999]
          tunnel: [w1991 w1998] -> w1982
          tunnel: w1980 -> [w1990 w1995]
          tunnel: [w1990 w1994] -> w1979
          frame False {
          }
          frame True {
            w1992 = FALSE ("Camera 2.Cam 2")
            n768 = Bundle By Name(cluster=w1999, "Camera 2.Cam 2"=w1992) -> (w1998:T4)
            n769 = call <vilib>:"IMAQdx Unconfigure Acquisition.vi"("error in"=w1995, "Session In"=w1993) -> ("error out"=w1997:errorcluster, "Session Out"=w1996:T5)  [unwired: 8 in]
            n770 = local write "Cam 2"(w1992) -> ()
            n771 = call <vilib>:"IMAQdx Close Camera.vi"("error in"=w1997, "Session In"=w1996) -> ("error out"=w1994:errorcluster)  [unwired: 9 in]
          }
        }
        n772 = case shown="True" w1987 {
          tunnel: w1984 -> [_ w2004]
          tunnel: w1982 -> [w2001 w2009]
          tunnel: [w2001 w2008] -> w1981
          tunnel: w1979 -> [w2000 w2005]
          tunnel: [w2000 w2003] -> w1978
          frame False {
          }
          frame True {
            w2002 = FALSE ("Camera 1.Cam 1")
            n773 = Bundle By Name(cluster=w2009, "Camera 1.Cam 1"=w2002) -> (w2008:T4)
            n774 = call <vilib>:"IMAQdx Unconfigure Acquisition.vi"("error in"=w2005, "Session In"=w2004) -> ("error out"=w2006:errorcluster, "Session Out"=w2007:T5)  [unwired: 8 in]
            n775 = local write "Cam 1"(w2002) -> ()
            n776 = call <vilib>:"IMAQdx Close Camera.vi"("error in"=w2006, "Session In"=w2007) -> ("error out"=w2003:errorcluster)  [unwired: 9 in]
          }
        }
        n777 = call <vilib>:"Add State(s) to Queue__jki_lib_state_machine.vi"("State(s) in (\"\")"=w1989) -> ("States Out"=w1988:string)  [unwired: 14 in]
      }
    }
    n778 = call <extravilib>:"Write.vi"("element"=w7) -> ("channel"=w9:T16)  [unwired: 1 out]
  }
  n779 = while {
    tunnel: w1 -> [w2010]
    stop <- w2014 stop-if-true
    # "Image Save"
    n780 = call <extravilib>:"Read.vi"("channel"=w2010) -> ("element"=w2012:T4)  [unwired: 1 in, 1 out]
    n781 = Unbundle By Name(w2012) -> ("Img_Capt"=w2015:bool, "Exit"=w2011:bool)
    n782 = case shown="False" w2015 {
      selector: w2015 -> [_ w2021]
      tunnel: [TRUE ("Last Image?") w2022] -> w2013
      tunnel: w2010 -> [_ w2023]
      tunnel: w2011 -> [_ w2020]
      frame False {
        n783 = local write "Save buffer"(T2 {"# elements in queue"=0, "# elements in queue"=0} ("Image Saving")) -> ()
        n784 = Wait (ms)(milliseconds to wait=u32 10) -> ()  [unwired: 1 out]
      }
      frame True {
        n785 = while {
          tunnel: w2023 -> [w2038]
          tunnel: [w2026] -> w2022
          shift-right: [FALSE] -> _
          shift-left: w2021 -> [w2036]
          tunnel: w2020 -> [w2035]
          stop <- w2026 stop-if-true
          n786 = call <extravilib>:"Read.vi"("channel"=w2038) -> ("element"=w2037:T4)  [unwired: 1 in, 1 out]
          n787 = call "Image_Save_Handler_2.0.vi"("first iteration"=w2036, "Data"=w2037, "Stop?"=w2035) -> ("Image Save 1"=→"Camera 1 Detect":T3, "Container num. Out"=w2024:i32, "Image Save 2"=→"Camera 2 Detect":T3, "Container barcode"=w2025:string, "Cam2_Stats"=→"Cam2_Stats":cluster{"Mean_Area":i32, "Img_Count":u32}, "Ready file created"=w2030:bool, "Cam1_Stats"=→"Cam1_Stats":cluster{"Mean_Area":i32, "Img_Count":u32}, "Queue size"=→"Save buffer":T2, "timeout"=→"Ready":bool, "Sample Name"=→"Sample Number":string, "Stop out"=w2026:bool)  [unwired: 13 in, 1 out]
          "Individual processed" <- w2030
          n788 = case shown="True" w2030 {
            tunnel: w2030 -> [_ w2042]
            tunnel: w2025 -> [_ w2041]
            tunnel: w2024 -> [_ w2040]
            frame False {
            }
            frame True {
              n789 = property on="Individual processed" class="Bool (strict)"("Val(Sgnl)"=w2042) -> ()  [unwired: 2 in, 2 out]
              "Container barcode" <- w2041
              "Container num. Out" <- w2040
            }
          }
        }
      }
    }
    n790 = And(x=w2013, y=w2011) -> (x .and. y?=w2014:bool)
    n791 = case shown="False" w2014 {
      frame False {
      }
      frame True {
        n792 = call "IMAQ Dispose"("All Images? (No)"=TRUE) -> ()  [unwired: 5 in, 1 out]
      }
    }
  }
  n793 = while {
    tunnel: w1 -> [w2047]
    tunnel: [w2045] -> w6
    stop <- w2049 stop-if-true
    # "Image handling - object detection"
    n794 = call <extravilib>:"Read.vi"("channel"=w2047) -> ("element"=w2044:T4)  [unwired: 1 in, 1 out]
    n795 = Unbundle By Name(w2044) -> ("Img_Capt"=w2046:bool, "Exit"=w2043:bool)
    n796 = case shown="False" w2046 {
      tunnel: [TRUE ("Last Image?") w2058] -> w2048
      tunnel: w2047 -> [_ w2059]
      tunnel: [w2052 w2057] -> w2045
      frame False {
        # "Image capture inactive"
        n797 = Bundle(TRUE, FALSE) -> (w2053:cluster{bool, bool})  [unwired: 1 in]
        n798 = call <extravilib>:"Write.vi"("element"=w2053) -> ("channel"=w2052:T17)  [unwired: 1 out]
        n799 = local write "Process buffer"(T2 {"# elements in queue"=0, "# elements in queue"=0} ("Image processing")) -> ()
        n800 = Wait (ms)(milliseconds to wait=u32 10) -> ()  [unwired: 1 out]
      }
      frame True {
        # "Image capture active"
        n801 = while "Save image" {
          tunnel: w2059 -> [w2068]
          tunnel: [w2064] -> w2058
          tunnel: [w2066] -> w2057
          stop <- w2064 stop-if-true
          # "Image Processing"
          n802 = call <extravilib>:"Read.vi"("channel"=w2068) -> ("element"=w2067:T4)  [unwired: 1 in, 1 out]
          n803 = call "Image_Processing_Queue_2.0.vi"("Data"=w2067) -> ("Status"=w2066:T17, "Process queue"=→"Process buffer":T2, "Last Image?"=w2064:bool, "Image 1"=→"Camera 1":T3, "Image 2"=→"Camera 2":T3, "Binary 1"=→"Camera 1 Binary":T3, "Binary 2"=→"Camera 2 Binary":T3)  [unwired: 9 in, 3 out]
        }
      }
    }
    n804 = And(x=w2048, y=w2043) -> (x .and. y?=w2049:bool)
  }
  n805 = while {
    tunnel: w1 -> [w2071]
    tunnel: w6 -> [w2075]
    stop <- w2069 stop-if-true
    # "Camera Handler"
    n806 = call <extravilib>:"Read.vi"("channel"=w2075) -> ("element"=w2074:cluster{bool, bool})  [unwired: 1 in, 1 out]
    n807 = call <extravilib>:"Read.vi"("channel"=w2071) -> ("element"=w2070:T4)  [unwired: 1 in, 1 out]
    n808 = Unbundle(w2074) -> (w2072:bool, w2073:bool)
    n809 = Unbundle By Name(w2070) -> ("Img_Capt"=w2077:bool, "Exit"=w2069:bool)
    n810 = Not(x=w2073) -> (.not. x?=w2078:bool)
    n811 = And(x=w2078, y=w2077) -> (x .and. y?=w2076:bool)
    n812 = case shown="False" w2076 {
      tunnel: w2070 -> [_ w2081]
      tunnel: w2072 -> [_ w2082]
      frame False {
        # "Empty Case\nImage Capture currently inactive."
        n813 = local write "Framerate"(0.0 ("Framerate")) -> ()
        n814 = Wait (ms)(milliseconds to wait=u32 20) -> ()  [unwired: 1 out]
      }
      frame True {
        # "Capture Image\nImage Capture currently active, transmitting data."
        n815 = call "Image_Snap_Dual_2.0.vi"("Data"=w2081, "Detect Movement"=w2082) -> ("Framerate"=→"Framerate":i32)  [unwired: 6 in, 3 out]
      }
    }
  }
